vi "Position_TOTAL_R21.vi"(5 "Distance Between \nCameras  (*unit)":sgl=2.5) -> (12 "dX, dY\nLeft Cam":cluster{"X":sgl[], "Y":sgl[]}={"X"=[-5.750775, -4.1849813, -3.081379, -2.0098581, 0.0], "Y"=[7.9585915, 7.9595685, 7.960258, 7.960927, 0.0]}, 13 "Position Valid":bool=TRUE, 14 "Left Camera Real Coordinates":cluster{"X":sgl, "Y":sgl}={"X"=7.9602513, "Y"=5.592073}, 16 "dX, dY\nRight Cam":cluster{"X":sgl[], "Y":sgl[]}={"X"=[-7.3032045, -5.737411, -4.6338086, -3.5622878, -1.5524296], "Y"=[7.2714148, 7.2723923, 7.2730813, 7.273751, -0.68717635]}, 18 "Robot Coordinates":cluster{"X":sgl, "Y":sgl}={"X"=7.616663, "Y"=6.3682876}, 19 "Orietnation\n(current)":sgl=-23.843685 format="%#_13g")   [LabVIEW 2015]
uses:
  <vilib>/Analysis/coordinate.llb/2D Cartesian Coordinate Rotation (Array).vi
  <vilib>/myRIO/Common/Instrument Driver Framework/myRIO v1.0/DIO/vis/myRIO v1.0 Close DIO.vi
  <vilib>/myRIO/Common/Instrument Driver Framework/myRIO v1.0/DIO/vis/myRIO v1.0 Unreserve DIO.vi
  <vilib>/myRIO/Common/Instrument Driver Framework/myRIO v1.0/DIO/vis/myRIO v1.0 Build MUX Configuration DIO.vi
  <vilib>/myRIO/Common/Instrument Driver Framework/myRIO v1.0/Resource Manager/vis/myRIO v1.0 Unreserve Channel List.vi
  <vilib>/myRIO/Common/Instrument Driver Framework/myRIO v1.0/Resource Manager/vis/myRIO v1.0 Create Configuration List.vi
  <vilib>/myRIO/Common/Instrument Driver Framework/myRIO v1.0/Resource Manager/vis/myRIO v1.0 Unreserve Channel.vi
  <vilib>/myRIO/Common/Instrument Driver Framework/myRIO v1.0/Resource Manager/vis/myRIO v1.0 Build Mutex Name.vi
  <vilib>/Instr/_visa.llb/VISA Configure Serial Port (Instr).vi
  <vilib>/myRIO/Common/Instrument Driver Framework/myRIO v1.0/DIO/vis/myRIO v1.0 Shutdown DIO.vi
  <vilib>/Utility/error.llb/Error Cluster From Error Code.vi
  <vilib>/myRIO/Common/Instrument Driver Framework/myRIO v1.0/Resource Manager/vis/myRIO v1.0 Configure IO.vi
  <vilib>/myRIO/Common/Instrument Driver Framework/Utilities/vis/Configuration Manager.vi
  <vilib>/myRIO/Common/Instrument Driver Framework/Utilities/vis/IO Manager.vi
  <vilib>/myRIO/Common/Instrument Driver Framework/myRIO v1.0/myRIO v1.0 Close.vi
  <vilib>/Analysis/NI_AALPro.lvlib
  <vilib>/myRIO/Instrument Drivers/Onboard IO/DIO/DIO.lvlib
panel:
  out "Scale Based\nWeight":sgl format="%#_13g"
  in  "Triangle Based\nWeight":sgl=0.4 format="%#_13g"
  out "Current Cam State - R":T1(ring)=enum."Normal - 5"
  out "Current Cam State - L":T1(ring)=enum."Normal - 5"
  out "Valid Beacon Sets_":bool[](array[boolean])=[TRUE, TRUE, TRUE, TRUE, FALSE]
  in  "Distance Threshold\nRef Triangles (*unit)":sgl=30.0
  out "dA2 4":sgl=9.6935425 format="%#_13g"
  out "dA2 2":sgl=9.6935425 format="%#_13g"
  out "dA2 3":sgl=9.6935425 format="%#_13g"
  out "Beacon Scales - Left":sgl[](array[numeric])=[76.306, 116.841255, 157.35043, 195.67218, 0.0]
  out "Beacon Scales - Right":sgl[](array[numeric])=[76.306, 116.841255, 157.35043, 195.67218, 0.0]
  in  "New Orientation \nThreshold":sgl=10.0
  in  "Moving Average\nWindow Length":u8=2
  out "Current Recovery State -L":enum16{"Generic Sweep", "Recovery Search"}(ring)=enum."Recovery Search"
  out "Current Move Delta - L 2":u16
  out "Next Recovery State - Left":enum16{"Generic Sweep", "Recovery Search"}(ring)=enum."Recovery Search"
  out "Next Recovery State - Right":enum16{"Generic Sweep", "Recovery Search"}(ring)=enum."Recovery Search"
  out "Current Recovery State - Right":enum16{"Generic Sweep", "Recovery Search"}(ring)=enum."Recovery Search"
  in  "Initial Recovery State  - Right":enum16{"Generic Sweep", "Recovery Search"}(ring)=enum."Recovery Search"
  in  "Initial Recovery State - L":enum16{"Generic Sweep", "Recovery Search"}(ring)=enum."Recovery Search"
  out "Next Tracking State - Right":enum16{"Track", "Reactive Predict", ""}(ring)
  out "Current Tracking State - Right 2":enum16{"Track", "Reactive Predict", ""}(ring)
  in  "Initial Tracking State - Right":enum16{"Track", "Reactive Predict", ""}(ring)
  out "Last Track Angle - R":sgl=98.61328
  out "Next Tracking State - Left":enum16{"Track", "Reactive Predict", ""}(ring)
  in  "Initial Tracking State - Left":enum16{"Track", "Reactive Predict", ""}(ring)
  out "Current Tracking State - Left":enum16{"Track", "Reactive Predict", ""}(ring)
  in  "Timeout to \nEnable Reactive Predict":u16=5
  out "Tracking Timeout\nCount - R":i32
  in  "Tracking Timeout\nThreshold":i32=10
  out "Tracking Timeout\nCount - L":i32
  in  "Search Direction - in - Right":bool=TRUE
  out "Next Main State - Right":T2(ring)=enum."Tracking"
  in  "Recovery Search\nDirection - R":bool
  out "Recovery Mode Count in Right":i32
  out "Frames Processed\nCount - in Right":i32
  out "Recovery Search\nmove Count - Right":u16
  out "Recovery Search\nAttempt Count - Right":u16
  in  "Mounting Offset - Right":sgl=45.0
  in  "Tracking Angle - Right":sgl=98.60307
  in  "Current Servo Position\n- Right":u16
  out "New Data  Flag\nRight Servo":bool
  in  "Track Angle Valid  - Right":bool=TRUE
  out "Current Main State - Right":T2(ring)=enum."Tracking"
  in  "Initial Main State- Right":T2(ring)
  in  "Recovery Search\nDirection - L 2":bool
  in  "Max Recovery Count\n(Recovery Search) 2":u16
  in  "Max Recovery\nSearch Attempts 2":u16
  in  "Image Lock - Right 2":bool
  out "Last Track Angle - L":sgl=87.24609
  in  "Recovery Search\nDirection - L":bool=TRUE
  out "Next Main State - Left":T2(ring)=enum."Tracking"
  out "Current Move Delta - L":u16
  in  "Max Recovery Count\n(Recovery Search)":u16=10
  in  "Max Recovery\nSearch Attempts":u16=3
  out "Recovery Search\nAttempt Count - in - L":u16
  out "Recovery Search\nmove Count - in - L":u16
  in  "Image Lock - Right":bool=TRUE
  out "Recovery Mode Count - in Left":u16
  in  "Middle Beacon\nCoordinates":cluster{"X":sgl, "Y":sgl}={"X"=0.0, "Y"=2.5}
  in  "Min Num Frames\nper Search":i32=2
  in  "Wait Tick Threshold":i32=10
  out "Frames Processed\nCount - in -L":i32
  in  "Maximum Move \nServo Threshold":i16=300
  in  "Minimum Delta \nServo Threshold":i16=3
  in  "Mounting Offset - Left":sgl=-45.0
  in  "Search Step Size":u16=50
  in  "Search Direction - in - L":bool
  in  "Current Servo Position\n- Left":u16
  in  "Tracking Angle - Left":sgl=87.25689
  out "New Data  Flag\nLeft Servo":bool
  in  "Track Angle Valid - Left":bool=TRUE
  in  "Image Lock - Left":bool=TRUE
  in  "Initial Main State - Left":T2(ring)
  out "Current Main State - Left":T2(ring)=enum."Tracking"
  in  "Position Calc\nTimer":u32=100 caption="Position Calc Timer"
  in  "Fetch Input\n(mSec)":u32=20 caption="Update Camera Input\n(mSec)"
  out "Right Data\nInput Flag\n- Internal":bool=TRUE
  in  "Position Calc\nReady":bool
  out "This Servo \nAngle - Right":sgl=98.90625
  in  "Beacon Angles -R":sgl[](array[numeric])=[111.28093, 105.355774, 98.60307, 92.04714, 103.90625]
  in  "Beacon Angles - L":sgl[](array[numeric])=[101.98467, 94.59042, 87.25689, 80.30646, 91.66016]
  in  "Valid Angles -R":bool[](array[boolean])=[TRUE, TRUE, TRUE, TRUE, FALSE]
  in  "Valid Angles - L":bool[](array[boolean])=[TRUE, TRUE, TRUE, TRUE, FALSE]
  out "Left Data\nInput Flag\n- Internal":bool
  in  "Check Shared Var Timer":u32=50 caption="Main Loop\n Timer (ms)"
  out "Left_Flag 2":bool
  out "Right_Flag 2":bool
  out "Beacons Found\n- Left (Bool Array) 2":bool[](array[boolean])=[TRUE, TRUE, TRUE, TRUE, FALSE]
  out "LEFT Beacon Coord - X px (IN) 2":sgl[](array[numeric])=[76.306, 116.841255, 157.35043, 195.67218, 0.0]
  out "LEFT Beacon Position - Y px (IN) 2":sgl[](array[numeric])=[154.30304, 148.59094, 148.39949, 146.94655, 0.0]
  out "This Servo \nAngle - Left":sgl=86.66016
  in  "Compliance Slope":u8=128
  out "deltaMoveServo\n- R":i16
  out "Move Respond - R":bool
  out "Move Respond - L":bool
  out "Last Position":cluster{"X":sgl, "Y":sgl}={"X"=7.6261, "Y"=6.350474}
  out "Last Orientation":sgl=-23.876373
  in  "Distance\nBetween Beacons \n- Tolerance":sgl=0.35 format="%#_13g"
  in  "Distance\nBetween Beacons":sgl=1.0 format="%#_13g"
  out "dT":dbl=143.499
  out "Position Valid\nHistory":bool[](array[boolean])=[TRUE, FALSE, FALSE, TRUE, TRUE, FALSE, TRUE, TRUE, TRUE, TRUE, TRUE, TRUE, FALSE, TRUE, FALSE]
  out "Orientation\nHistory":sgl[](array[numeric])=[-23.876373, 0.0, 0.0, -23.938759, -24.0458, 0.0, -23.14014, -22.504314, -22.596928, -22.90728, -23.237453, -23.75214, 0.0, -23.808718, 0.0]
  out "Robot Coordinates\nHistory":cluster{sgl, sgl}[](array[cluster])=[{7.6261, 6.350474}, {0.0, 0.0}, {0.0, 0.0}, {7.63815, 6.33973}, {7.6316156, 6.322055}, {0.0, 0.0}, {7.6863523, 6.2558875}, {7.688662, 6.2228284}, {7.6736236, 6.2455945}, {7.6880507, 6.2819676}, {7.6893277, 6.3140097}, {7.668109, 6.3330927}, {0.0, 0.0}, {7.6506357, 6.3142757}, {0.0, 0.0}]
  in  "New Position \nThreshold":sgl=1.5
  out "Orientation Avgd":sgl=-23.876373
  in  "History Size":u8=15
  in  "Max Y (arena)":sgl=15.0
  in  "Max X (arena)":sgl=35.0
  in  "New Position\nWeight":sgl=0.7 format="%#_13g"
  in  "Max Std Dev (3)":sgl=0.2 format="%#_13g"
  in  "Max Std Dev (4)":sgl=0.2 format="%#_13g"
  out "Post Filtering\n- Valid Beacons":bool[](array[boolean])=[FALSE, TRUE, TRUE, TRUE, FALSE]
  out "Robot Coordinates - Avgd":cluster{"X":sgl, "Y":sgl}={"X"=7.6261, "Y"=6.350474}
  out "Real Position in Course 2":cluster{"X":dbl[], "Y":dbl[]}(graph)={"X"=[7.626100046018056], "Y"=[6.35047366782369]}
  out "Position \nLock Status":bool=TRUE
  out "Right Camera Real Coordinate":cluster{"X":sgl, "Y":sgl}={"X"=7.2730746, "Y"=7.1445026}
  out "deltaMoveServo\n- L":i16
  in  "Search Step Size\n(deg)":sgl=15.0 format="%#_13g"
  out "Beacons Found\n- Right (Bool Array)":bool[](array[boolean])=[TRUE, TRUE, TRUE, TRUE, FALSE]
  out "RIGHT Beacon Position - Y px (IN)":sgl[](array[numeric])=[153.02994, 149.48933, 150.4864, 150.33003, 0.0]
  out "RIGHT Beacon Coord - X px (IN)":sgl[](array[numeric])=[91.3685, 123.99656, 161.27843, 197.4523, 0.0]
  in  "Right Servo\nID":string="\u0001"
  in  "Servo Comm\nWait Time - (ms)":i32
  in  "Left Servo\nID":string="\u0000"
  out "dT - Comm Loop":u32=19
  in  "Servo Comm\nLoop Time (ms)":i32=20
  in  "close comms":bool
  in  "Max Read\nTx Attempts":u8=3
  in  "Max Write\nTx Attempts":u8=3
  out "Current R (10bit)":u16=696
  out "Servo Moving - R":bool
  out "Servo Moving - L":bool
  out "Current L (10bit)":u16=347
  in  "SERVO ENABLE":bool=TRUE
  out "Move Servo - L":bool
  out "Move Servo - R":bool
  in  "Servo Goal Position\n - Right":u16=695
  in  "Move Servo\nThreshold (deg)":sgl=2.0 format="%#_13g"
  in  "Servo Algorithm\nCycle Time(ms)":i32=25
  in  "Servo Goal Position\n - Left":u16=349
  in  "Current Angle\n - Left (internal)":sgl=86.66016
  in  "Current Angle\n - Right (internal)":sgl=98.90625
  in  "stop":bool
  in  "Num of Beacons (Total)":i8=5
  out "Angle to Pixel Ratios":T3={"Angle to Pixel\nRatio - Horizontal"=0.18125, "Angle to Pixel\nRatio - Vertical"=0.1875} {"Angle to Pixel\nRatio - Vertical" format="%#_13g"; "Angle to Pixel\nRatio - Horizontal" format="%#_13g"}
  in  "Cam AOV Vertical (deg)":sgl=45.0
  in  "Cam AOV Horizontal (deg)":sgl=58.0
  in  "Image Height (px)":sgl=240.0
  in  "Image Width (px)":sgl=320.0
  out "Beacon Coordinates - Left Image":T4={"Beacon Position - X px"=[76.306, 116.841255, 157.35043, 195.67218, 0.0], "Beacon Position - Y px"=[154.30304, 148.59094, 148.39949, 146.94655, 0.0]}
  out "Beacon Coordinates - Right Image":T4={"Beacon Position - X px"=[91.3685, 123.99656, 161.27843, 197.4523, 0.0], "Beacon Position - Y px"=[153.02994, 149.48933, 150.4864, 150.33003, 0.0]}
  out "Distance to LBF":sgl[](array[numeric])=[0.024284193, 0.015691843, 0.008273765, 0.028971607, 0.03291407]
  out "Local Coordinates - Calculated":cluster{sgl[], sgl[]}(graph)={[-2.0384164, -0.70265853, 0.4090246, 1.3811935, 0.0], [9.602626, 8.751521, 8.536832, 8.085801, 0.0]}
  out "Local Coordinates - Rotated":cluster{dbl[], dbl[]}(graph)={[1.5524295802029098, -5.750774735805926, -4.1849814062260675, -3.0813788557258652, -2.009858210562305, 0.0], [0.6871763361707266, 7.9585912385832795, 7.959568450875426, 7.960257859242679, 7.960927027680405, 0.0]}
  out "All Object Coordinates \n- Local - Rotated":cluster{"X":sgl[], "Y":sgl[]}={"X"=[1.5524296, -5.750775, -4.1849813, -3.081379, -2.0098581, 0.0], "Y"=[0.68717635, 7.9585915, 7.9595685, 7.960258, 7.960927, 0.0]}
  out "Local Coordinates - Normalized":cluster{sgl[], dbl[]}(graph)={[1.6977187, -2.0372734, -0.60508364, 0.4043527, 1.3844445, 0.0], [0.0, 9.605212211608887, 8.972328186035156, 8.526259422302246, 8.093157768249512, 0.0]}
  in  "Max Std Dev (5)":sgl=0.2 format="%#_13g"
  out "All Object Coordinates \n- Local":cluster{"X":sgl[], "Y":sgl[]}={"X"=[1.6977187, -2.0372734, -0.60508364, 0.4043527, 1.3844445, 0.0], "Y"=[0.0, 9.605212, 8.972328, 8.526259, 8.093158, 0.0]}
  out "LOCAL\nBeacon Coordinates\nRelative to Robot":cluster{"dX_beacon":sgl[], "dY_beacon":sgl[]}={"dX_beacon"=[-2.0384164, -0.70265853, 0.4090246, 1.3811935, 0.0], "dY_beacon"=[9.602626, 8.751521, 8.536832, 8.085801, 0.0]}
  in  "Real Beacon\n - Coordinates":cluster{"X":dbl[], "Y":dbl[]}={"X"=[0.0, 0.0, 0.0, 0.0, 0.0, 0.0], "Y"=[0.5, 1.5, 2.5, 3.5, 4.5, 0.0]}
  # "POSITION CALCULATION VARIABLES"
  # "OUTPUT VALUES"
  # "CONFIG VALUES"
  # "FILTER CONFIG VALUES"
  # "FEEDBACK INPUT VALUES"
  # "INPUT VALUES"
  # "INTERMEDIATE VALUES"
  # "IMAGE TO ANGLE VARIABLES"
  # "VISION PROCESSEING INPUTS"
  # "Use moving average for previous orientation thresholds"
  # "INPUTS"
  # "CONFIG"
  # "OUTPUT VALUES"
  # "*********************"
  # "unfiltered"
  # "NEW FILTER VALS"
  # "Inter Beacon Distance Filtering"
  # "MOVING AVERAGE\nVARIABLES"
  # "DISTANCE SOURCE WEIGHT"
  # "SERVO CONTROL VARIABLES"
  # "SERVO CONTROL VARIABLES"
  # "CONFIG"
  # "SHARED VARIABLE INPUTS"
  # "LOCAL VARIABLE INPUTS"
  # "INTERNRAL VARIABLES"
  # "SEARCH ROUTINE VARIABLES"
  # "MISC"
  # "SERVO IDs"
  # "CONTROL DELAYS"
  # "COMM LOOP DELAY"
  # "COMM PROTOCOL"
  # "SETTINGS"
  # "Make function of distance^^"
  # "**** only left side starts search\nat previously known good angle"
  # "LEFT SERVO"
  # "RIGHT SERVO"
  # "Main State Machine"
  # "Recovery State Machine"
  # "Current Track Angle Inputs"
  # "Servo Status Inputs"
  # "Main State Machine Inputs"
  # "Recovery State Machine Inputs"
  # "Current Track Angle Inputs"
  # "Servo Status Inputs"
  # "Recovery State Machine Feedback"
  # "Tracking State Machine Inputs"
  # "Tracking State Machine Inputs"
  # "NOTE: Must be 1 bigger than amount of beacons"
  # "NOTE: Must be 1 bigger than amount of beacons"
types:
  T1 = enum16{"Sub - 2", "Sub - 3", "Sub - 4", "Normal - 5"}
  T2 = enum16{"Start Up Search", "Tracking", "Recovery Mode", ""}
  T3 = cluster{"Angle to Pixel\nRatio - Horizontal":sgl, "Angle to Pixel\nRatio - Vertical":sgl}
  T4 = cluster{"Beacon Position - X px":sgl[], "Beacon Position - Y px":sgl[]}
  T5 = cluster{"Tracking Coordinates":cluster{"X":dbl, "Y":dbl}, "Current Valid":bool, "Current State - Out":enum16{"Sub - 2", "Sub - 3", "Sub - 4", "Normal - 5"}}
  T6 = cluster{"Array of Double":dbl[], "Array of Double":dbl[]}
  T7 = typedef "DIO.lvlib/DIO Reference.ctl" = cluster{"myRIO Reference":T8, "DIO Channels List":T12}
  T8 = typedef "myRIO Generic Hardware Reference.ctl" = cluster{"myRIO Model":T9, "myRIO Hardware Reference":T10}
  T9 = typedef "Hardware Version Enum.ctl" = enum16{"Unknown", "myRIO-1900", "myRIO-1950", "roboRIO"}
  T10 = typedef "myRIO v1.0 Reference.ctl" = cluster{"Generic FPGA Reference":T11, "Allow multiple opens":bool}
  T11 = typedef "Generic FPGA Reference.ctl" = refnum<k20>
  T12 = typedef "DIO Channels List.ctl" = T13[]
  T13 = typedef "DIO Channels Enum.ctl" = enum16{"Not Connected", "C/DIO0", "C/DIO1", "C/DIO2", "C/DIO3", "C/DIO4", "C/DIO5", "C/DIO6", "C/DIO7", "A/DIO0", "A/DIO1", "A/DIO2", "A/DIO3", "A/DIO4", "A/DIO5", "A/DIO6", "A/DIO7", "A/DIO8", "A/DIO9", "A/DIO10", "A/DIO11", "A/DIO12", "A/DIO13", "A/DIO14", "A/DIO15", "B/DIO0", "B/DIO1", "B/DIO2", "B/DIO3", "B/DIO4", "B/DIO5", "B/DIO6", "B/DIO7", "B/DIO8", "B/DIO9", "B/DIO10", "B/DIO11", "B/DIO12", "B/DIO13", "B/DIO14", "B/DIO15", "LED0", "LED1", "LED2", "LED3", "Button0", "DIO/DIO0", "DIO/DIO1", "DIO/DIO2", "DIO/DIO3", "DIO/DIO4", "DIO/DIO5", "DIO/DIO6", "DIO/DIO7", "DIO/DIO8", "DIO/DIO9", "SPI/CS0", "SPI/CS1", "SPI/CS2", "SPI/CS3", "LED RADIO (Green)", "LED RADIO (Red)", "LED COMM (Green)", "LED COMM (Red)", "LED MODE (Green)", "LED MODE (Red)"}
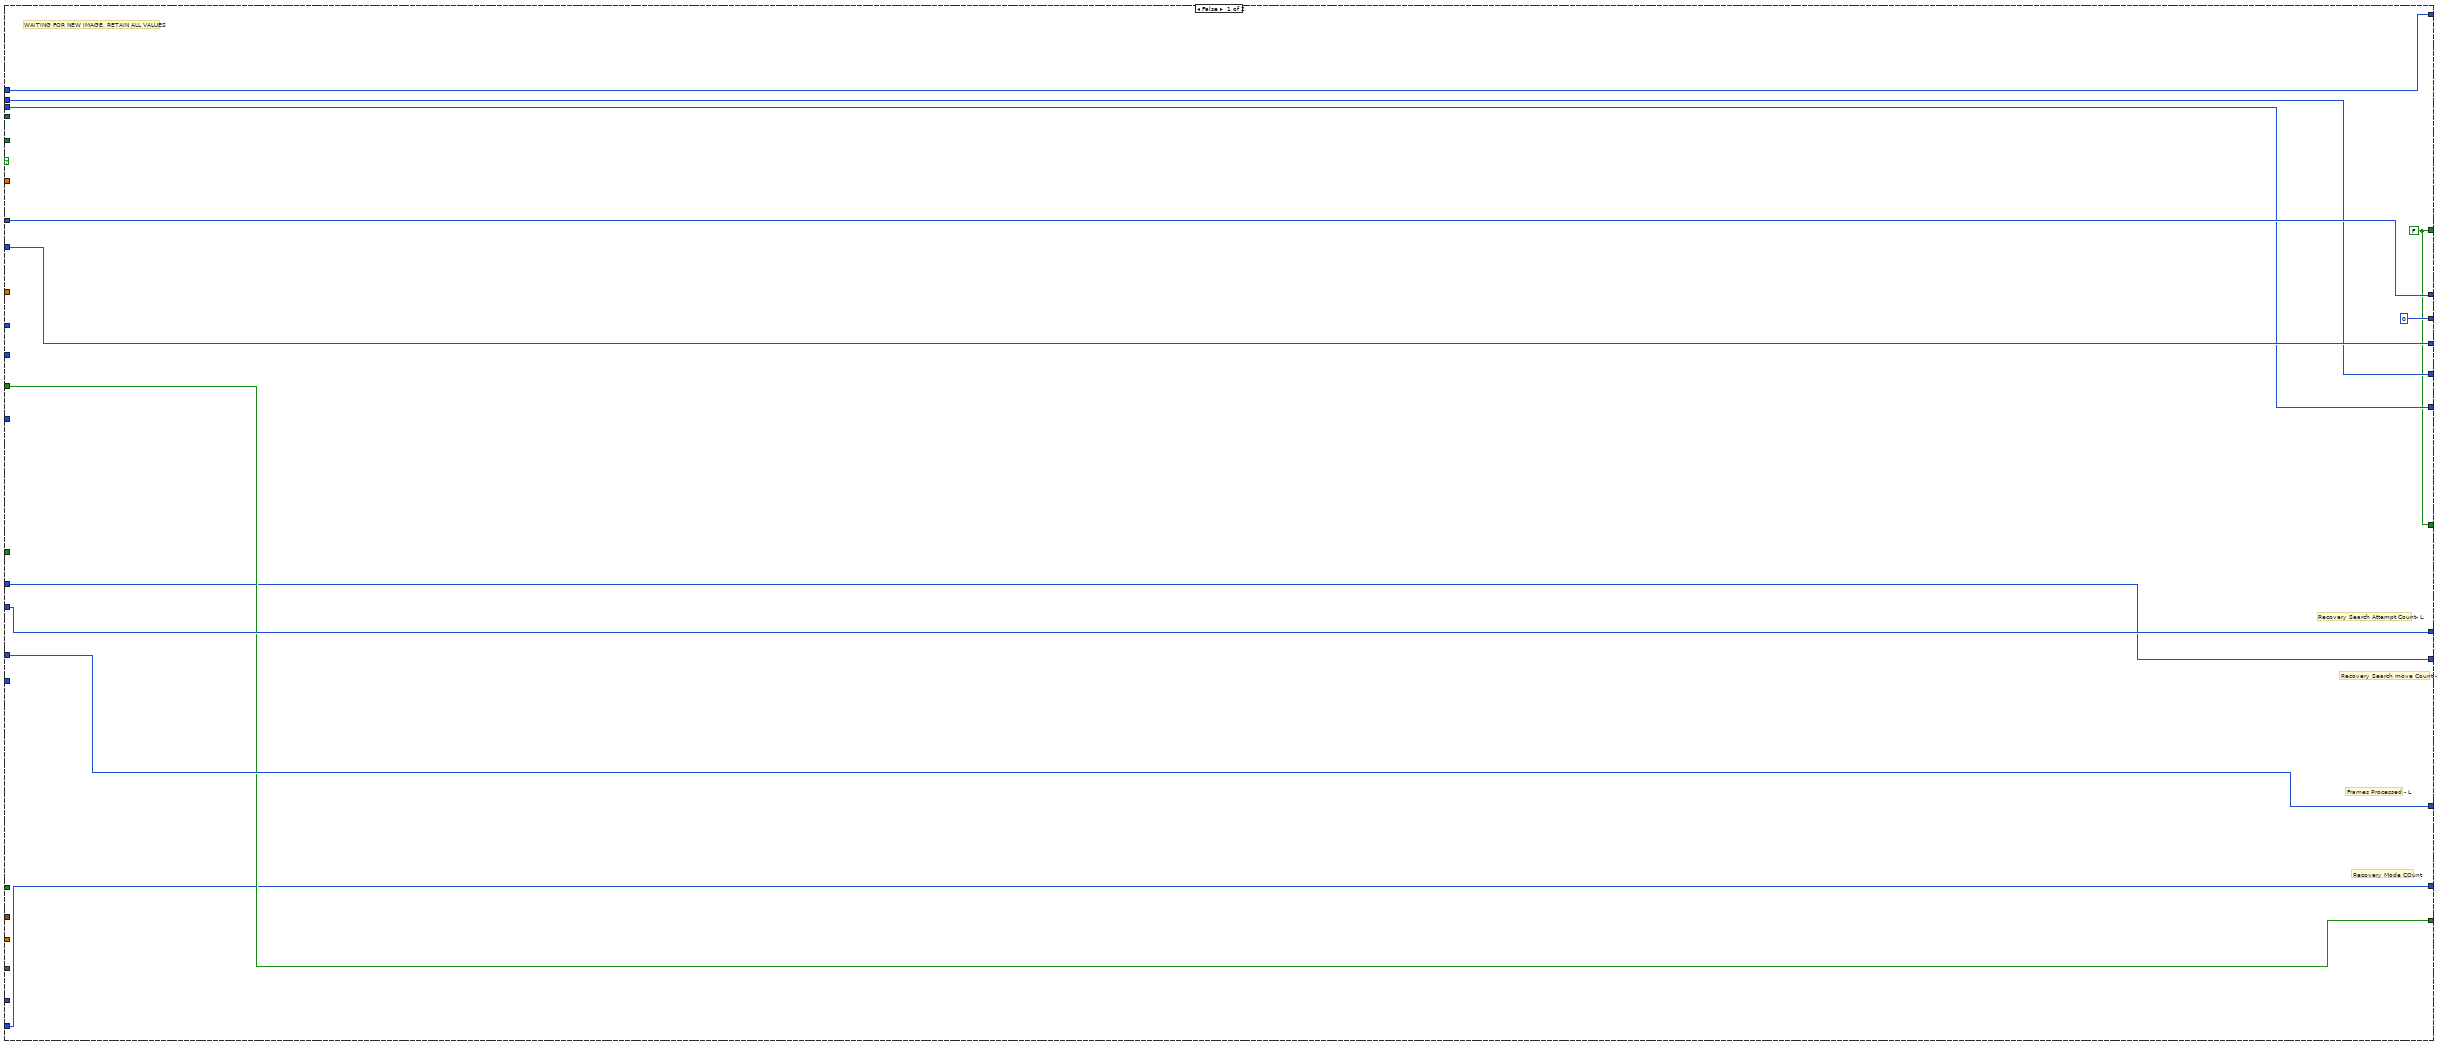
[diagram p2: hidden frame]
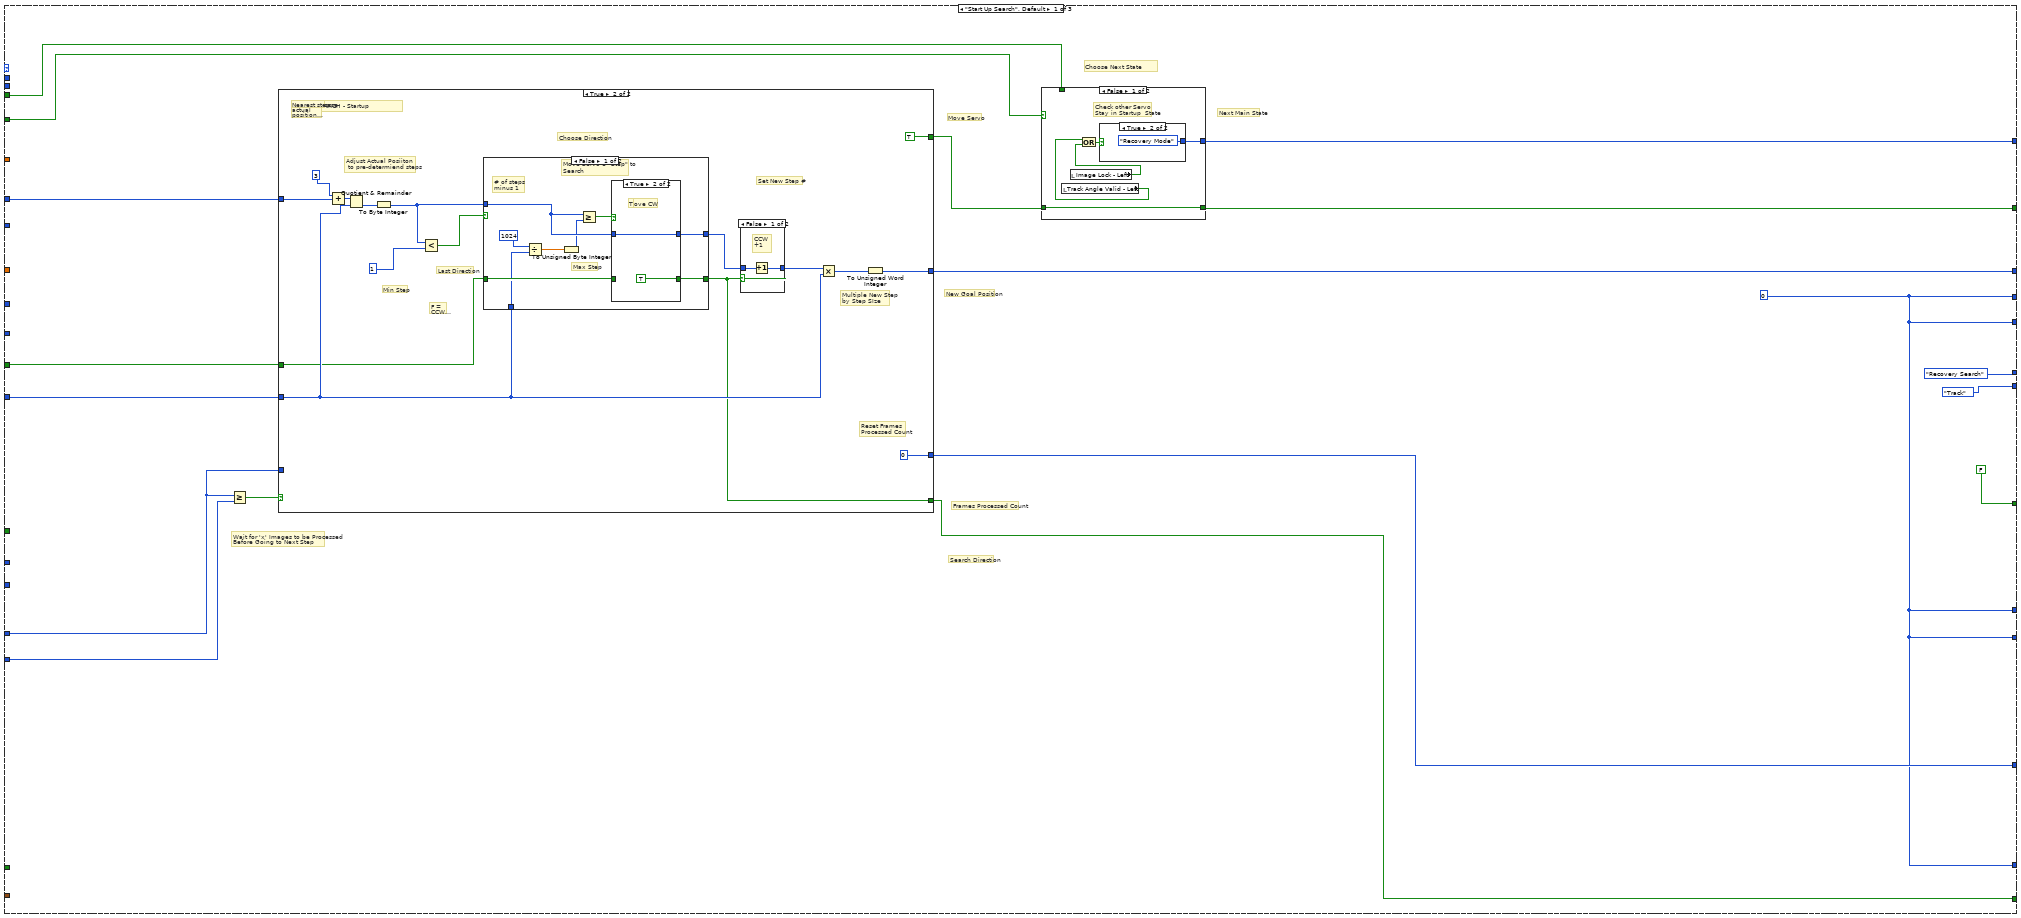
[diagram p3: hidden frame]
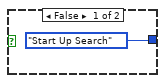
[diagram p4: hidden frame]
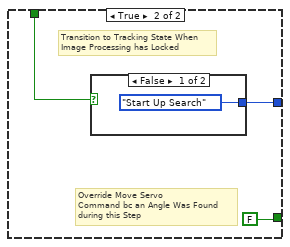
[diagram p5: hidden frame]
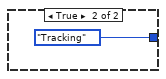
[diagram p6: hidden frame]
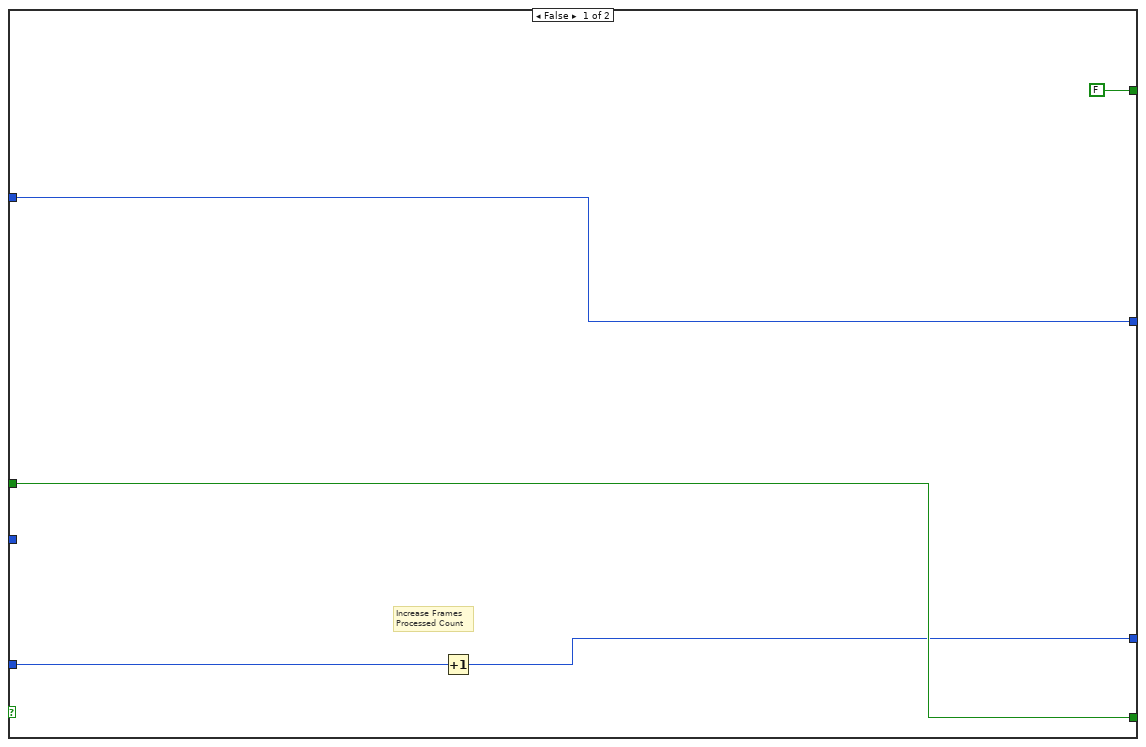
[diagram p7: hidden frame]
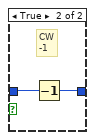
[diagram p8: hidden frame]
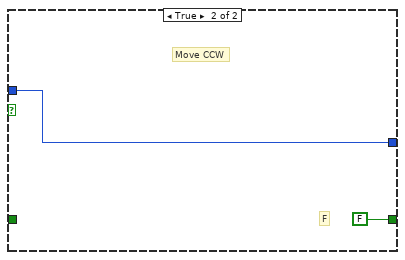
[diagram p10: hidden frame]
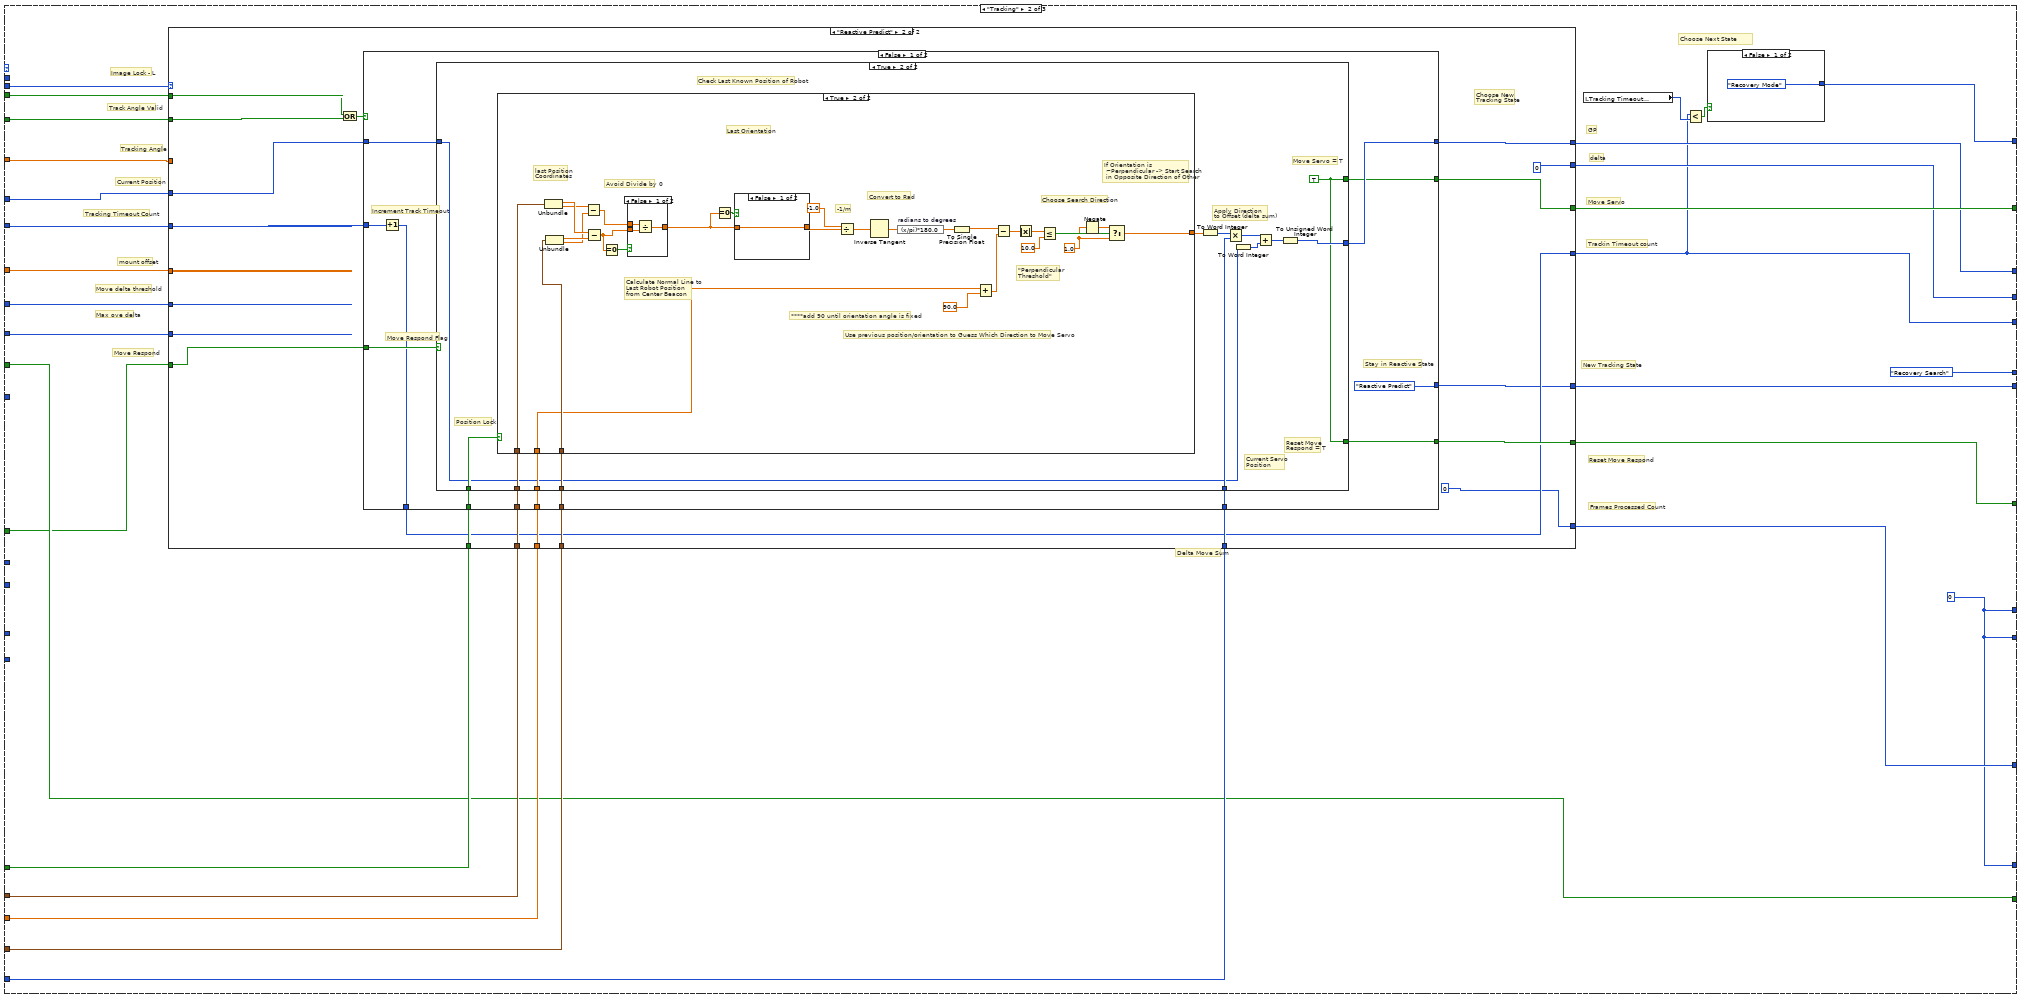
[diagram p11: hidden frame]
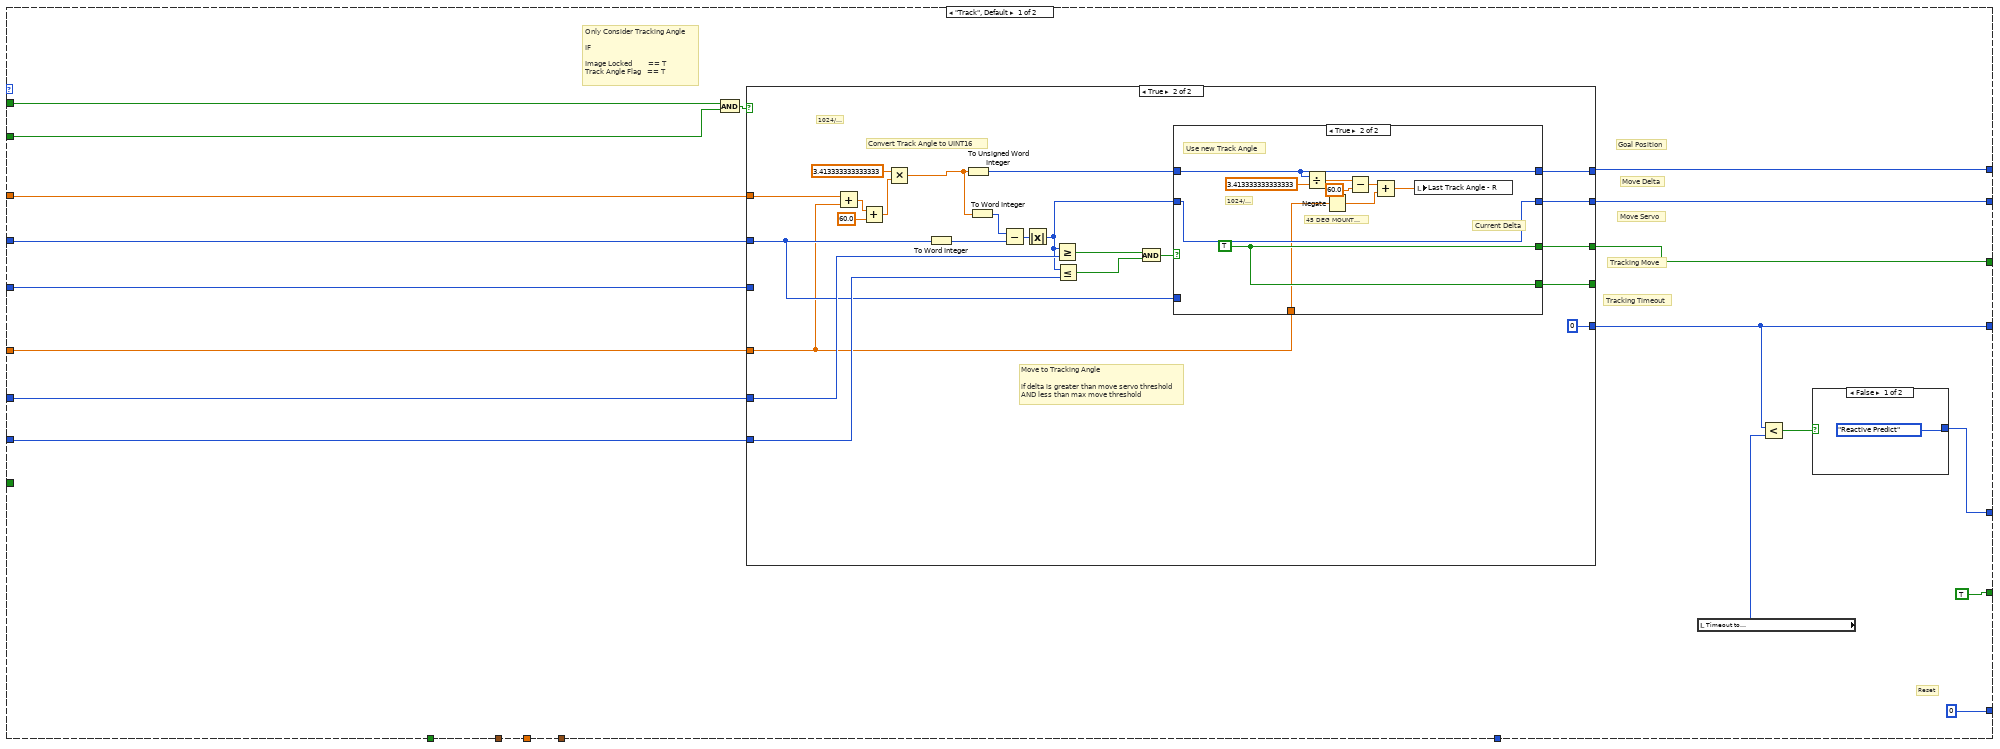
[diagram p12: hidden frame]
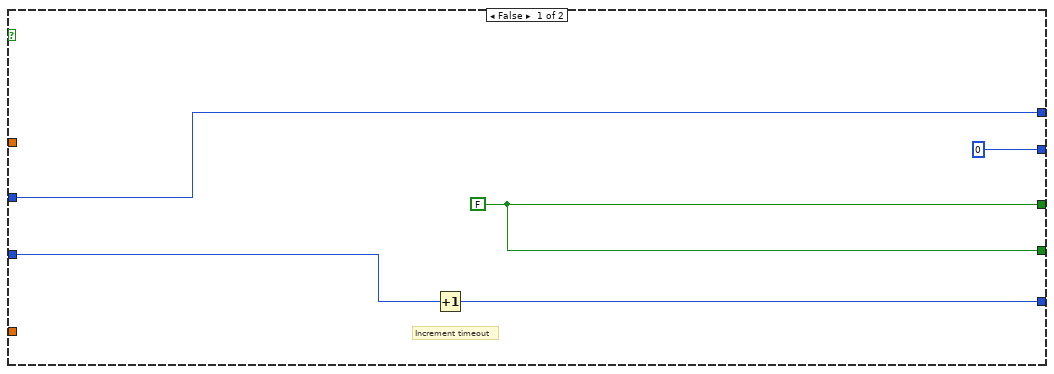
[diagram p13: hidden frame]
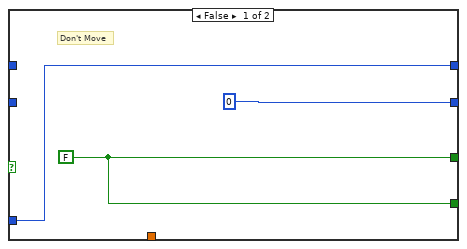
[diagram p14: hidden frame]
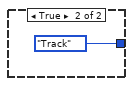
[diagram p15: hidden frame]
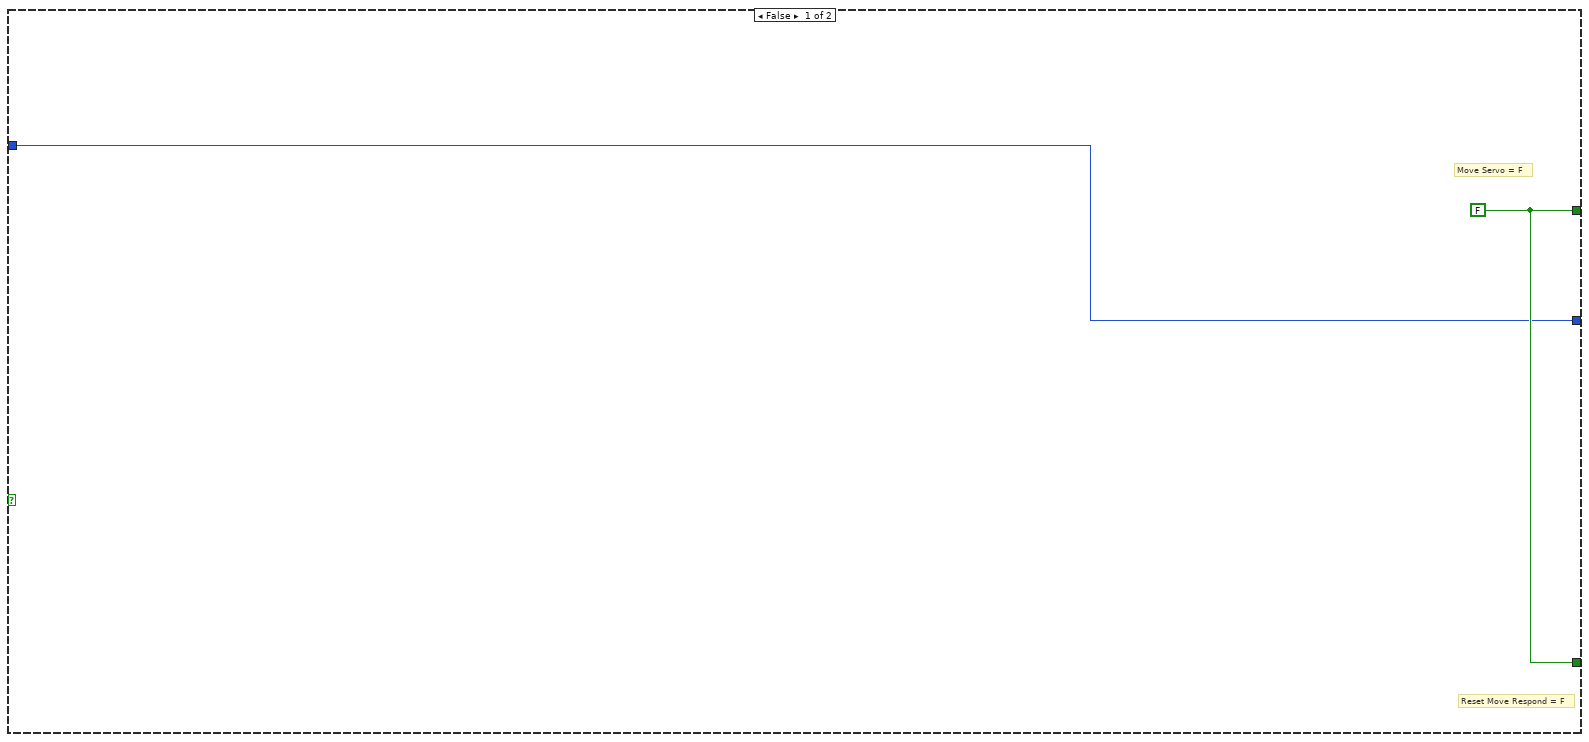
[diagram p16: hidden frame]
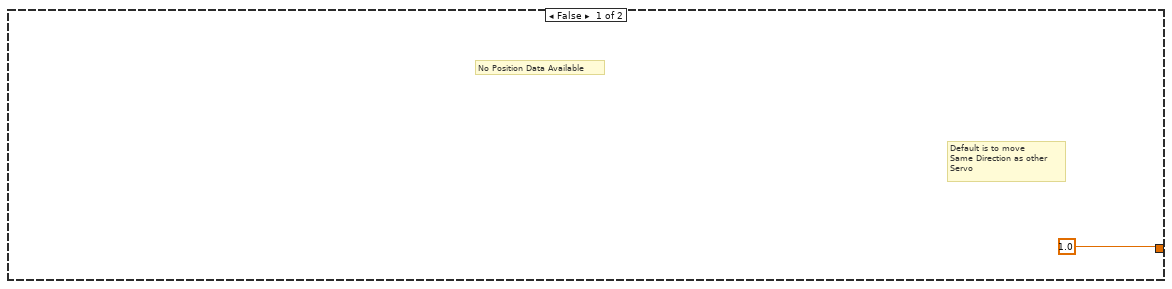
[diagram p17: hidden frame]
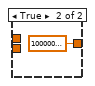
[diagram p18: hidden frame]
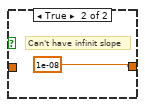
[diagram p19: hidden frame]
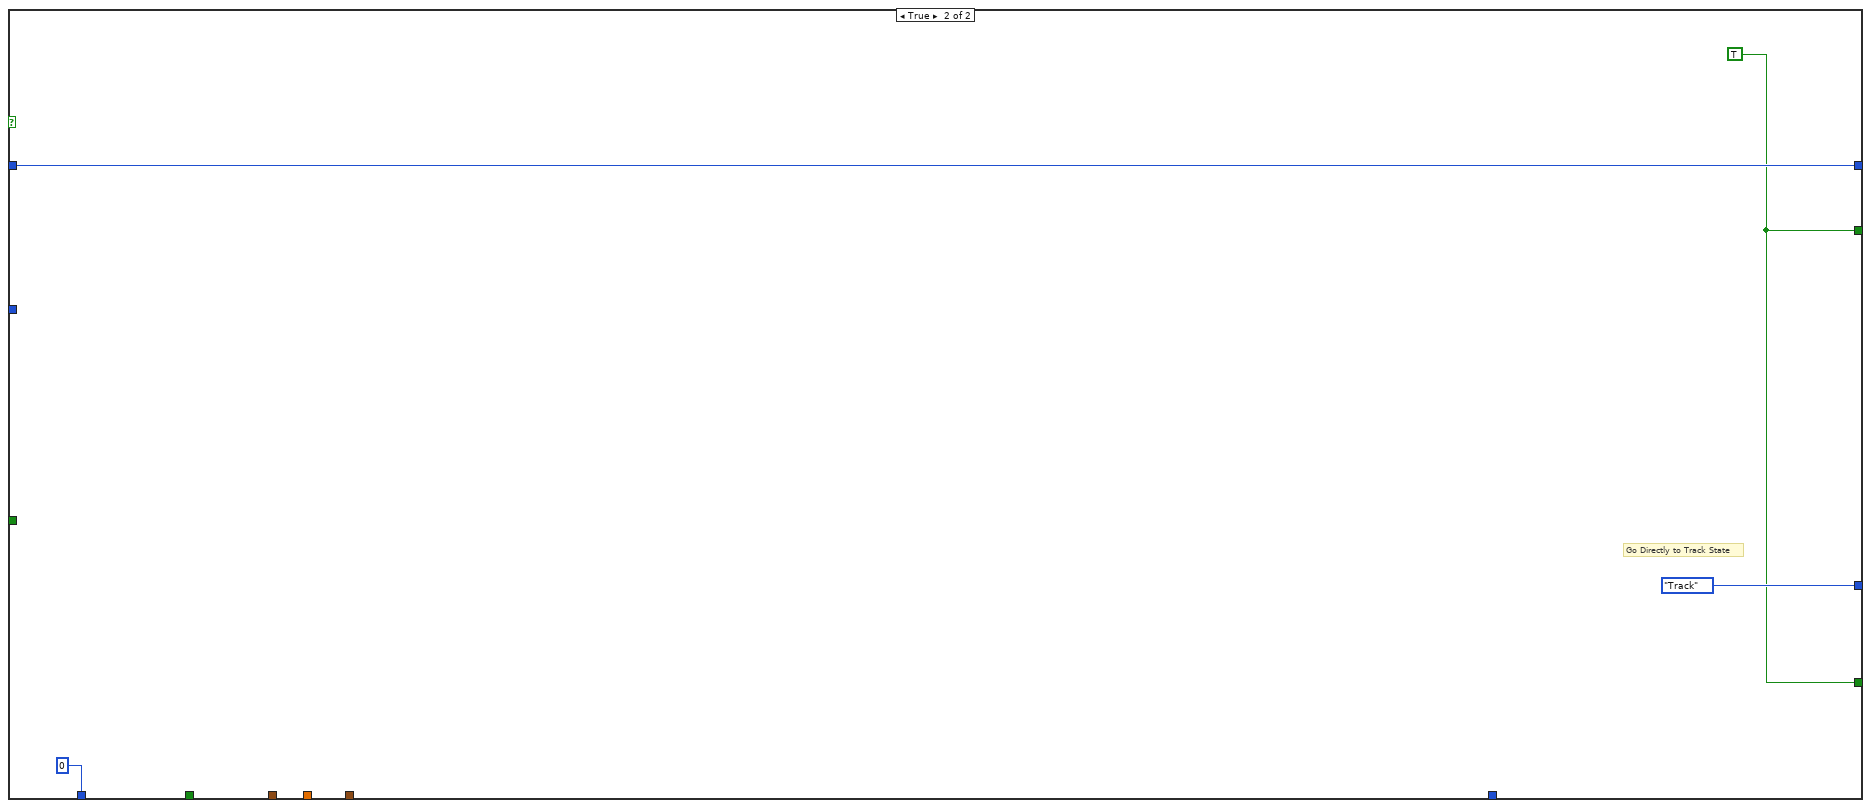
[diagram p20: hidden frame]
diagram:
  (unwired) enum16{"Generic Sweep", "Recovery Search"}."Recovery Search"
  w12 = 0 ("Frames Processed\nCount - in")
  w13 = 0 ("Frames Processed\nCount - in")
  w2 = FALSE
  w34 = sgl 0.0
  # "SERVO CONTROL FLAGS"
  # "***"
  # "Next Tracking State"
  # "Tracking Timeout Count"
  # "Search Direction - L"
  # "Next Recovery State"
  # "Move Respond"
  # "Recovery Mode Count - L"
  # "Delta Move Sum - L"
  # "Wait Tick Count - L"
  # "Frames Processed - L"
  # "Recovery Search move Count - L"
  # "Recovery Search Attempt Count- L"
  # "Next Main State"
  # "Search Direction - L"
  # "Next Recovery State"
  # "INPUTS - Local vars"
  # "Recovery Mode Count - L"
  # "Delta Move Sum - L"
  # "Frames Processed\nLeft"
  # "Move Respond - R"
  # "Initial Search Direction\n- Right"
  # "Move Respond"
  # "Recovery Mode Count - L"
  # "Delta Move Sum - L"
  # "Wait Tick Count - L"
  # "Frames Processed - L"
  # "Recovery Search move Count - L"
  # "Recovery Search Attempt Count- L"
  # "Next Main State"
  # "Settings -- Update in a slow loop"
  # "Recovery Mode Count - L"
  # "Delta Move Sum - L"
  # "Frames Processed\nLeft"
  # "Move Respond - L"
  # "Replace these with\nconstants"
  # "Initial Search Direction\n- Left"
  # "Read Inputs when Available"
  # "# of Physical Beacons"
  # "Right Data Internal Falg"
  # "Left Data Internal Falg"
  # "Initialize Shift Arrays"
  # "Robot Position (cluster)\nShift Array"
  # "Robot Position (cluster)\nShift Array"
  # "Position Valid Shift Array"
  # "Orientation Shift Array"
  # "Position Valid Shift Array"
  # "Orientation Shift Array"
  # "Servo Communication (to Servo- UART))"
  # "Internal Local Variables"
  # "Servo Control Logic"
  # "Local Variables"
  # "Images to Robot Position Calculation Process"
  # "SERVO MOTOR CONTROL"
  # "SERVO MOTOR CONTROL"
  n1 = Divide(x="Cam AOV Horizontal (deg)", y="Image Width (px)") -> (x/y=w25:sgl)
  n2 = Divide(x="Cam AOV Vertical (deg)", y="Image Height (px)") -> (x/y=w26:sgl)
  n3 = Bundle(w25, w26) -> (w20:cluster{sgl, sgl})  [unwired: 1 in]
  "Angle to Pixel Ratios" <- w20
  n4 = disable-structure shown="Disabled" {
    frame Disabled {
      # "Always Read Incoming Flags & Store"
      n5 = while {
        tunnel: "Check Shared Var Timer" -> [w46]
        stop <- FALSE stop-if-true
        n6 = shared-variable "myRIO-1900\\Lib1.lvlib\\RIGHT_FLAG"() -> (→"Right_Flag 2":bool)  [unwired: 1 in, 1 out]
        n7 = shared-variable "myRIO-1900\\Lib1.lvlib\\Left_Flag"() -> (→"Left_Flag 2":bool)  [unwired: 1 in, 1 out]
        n8 = call "Wait8"("Count(mSec)"=w46) -> ()  [unwired: 1 out]
      }
    }
    frame Enabled {
    }
  }
  n9 = while {
    shift-right: [w55] -> _
    shift-left: w2 -> [w60]
    shift-right: [w54] -> _
    shift-left: w2 -> [w58]
    tunnel: w20 -> [w56]
    tunnel: "Num of Beacons (Total)" -> [w57]
    stop <- FALSE stop-if-true
    # "Wait for Both Internal Flags"
    n10 = call "Wait6"("Count(mSec)"="Fetch Input\n(mSec)") -> ()  [unwired: 1 out]
    n11 = shared-variable "RT myRIO Target - Overlord\\Localization_Variables_r0.lvlib\\RIGHT_FLAG"() -> (w51:bool)  [unwired: 1 in, 1 out]
    n12 = shared-variable "RT myRIO Target - Overlord\\Localization_Variables_r0.lvlib\\Left_Flag"() -> (w52:bool)  [unwired: 1 in, 1 out]
    n13 = case shown="True" w51 {
      tunnel: w57 -> [_ w79]
      tunnel: w56 -> [_ w77]
      tunnel: [w61 w67] -> w49
      tunnel: w58 -> [w61 _]
      frame False {
        # "Don't Update Servo Position\nbc we're waiting on new Data to\ncome in and the servo position\nwas set at the previous set of data"
      }
      frame True {
        w67 = TRUE
        # "Store Values"
        # "Raise Internal Flag"
        # "If New Data Available"
        # "From Shift Reg"
        # "Perforrm Indivudual Angle Calculation"
        # "Pull Down Individual Flag"
        n14 = shared-variable "RT myRIO Target - Overlord\\Localization_Variables_r0.lvlib\\RIGHT_BEACON_X_array"() -> (w73:dbl[])  [unwired: 1 in, 1 out]
        "RIGHT Beacon Coord - X px (IN)" <- w73
        n15 = shared-variable "RT myRIO Target - Overlord\\Localization_Variables_r0.lvlib\\Image Lock - R"() -> (w68:bool)  [unwired: 1 in, 1 out]
        n16 = shared-variable "RT myRIO Target - Overlord\\Localization_Variables_r0.lvlib\\RIGHT_BEACON_Scales"() -> (→"Beacon Scales - Right":sgl[])  [unwired: 1 in, 1 out]
        n17 = shared-variable "RT myRIO Target - Overlord\\Localization_Variables_r0.lvlib\\Info - Right"() -> (w65:T5)  [unwired: 1 in, 1 out]
        n18 = shared-variable "RT myRIO Target - Overlord\\Localization_Variables_r0.lvlib\\RIGHT_BEACON_Y_array"() -> (w72:dbl[])  [unwired: 1 in, 1 out]
        "RIGHT Beacon Position - Y px (IN)" <- w72
        n19 = shared-variable "RT myRIO Target - Overlord\\Localization_Variables_r0.lvlib\\RIGHT_BEACON_BOOL_array"() -> (w71:bool[])  [unwired: 1 in, 1 out]
        "Beacons Found\n- Right (Bool Array)" <- w71
        n20 = Unbundle By Name(w65) -> ("Tracking Coordinates"=w64:cluster{"X":dbl, "Y":dbl}, "Current Valid"=w63:bool, "Current State - Out"=→"Current Cam State - R":T1)
        n21 = local write "Image Lock - Right"(w68) -> ()
        n22 = Bundle("Array of Double"=w73, "Array of Double"=w72) -> (w70:T6)  [unwired: 1 in]
        "Beacon Coordinates - Right Image" <- w70
        n23 = shared-variable "RT myRIO Target - Overlord\\Localization_Variables_r0.lvlib\\Right Servo Angle_Image"() -> (w69:dbl)  [unwired: 1 in, 1 out]
        "This Servo \nAngle - Right" <- w69
        n24 = shared-variable "RT myRIO Target - Overlord\\Localization_Variables_r0.lvlib\\RIGHT_FLAG"(FALSE) -> ()  [unwired: 1 in, 1 out]
        n25 = feedback #1() -> (w81:sgl[])  [unwired: 1 in]
        n26 = feedback #2() -> (w80:bool[])  [unwired: 1 in]
        n27 = call "Angle Calc_Individual Process R4.vi"("Angle to Pixel Ratios"=w77, "Previous Angles"=w81, "Num of Beacons"=w79, "Beacon Coordinates - Image"=w70, "Current Servo Angle"=w69, "Beacons Found (Bool Array)"=w71, "Previous Valid Angles"=w80, "Tracking Coordinates"=w64) -> ("Servo Goal Angle"=w76:sgl, "Valid Beacons (Bool Array)\nPosition Calc"=w75:bool[], "Angle Of Beacons \nRelative to Robot"=w74:sgl[])  [unwired: 4 in, 1 out]
        n28 = feedback-in #1(w74) -> ()
        n29 = feedback-in #2(w75) -> ()
        n30 = local write "Beacon Angles -R"(w74) -> ()
        n31 = local write "Tracking Angle - Right"(w76) -> ()
        n32 = local write "Valid Angles -R"(w75) -> ()
        n33 = local write "Track Angle Valid  - Right"(w63) -> ()
        n34 = local write "New Data  Flag\nRight Servo"(w67) -> ()
      }
    }
    "Right Data\nInput Flag\n- Internal" <- w49
    n35 = case shown="True" w52 {
      tunnel: [w82 w88] -> w48
      tunnel: w60 -> [w82 _]
      tunnel: w56 -> [_ w92]
      tunnel: w57 -> [_ w91]
      frame False {
        # "Don't Update Servo Position\nbc we're waiting on new Data to\ncome in and the servo position\nwas set at the previous set of data"
      }
      frame True {
        w88 = TRUE
        # "Store Values"
        # "Raise Internal Flag"
        # "If New Data Available"
        # "Perforrm Indivudual Angle Calculation"
        # "Pull Down Individual Flag"
        n36 = shared-variable ".\\Localization_Variables_r0.lvlib\\LEFT_BEACON_X_array"() -> (w98:dbl[])  [unwired: 1 in, 1 out]
        "LEFT Beacon Coord - X px (IN) 2" <- w98
        n37 = shared-variable "RT myRIO Target - Overlord\\Localization_Variables_r0.lvlib\\LEFT_BEACON_Scales"() -> (→"Beacon Scales - Left":sgl[])  [unwired: 1 in, 1 out]
        n38 = shared-variable "RT myRIO Target - Overlord\\Localization_Variables_r0.lvlib\\LEFT_BEACON_Y_array"() -> (w99:dbl[])  [unwired: 1 in, 1 out]
        "LEFT Beacon Position - Y px (IN) 2" <- w99
        n39 = shared-variable "RT myRIO Target - Overlord\\Localization_Variables_r0.lvlib\\LEFT_BEACON_BOOL_array"() -> (w100:bool[])  [unwired: 1 in, 1 out]
        "Beacons Found\n- Left (Bool Array) 2" <- w100
        n40 = shared-variable "RT myRIO Target - Overlord\\Localization_Variables_r0.lvlib\\Image Lock - L"() -> (w89:bool)  [unwired: 1 in, 1 out]
        n41 = shared-variable "RT myRIO Target - Overlord\\Localization_Variables_r0.lvlib\\Info - Left"() -> (w86:T5)  [unwired: 1 in, 1 out]
        n42 = Unbundle By Name(w86) -> ("Tracking Coordinates"=w85:cluster{"X":dbl, "Y":dbl}, "Current Valid"=w84:bool, "Current State - Out"=→"Current Cam State - L":T1)
        n43 = local write "Image Lock - Left"(w89) -> ()
        n44 = Bundle("Array of Double"=w98, "Array of Double"=w99) -> (w96:T6)  [unwired: 1 in]
        "Beacon Coordinates - Left Image" <- w96
        n45 = shared-variable "RT myRIO Target - Overlord\\Localization_Variables_r0.lvlib\\Left Servo Angle_Image"() -> (w90:dbl)  [unwired: 1 in, 1 out]
        "This Servo \nAngle - Left" <- w90
        n46 = shared-variable "RT myRIO Target - Overlord\\Localization_Variables_r0.lvlib\\Left_Flag"(FALSE) -> ()  [unwired: 1 in, 1 out]
        n47 = feedback #3() -> (w102:sgl[])  [unwired: 1 in]
        n48 = feedback #4() -> (w101:bool[])  [unwired: 1 in]
        n49 = call "Angle Calc_Individual Process R4.vi"("Angle to Pixel Ratios"=w92, "Previous Angles"=w102, "Num of Beacons"=w91, "Beacon Coordinates - Image"=w96, "Current Servo Angle"=w90, "Beacons Found (Bool Array)"=w100, "Previous Valid Angles"=w101, "Tracking Coordinates"=w85) -> ("Servo Goal Angle"=w95:sgl, "Valid Beacons (Bool Array)\nPosition Calc"=w94:bool[], "Angle Of Beacons \nRelative to Robot"=w93:sgl[])  [unwired: 4 in, 1 out]
        n50 = feedback-in #3(w93) -> ()
        n51 = feedback-in #4(w94) -> ()
        n52 = local write "Beacon Angles - L"(w93) -> ()
        n53 = local write "Valid Angles - L"(w94) -> ()
        n54 = local write "Tracking Angle - Left"(w95) -> ()
        n55 = local write "Track Angle Valid - Left"(w84) -> ()
        n56 = local write "New Data  Flag\nLeft Servo"(w88) -> ()
      }
    }
    "Left Data\nInput Flag\n- Internal" <- w48
    n57 = And(x=w48, y=w49) -> (x .and. y?=w59:bool)
    n58 = case shown="True" w59 {
      selector: w59 -> [_ w105]
      tunnel: w48 -> [w104 _]
      tunnel: [w104 w106] -> w55
      tunnel: [w103 w106] -> w54
      tunnel: w49 -> [w103 _]
      frame False {
      }
      frame True {
        w106 = FALSE
        # "Reset Internal Data Flags"
        # "Position Data\nReady Enabled"
        n59 = local write "Position Calc\nReady"(w105) -> ()
      }
    }
  }
  n60 = Bundle(w34, w34) -> (w37:cluster{sgl, sgl})  [unwired: 1 in]
  n61 = Initialize Array(w34, "History Size") -> (w32:sgl[])
  n62 = Initialize Array(w37, "History Size") -> (w33:cluster{sgl, sgl}[])
  n63 = Initialize Array(FALSE, "History Size") -> (w31:bool[])
  n64 = call "Tick Count4"() -> ("Tick Count(uSec)"=w30:u32)
  n65 = while {
    shift-right: [w117] -> _
    shift-left: w32 -> [w114]
    shift-right: [w116] -> _
    shift-left: w31 -> [w115]
    shift-right: [w118] -> _
    shift-left: w33 -> [w109]
    shift-right: [w110] -> _
    shift-left: w30 -> [w111]
    stop <- "stop" stop-if-true
    n66 = call "Wait5"("Count(mSec)"="Position Calc\nTimer") -> ()  [unwired: 1 out]
    n67 = case shown="True" "Position Calc\nReady" {
      selector: "Position Calc\nReady" -> [_ w179]
      tunnel: w109 -> [_ w204]
      tunnel: w109 -> [w127 w197]
      tunnel: w114 -> [w129 w196]
      tunnel: w115 -> [w128 w195]
      tunnel: [w129 w203] -> w117
      tunnel: [w128 w201] -> w116
      tunnel: [w127 w202] -> w118
      tunnel: w115 -> [_ w194]
      tunnel: w114 -> [_ w193]
      tunnel: [w126 w186] -> w112
      tunnel: w111 -> [_ w186]
      tunnel: [FALSE TRUE] -> w113
      tunnel: w109 -> [_ w181]
      frame False {
        n68 = call "Tick Count5"() -> ("Tick Count(uSec)"=w126:u32)
      }
      frame True {
        # "dY"
        # "dX"
        # "Valid"
        # "Find Local Coordinates"
        # "Valid COunt"
        # "Make sure 2+ Data Sets are Still available"
        # "Check 1st element\nwith rest of elements"
        # "Make Sure all Pointed \nIn Same Direction"
        # "For Each Valid Beacon\nCalculate Distance from Each Camera to Each Beacon"
        # "Find Common Beacons\nAmong Cameras"
        # "Currently will only\ncalculate position if 2+ \nbeacons are available \nfrom both cameras"
        # "System is in Normal (long range) State"
        # "Average Both Data Sets"
        # "Estimate Distance for each Available Beacon Angle\nPER Camera, indivduallly"
        # "At least 2+ Avaialbe"
        # "CALCULATE AVERAGE ORIENTATION"
        # "Update Outputs\nif Current Calc is Invalid\n(shouldn't matter)"
        # "Estimate Orienation Based on Previous Position"
        # "****# of previous in history that must be true\nin order for position to be considered \"locked\""
        # "New Position is Valid if both \nOrientation and Positions\nis within range of previous"
        # "Robot Position\n Shift Array"
        # "Position Valid Shift Array"
        # "Orientation Shift Array"
        # "Orientation Value"
        # "Shift & Insert Current Position Valid"
        # "Position Valid\n(orientation)"
        # "Position Valid\n(position)"
        # "Update Shift Registers"
        # "Shift & Insert Current Calculated Orientation"
        # "Shift & Insert Current Robot Position"
        # "UPDATE FINAL OUTPUT\n VALUES"
        n69 = local read "Num of Beacons (Total)"() -> (w162:i8)
        n70 = Not(x=w179) -> (.not. x?=w180:bool)
        n71 = local write "Position Calc\nReady"(w180) -> ()
        n72 = disable-structure shown="Disabled" {
          frame Disabled {
            w205 = T1."Normal - 5" ("Initial State")
            # "***********do for both"
            # "sTATE"
            n73 = local read "Current Cam State - L"() -> (w209:T1)
            n74 = local read "Current Cam State - R"() -> (w208:T1)
            n75 = Equal?(x=w209, y=w205) -> (x = y?=w207:bool)
            n76 = Equal?(x=w208, y=w205) -> (x = y?=w206:bool)
            n77 = And(x=w207, y=w206) -> ()  [unwired: 1 out]
          }
          frame Enabled {
          }
        }
        n78 = local read "Beacon Scales - Left"() -> (w168:sgl[])
        n79 = local read "Beacon Scales - Right"() -> (w165:sgl[])
        n80 = for {
          N: w162 -> [_]
          tunnel: "Valid Angles - L" -> [w338] mode=indexing
          tunnel: "Beacon Angles - L" -> [w347] mode=indexing
          tunnel: w168 -> [w348] mode=indexing
          tunnel: "Valid Angles -R" -> [w337] mode=indexing
          tunnel: "Beacon Angles -R" -> [w346] mode=indexing
          tunnel: w165 -> [w345] mode=indexing
          tunnel: "Distance Between \nCameras  (*unit)" -> [w344]
          tunnel: [w336] -> w159 mode=indexing
          tunnel: [w335] -> w158 mode=indexing
          tunnel: [w334] -> w160 mode=indexing
          # "dY"
          # "dX"
          # "Valid"
          # "If Both Cameras are using Same Beacon Data,\nAverage the 2 independently esitmated positions"
          # "dY"
          # "dX"
          # "dY"
          # "dX"
          n81 = case shown="True" w338 {
            tunnel: w347 -> [_ w425]
            tunnel: [w412 w416] -> w342
            tunnel: [w412 w417] -> w341
            tunnel: w348 -> [_ w415]
            frame False {
              w412 = sgl 0.0
              # "Current Data Set Was Not Valid\nFill with 0\nWill not be used later"
            }
            frame True {
              # "Estimate Distance"
              # "Negate dX if A2>90"
              # "Find LOCAL Coordinate of Each Beacon"
              # "Current - Valid Data Set"
              n82 = call "Scaling and Mapping"("Signals"=w415) -> ("Scaled Signals"=w414:dynamicdata)  [unwired: 9 in, 1 out]
              n83 = To Single Precision Float(number=w414) -> (single precision float=w413:sgl)
              n84 = Less?(x=w425, y=sgl 90.0) -> (x < y?=w427:bool)
              n85 = case shown="False" w427 {
                tunnel: w425 -> [w434 w436]
                tunnel: [w432 w437] -> w424
                tunnel: [FALSE TRUE] -> w419
                frame False {
                  # "Negative Y"
                  # "A2 is > 90"
                  n86 = Subtract(x=w434, y=sgl 90.0) -> (x-y=w432:sgl)
                }
                frame True {
                  # "Positive Y"
                  # "A2 is < 90"
                  n87 = Subtract(x=sgl 90.0, y=w436) -> (x-y=w437:sgl)
                }
              }
              "dA2 2" <- w424
              n88 = expression code="(x/180.0)*pi" "degrees to radians"(w424) -> (w422:sgl)
              n89 = expression code="(x/180.0)*pi" "degrees to radians"(w424) -> (w423:sgl)
              n90 = Cosine(x=w422) -> (cos(x)=w420:sgl)
              n91 = Sine(x=w423) -> (sin(x)=w421:sgl)
              n92 = Multiply(x=w413, y=w420) -> (x*y=w417:sgl)
              n93 = Multiply(x=w413, y=w421) -> (x*y=w418:sgl)
              n94 = case shown="True" w419 {
                tunnel: w418 -> [w429 w430]
                tunnel: [w428 w430] -> w416
                frame False {
                  n95 = Negate(x=w429) -> (-x=w428:sgl)
                }
                frame True {
                }
              }
            }
          }
          n96 = case shown="True" w337 {
            tunnel: w346 -> [_ w398]
            tunnel: [w383 w385] -> w340
            tunnel: [w383 w384] -> w339
            tunnel: w345 -> [_ w390]
            tunnel: w344 -> [_ w387]
            frame False {
              w383 = sgl 0.0
              # "Current Data Set Was Not Valid\nFill with 0\nWill not be used later"
            }
            frame True {
              # "Add delta for\nRIGHT camera ONLY"
              # "Estimate Distance"
              # "Negate dX if A2>90"
              # "Find LOCAL Coordinate of Each Beacon"
              # "Current - Valid Data Set"
              n97 = call "Scaling and Mapping2"("Signals"=w390) -> ("Scaled Signals"=w389:dynamicdata)  [unwired: 9 in, 1 out]
              n98 = To Single Precision Float(number=w389) -> (single precision float=w388:sgl)
              n99 = Less?(x=w398, y=sgl 90.0) -> (x < y?=w400:bool)
              n100 = case shown="False" w400 {
                tunnel: w398 -> [w407 w409]
                tunnel: [w405 w410] -> w397
                tunnel: [FALSE TRUE] -> w392
                frame False {
                  # "Negative Y"
                  # "A2 is > 90"
                  n101 = Subtract(x=w407, y=sgl 90.0) -> (x-y=w405:sgl)
                }
                frame True {
                  # "Positive Y"
                  # "A2 is < 90"
                  n102 = Subtract(x=sgl 90.0, y=w409) -> (x-y=w410:sgl)
                }
              }
              "dA2 3" <- w397
              n103 = expression code="(x/180.0)*pi" "degrees to radians"(w397) -> (w395:sgl)
              n104 = expression code="(x/180.0)*pi" "degrees to radians"(w397) -> (w396:sgl)
              n105 = Cosine(x=w395) -> (cos(x)=w393:sgl)
              n106 = Sine(x=w396) -> (sin(x)=w394:sgl)
              n107 = Multiply(x=w388, y=w393) -> (x*y=w384:sgl)
              n108 = Multiply(x=w388, y=w394) -> (x*y=w391:sgl)
              n109 = case shown="True" w392 {
                tunnel: w391 -> [w402 w403]
                tunnel: [w401 w403] -> w386
                frame False {
                  n110 = Negate(x=w402) -> (-x=w401:sgl)
                }
                frame True {
                }
              }
              n111 = Add(x=w387, y=w386) -> (x+y=w385:sgl)
            }
          }
          n112 = And(x=w338, y=w337) -> (x .and. y?=w343:bool)
          n113 = case shown="False" w343 {
            tunnel: w342 -> [w356 w382]
            tunnel: w341 -> [w353 w381]
            tunnel: w340 -> [w355 w380]
            tunnel: w339 -> [w354 w379]
            tunnel: [w351 w375] -> w336
            tunnel: [w350 w374] -> w335
            tunnel: w338 -> [w352 _]
            tunnel: w337 -> [w357 _]
            tunnel: [w349 TRUE] -> w334
            frame False {
              n114 = Exclusive Or(1:w357, 2:w352) -> (0:w358:bool)
              n115 = case shown="True" w358 {
                tunnel: w356 -> [_ w366]
                tunnel: w355 -> [_ w363]
                tunnel: w354 -> [_ w362]
                tunnel: w353 -> [_ w364]
                tunnel: w352 -> [_ w368]
                tunnel: [w359 w367] -> w351
                tunnel: [w359 w365] -> w350
                tunnel: [FALSE TRUE] -> w349
                frame False {
                  w359 = sgl 0.0
                  # "None are valid,"
                }
                frame True {
                  # "Only 1 beacon is valid,\nUse the valid beacon"
                  n116 = case shown="False" w368 {
                    tunnel: [w370 w372] -> w367
                    tunnel: w366 -> [_ w372]
                    tunnel: [w369 w371] -> w365
                    tunnel: w364 -> [_ w371]
                    tunnel: w363 -> [w370 _]
                    tunnel: w362 -> [w369 _]
                    frame False {
                      # "Left is invalid,\nRight MUST be valid"
                    }
                    frame True {
                      # "Left is Valid"
                    }
                  }
                }
              }
            }
            frame True {
              w376 = sgl 2.0 ("y")
              # "Both are Valid"
              n117 = Add(x=w382, y=w380) -> (x+y=w377:sgl)
              n118 = Add(x=w381, y=w379) -> (x+y=w378:sgl)
              n119 = Divide(x=w378, y=w376) -> (x/y=w374:sgl)
              n120 = Divide(x=w377, y=w376) -> (x/y=w375:sgl)
            }
          }
        }
        n121 = And(x="Valid Angles - L", y="Valid Angles -R") -> (x .and. y?=w150:bool[])
        n122 = Boolean To (0,1)(Boolean=w150) -> (0, 1=w147:i16[])
        n123 = Add Array Elements(numeric array=w147) -> (sum=w148:i16)
        n124 = Greater?(x=w148, y=1) -> (0:w146:bool)
        n125 = for {
          N: w162 -> [_]
          tunnel: w146 -> [w270]
          tunnel: "Beacon Angles - L" -> [w269] mode=indexing
          tunnel: "Beacon Angles -R" -> [w268] mode=indexing
          tunnel: "Distance Between \nCameras  (*unit)" -> [w267]
          tunnel: "Distance Threshold\nRef Triangles (*unit)" -> [w266]
          tunnel: [w265] -> w133 mode=indexing
          tunnel: [w264] -> _ mode=indexing
          tunnel: [w263] -> w132 mode=indexing
          tunnel: [w262] -> _ mode=indexing
          tunnel: [w261] -> w134 mode=indexing
          tunnel: [w260] -> w140 mode=indexing
          n126 = case shown="True" w270 {
            tunnel: w269 -> [w275 w285]
            tunnel: w268 -> [w274 w284]
            tunnel: w267 -> [_ w276]
            tunnel: w266 -> [_ w277]
            tunnel: [w275 w283] -> w265
            tunnel: [w274 w282] -> w264
            tunnel: [FALSE w281] -> w263
            tunnel: [w272 w280] -> w262
            tunnel: [w272 w279] -> w261
            tunnel: [0 w278] -> w260
            frame False {
              w272 = sgl 1.0
            }
            frame True {
              # "Build Reference Triangle"
              n127 = call "Position Calc_Build Reference Triangle_R1.vi"("A2_in"=w285, "A3_in"=w284, "S1 (Length Between\n Cameras - inches)"=w276, "Distance\nThreshold"=w277) -> ("S2"=w280:sgl, "S3"=w279:sgl, "Direction"=w278:i8, "A2"=w283:sgl, "A3"=w282:sgl, "Accept"=w281:bool)  [unwired: 6 in]
            }
          }
        }
        n128 = for {
          N: w162 -> [_]
          tunnel: w132 -> [w255] mode=indexing
          tunnel: w140 -> [w259] mode=indexing
          tunnel: [w259] -> w142 mode=indexing if=w255
          shift-right: [w258] -> w136
          shift-left: 0 -> [w256]
          # "Only add to array\nif valid distance"
          n129 = Increment(x=w256) -> (x+1=w257:i32)
          n130 = Select(t=w257, s=w255, f=w256) -> (s? t:f=w258:i32)
        }
        n131 = Index Array(array=w142, index=0) -> (element=w143:i32)
        n132 = Equal?(x=w142, y=w143) -> (x = y?=w144:bool[])
        n133 = And Array Elements(Boolean array=w144) -> (logical AND=w138:bool)
        n134 = Greater?(x=w136, y=1) -> (0:w137:bool)
        n135 = And(x=w138, y=w137) -> (x .and. y?=w131:bool)
        n136 = case shown="True" w131 {
          tunnel: w162 -> [w212 w221]
          tunnel: w134 -> [_ w220]
          tunnel: w133 -> [_ w219]
          tunnel: w132 -> [_ w218]
          tunnel: [w211 w217] -> w161
          tunnel: [w210 w216] -> w157
          tunnel: [w210 w215] -> w156
          frame False {
            # "Build Array for False"
            n137 = for {
              N: w212 -> [_]
              tunnel: [sgl 0.0] -> w210 mode=indexing
              tunnel: [FALSE] -> w211 mode=indexing
            }
          }
          frame True {
            n138 = for {
              N: w221 -> [_]
              tunnel: w219 -> [w227] mode=indexing
              tunnel: w220 -> [w226] mode=indexing
              tunnel: [w225] -> w216 mode=indexing
              tunnel: [w224] -> w215 mode=indexing
              tunnel: [w223] -> w217 mode=indexing
              tunnel: w218 -> [w222] mode=indexing
              n139 = case shown="True" w222 {
                selector: w222 -> [w229 w233]
                tunnel: w227 -> [_ w241]
                tunnel: [w228 w231] -> w225
                tunnel: [w228 w232] -> w224
                tunnel: w226 -> [_ w230]
                tunnel: [w229 w233] -> w223
                frame False {
                  w228 = sgl 0.0
                  # "Current Data Set Was Not Valid\nFill with 0\nWill not be used later"
                }
                frame True {
                  # "dY"
                  # "dX"
                  # "Negate dX if A2>90"
                  # "Find LOCAL Coordinate of Each Beacon"
                  # "Current - Valid Data Set"
                  n140 = Less?(x=w241, y=sgl 90.0) -> (x < y?=w243:bool)
                  n141 = case shown="False" w243 {
                    tunnel: w241 -> [w250 w252]
                    tunnel: [w248 w253] -> w240
                    tunnel: [FALSE TRUE] -> w235
                    frame False {
                      # "Negative Y"
                      # "A2 is > 90"
                      n142 = Subtract(x=w250, y=sgl 90.0) -> (x-y=w248:sgl)
                    }
                    frame True {
                      # "Positive Y"
                      # "A2 is < 90"
                      n143 = Subtract(x=sgl 90.0, y=w252) -> (x-y=w253:sgl)
                    }
                  }
                  "dA2 4" <- w240
                  n144 = expression code="(x/180.0)*pi" "degrees to radians"(w240) -> (w238:sgl)
                  n145 = expression code="(x/180.0)*pi" "degrees to radians"(w240) -> (w239:sgl)
                  n146 = Cosine(x=w238) -> (cos(x)=w236:sgl)
                  n147 = Sine(x=w239) -> (sin(x)=w237:sgl)
                  n148 = Multiply(x=w230, y=w236) -> (x*y=w232:sgl)
                  n149 = Multiply(x=w230, y=w237) -> (x*y=w234:sgl)
                  n150 = case shown="True" w235 {
                    tunnel: w234 -> [w245 w246]
                    tunnel: [w244 w246] -> w231
                    frame False {
                      n151 = Negate(x=w245) -> (-x=w244:sgl)
                    }
                    frame True {
                    }
                  }
                }
              }
            }
          }
        }
        n152 = Subtract(x=sgl 1.0, y="Triangle Based\nWeight") -> (x-y=w153:sgl)
        "Scale Based\nWeight" <- w153
        n153 = for {
          N: w162 -> [_]
          tunnel: w161 -> [w290] mode=indexing
          tunnel: w160 -> [w289] mode=indexing
          tunnel: w159 -> [w294] mode=indexing
          tunnel: w158 -> [w293] mode=indexing
          tunnel: w157 -> [w296] mode=indexing
          tunnel: w156 -> [w295] mode=indexing
          tunnel: "Triangle Based\nWeight" -> [w292]
          tunnel: w153 -> [w291]
          tunnel: [w288] -> w130 mode=indexing
          tunnel: [w287] -> w152 mode=indexing
          tunnel: [w286] -> w151 mode=indexing
          # "If Beacon info \nis available from\nboth"
          n154 = And(x=w290, y=w289) -> (x .and. y?=w297:bool)
          n155 = case shown="False" w297 {
            selector: w297 -> [_ w323]
            tunnel: w296 -> [w304 w331]
            tunnel: w295 -> [w302 w332]
            tunnel: w294 -> [w300 w330]
            tunnel: w293 -> [w299 w329]
            tunnel: w292 -> [_ w333]
            tunnel: w291 -> [_ w328]
            tunnel: [w303 w321] -> w286
            tunnel: [w305 w322] -> w287
            tunnel: w290 -> [w306 _]
            tunnel: w289 -> [w301 _]
            tunnel: [w298 w323] -> w288
            frame False {
              n156 = case shown="False" w306 {
                selector: w306 -> [_ w318]
                tunnel: [w311 w320] -> w305
                tunnel: w304 -> [_ w320]
                tunnel: [w309 w319] -> w303
                tunnel: w302 -> [_ w319]
                tunnel: w301 -> [w312 _]
                tunnel: w300 -> [w310 _]
                tunnel: w299 -> [w308 _]
                tunnel: [w307 w318] -> w298
                frame False {
                  n157 = case shown="False" w312 {
                    selector: w312 -> [w313 w315]
                    tunnel: [w314 w317] -> w311
                    tunnel: w310 -> [_ w317]
                    tunnel: [w314 w316] -> w309
                    tunnel: w308 -> [_ w316]
                    tunnel: [w313 w315] -> w307
                    frame False {
                      w314 = sgl 0.0
                      # "None avail"
                    }
                    frame True {
                    }
                  }
                }
                frame True {
                }
              }
            }
            frame True {
              n158 = Multiply(x=w331, y=w333) -> (x*y=w327:sgl)
              n159 = Multiply(x=w332, y=w333) -> (x*y=w325:sgl)
              n160 = Multiply(x=w330, y=w328) -> (x*y=w326:sgl)
              n161 = Multiply(x=w329, y=w328) -> (x*y=w324:sgl)
              n162 = Add(x=w327, y=w326) -> (x+y=w322:sgl)
              n163 = Add(x=w325, y=w324) -> (x+y=w321:sgl)
            }
          }
        }
        "Valid Beacon Sets_" <- w130
        n164 = Boolean To (0,1)(Boolean=w130) -> (0, 1=w173:i16[])
        n165 = Add Array Elements(numeric array=w173) -> (sum=w172:i16)
        n166 = Greater?(x=w172, y=i16 1) -> (0:w170:bool)
        n167 = case shown="True" w170 {
          tunnel: w204 -> [_ w529]
          tunnel: [0.0 ("f") w528] -> w200
          tunnel: [w441 w527] -> w199
          tunnel: w194 -> [_ w445]
          tunnel: w193 -> [_ w526]
          tunnel: [FALSE w525] -> w184
          tunnel: [FALSE w524] -> w183
          tunnel: w181 -> [_ w523]
          tunnel: [sgl 0.0 w521] -> w174
          tunnel: "Distance Between \nCameras  (*unit)" -> [_ w457]
          tunnel: w152 -> [_ w456]
          tunnel: w151 -> [_ w455]
          tunnel: w130 -> [_ w454]
          tunnel: w162 -> [_ w453]
          frame False {
            w440 = 0.0 ("f")
            n168 = Bundle("f"=w440, "f"=w440) -> (w441:cluster{"f":dbl, "f":dbl})  [unwired: 1 in]
          }
          frame True {
            w493 = sgl 2.0
            w510 = 0
            # "Valid Position Ccount"
            # "Only Apply This Filtering \nif 3 or More Beacons Still Valid"
            # "Orientation Value"
            # "Orientation Valid"
            # "Y (current)"
            # "X (current)"
            # "Number of Valid\nPrevious Orientations"
            # "More than 1 Previous\nValid Positions"
            # "More than\n2previous position\navailable"
            # "Choose Beacon Set\nwith Lowest Std Dev"
            # "Y value cannot be negative"
            # "Find New # Of Valid Beacons"
            # "Adjust/Normalize\nLocal Beacon Positions\nusing Line of Best fit"
            # "# Valid\nData Sets"
            # "cam, y"
            # "cam, x"
            # "Calculate dX and dY\nfor right cam"
            # "Average dX and dY from each (valid) beacon to find position of each camera\n\nthen average all  positions for each camera find center between"
            # "Convert Slope\nto Radians"
            # "*rotate CCW in rad"
            # "Rotate Coordinate\n System by Slope"
            n169 = Boolean To (0,1)(Boolean=w445) -> (0, 1=w477:i16[])
            n170 = Initialize Array(u8 0, "Moving Average\nWindow Length") -> (w450:u8[])
            n171 = Add Array Elements(numeric array=w477) -> (sum=w471:i16)
            n172 = Greater?(x=w471, y=0) -> (0:w447:bool)
            n173 = while {
              shift-right: [w531] -> w448
              shift-left: w450 -> [w533]
              tunnel: w445 -> [w538] mode=indexing
              shift-right: [w537] -> w446
              shift-left: u8 0 -> [w539]
              tunnel: "Moving Average\nWindow Length" -> [w530]
              i -> [w532]
              stop <- w534 stop-if-true
              # "Grab Last 2 Valid Position Indexes"
              n174 = case shown="True" w538 {
                tunnel: w539 -> [w541 w543]
                tunnel: [w541 w546] -> w537
                tunnel: w533 -> [w540 w545]
                tunnel: w532 -> [_ w544]
                tunnel: [w540 w542] -> w531
                frame False {
                }
                frame True {
                  # "Update Index\nto use"
                  # "Increment\nValid Count"
                  n175 = Replace Array Subset(array=w545, new element=w544, index=w543) -> (w542:u8[])
                  n176 = Increment(x=w543) -> (x+1=w546:u8)
                }
              }
              n177 = Greater Or Equal?(x=w537, y=w530) -> (x >= y?=w536:bool)
              n178 = Greater Or Equal?(x=w532, y=w530) -> (x >= y?=w535:bool)
              n179 = Or(x=w536, y=w535) -> (x .or. y?=w534:bool)
            }
            n180 = Bundle(w456, w455) -> (→"LOCAL\nBeacon Coordinates\nRelative to Robot" →"Local Coordinates - Calculated":cluster{sgl[], sgl[]})  [unwired: 1 in]
            n181 = call "Coordinate_Outlier_Filtering_R1.vi"("Num of Beacons"=w453, "Max Std Dev(all 5)"="Max Std Dev (5)", "X in"=w456, "Valid Data\nSets in"=w454, "Y in"=w455, "Max Std Dev( 4 )"="Max Std Dev (4)", "Max Std Dev (3)"="Max Std Dev (3)") -> ("Y out"=w467:sgl[], "X out"=w468:sgl[], "Valid Beacons\nout"=w465:bool[], "Slope out"=w474:dbl)  [unwired: 3 in, 2 out]
            n182 = Inverse Tangent(1:w474) -> (0:w489:dbl)
            n183 = expression code="(x/pi)*180.0" "radians to degrees"(w489) -> (w473:dbl)
            n184 = Boolean To (0,1)(Boolean=w465) -> (0, 1=w464:i16[])
            n185 = To Single Precision Float(number=w473) -> (single precision float=w521:sgl)
            n186 = case shown="True" w447 {
              tunnel: [w556 w567] -> w524
              tunnel: w526 -> [_ w570]
              tunnel: w521 -> [w557 w564]
              tunnel: [w555 w568] -> w528
              tunnel: w523 -> [_ _]
              tunnel: w448 -> [_ w562]
              tunnel: w446 -> [_ w561]
              frame False {
                # "Since no history available,\ncheck that current is with 0-360"
                # "Use Current Orientation bc \nPrevious are not available"
                # "New Position\nValid"
                n187 = In Range and Coerce(upper limit=sgl 360.0, x=w557, lower limit=sgl -360.0 ("upper limit")) -> (In Range?=w556:bool)  [unwired: 1 out]
                n188 = Select(t=w557, s=w556, f=sgl 0.0) -> (s? t:f=w555:sgl)
              }
              frame True {
                # "Moving Average Out"
                n189 = for {
                  N: w561 -> [_]
                  shift-right: [w596] -> w572
                  shift-left: 0.0 -> [w595]
                  tunnel: w562 -> [w594] mode=indexing
                  tunnel: w570 -> [w592]
                  # "Fetch Last Valid Values\nand Sum"
                  n190 = Index Array(array=w592, index=w594) -> (element=w593:sgl)
                  n191 = Add(x=w593, y=w595) -> (x+y=w596:dbl)
                }
                n192 = Increment(x=w561) -> (x+1=w563:u8)
                n193 = Add(x=w564, y=w572) -> (x+y=w565:dbl)
                n194 = To Double Precision Float(number=w563) -> (double precision float=w571:dbl)
                n195 = Divide(x=w565, y=w571) -> (x/y=w569:dbl)
                n196 = Greater Than 0?(x=w563) -> (x > 0?=w566:bool)
                n197 = case shown="True" w566 {
                  tunnel: w569 -> [w576 w582]
                  tunnel: w562 -> [_ w589]
                  tunnel: w570 -> [_ w588]
                  tunnel: [w575 w581] -> w568
                  tunnel: [w574 w584] -> w567
                  frame False {
                    # "No Pevious is Available to Compare\ncheck that current is real angle"
                    n198 = In Range and Coerce(upper limit=sgl 360.0, x=w576, lower limit=sgl -360.0 ("upper limit")) -> (In Range?=w574:bool)  [unwired: 1 out]
                    n199 = Select(t=w576, s=w574, f=sgl 0.0) -> (s? t:f=w575:dbl)
                  }
                  frame True {
                    # "Calculate New, Weighted\nOrientation"
                    # "Check That New Value\nis within Range of Old\n(avg)"
                    # "(X1 - X2)^2"
                    # "Previous"
                    # "Pevious is Available to Compare"
                    n200 = Index Array(array=w589, index=u8 0) -> (element=w590:u8)
                    n201 = Index Array(array=w588, index=w590) -> (element=w587:sgl)
                    n202 = Subtract(x=w587, y=w582) -> (x-y=w586:dbl)
                    n203 = Absolute Value(x=w586) -> (abs(x)=w585:dbl)
                    n204 = Less Or Equal?(x=w585, y="New Orientation \nThreshold") -> (x <= y?=w584:bool)
                    n205 = Select(t=w582, s=w584, f=sgl 0.0) -> (s? t:f=w581:dbl)
                  }
                }
              }
            }
            n206 = Add Array Elements(numeric array=w464) -> (sum=w463:i16)
            n207 = Greater?(x=w463, y=i16 2) -> (0:w461:bool)
            n208 = case shown="True" w461 {
              tunnel: w453 -> [_ w554]
              tunnel: w465 -> [w547 w553]
              tunnel: w468 -> [_ w552]
              tunnel: w467 -> [_ w551]
              tunnel: [w547 w550] -> w466
              tunnel: "Distance\nBetween Beacons" -> [_ w549]
              tunnel: "Distance\nBetween Beacons \n- Tolerance" -> [_ w548]
              frame False {
                # "Don't apply filtering,\nnot enough data points"
              }
              frame True {
                # "This will filter beacons if they are calculate to be \ntoo close to each other. The beacon(s) that is\n discarded is chosen based distance between each/every\nbeacon,. Capable of filtering as long as 1/2 of sample\nset has uniform distances (between beacons)."
                # "Validate Distance Between\nEach Beacon"
                n209 = call "Beacon_Filtering_Inter_Beacon_Distance_R1.vi"("Num of Beacons"=w554, "Inter Beacon\nReal Distance"=w549, "X in"=w552, "Inter Beacon\ndelta Threshold"=w548, "Y in"=w551, "Valid Data\nSets in"=w553) -> ("Beacons Valid - Out"=w550:bool[])  [unwired: 9 in]
              }
            }
            "Post Filtering\n- Valid Beacons" <- w466
            n210 = Increment(x=w453) -> (x+1=w511:i8)
            n211 = for {
              N: w511 -> [_]
              tunnel: [w709] -> w512 mode=indexing
              tunnel: w468 -> [w705]
              tunnel: w467 -> [w708]
              tunnel: [w707] -> w513 mode=indexing
              tunnel: w457 -> [w704]
              i -> [w706]
              # "Build Array's of Coordinates\nFor All Objects"
              n212 = Greater Than 0?(x=w706) -> (x > 0?=w710:bool)
              n213 = case shown="True" w710 {
                tunnel: [w712 w718] -> w709
                tunnel: w705 -> [w715 _]
                tunnel: w708 -> [w714 _]
                tunnel: [w711 0.0] -> w707
                tunnel: w706 -> [w716 _]
                tunnel: w704 -> [_ w718]
                frame True {
                  # "Rest of Array is\nBeacon Coordinates"
                  n214 = Decrement(x=w716) -> (x-1=w713:i32)
                  n215 = Index Array(array=w715, index=w713) -> (element=w712:sgl)
                  n216 = Index Array(array=w714, index=w713) -> (element=w711:sgl)
                }
                frame False {
                  # "First object is the\nother Camera\n\nthis coordinate\nis simply:\nx = 0\ny = distance btween cams"
                }
              }
            }
            n217 = Bundle(w512, w513) -> (→"All Object Coordinates \n- Local" →"Local Coordinates - Normalized":cluster{sgl[], dbl[]})  [unwired: 1 in]
            n218 = expression code="(x/180.0)*pi" "degrees to radians"(w528) -> (w472:dbl)
            n219 = call-poly <vilib>:"2D Cartesian Coordinate Rotation.vi"("theta"=w472, "Y"=w513, "X"=w512) -> ("Y Out"=w490:dbl[], "X Out"=w491:dbl[])  [unwired: 6 in, 1 out]
            n220 = Bundle("X Out"=w491, "Y Out"=w490) -> (→"All Object Coordinates \n- Local - Rotated" →"Local Coordinates - Rotated":cluster{"X Out":dbl[], "Y Out":dbl[]})  [unwired: 1 in]
            n221 = Index Array(array=w490, index=w510) -> (element=w486:dbl)
            n222 = Index Array(array=w491, index=w510) -> (element=w509:dbl)
            n223 = for {
              N: w453 -> [_]
              tunnel: w490 -> [w700]
              tunnel: w491 -> [w701]
              tunnel: w509 -> [w699]
              tunnel: w486 -> [w698]
              tunnel: [w697] -> w483 mode=indexing
              tunnel: [w696] -> w482 mode=indexing
              tunnel: [w695] -> w458 mode=indexing
              tunnel: [w694] -> w484 mode=indexing
              i -> [w703]
              n224 = Increment(x=w703) -> (x+1=w702:i32)
              n225 = Index Array(array=w700, index=w702) -> (element=w694:dbl)
              n226 = Index Array(array=w701, index=w702) -> (element=w695:dbl)
              n227 = Subtract(x=w694, y=w698) -> (x-y=w696:dbl)
              n228 = Subtract(x=w695, y=w699) -> (x-y=w697:dbl)
            }
            n229 = Bundle(w483, w482) -> (→"dX, dY\nRight Cam":cluster{dbl[], dbl[]})  [unwired: 1 in]
            n230 = Bundle(w458, w484) -> (→"dX, dY\nLeft Cam":cluster{dbl[], dbl[]})  [unwired: 1 in]
            n231 = Unbundle("Real Beacon\n - Coordinates") -> ("X"=w507:dbl[], "Y"=w487:dbl[])
            n232 = Boolean To (0,1)(Boolean=w466) -> (0, 1=w485:i16[])
            n233 = for {
              N: w453 -> [_]
              tunnel: w466 -> [w680] mode=indexing
              tunnel: w507 -> [w677] mode=indexing
              tunnel: w487 -> [w676] mode=indexing
              tunnel: w458 -> [w679] mode=indexing
              tunnel: w484 -> [w675] mode=indexing
              tunnel: w483 -> [w678] mode=indexing
              tunnel: w482 -> [w674] mode=indexing
              tunnel: [w673] -> w506 mode=indexing
              tunnel: [w672] -> w505 mode=indexing
              tunnel: [w671] -> w504 mode=indexing
              tunnel: [w670] -> w503 mode=indexing
              n234 = case shown="True" w680 {
                tunnel: w679 -> [_ w693]
                tunnel: w678 -> [_ w692]
                tunnel: w677 -> [_ w683]
                tunnel: w676 -> [_ w682]
                tunnel: w675 -> [_ w691]
                tunnel: w674 -> [_ w684]
                tunnel: [w681 w689] -> w673
                tunnel: [w681 w688] -> w672
                tunnel: [w681 w687] -> w671
                tunnel: [w681 w686] -> w670
                frame False {
                  w681 = sgl 0.0
                  # "Add Nothing"
                }
                frame True {
                  # "realX = beaconX + dY\nrealY = beaconY + (-dx)"
                  # "Right Cam"
                  # "Left Cam"
                  # "dX = -dX\nSwap dX, dY"
                  # "Translate to Real Coordinates\nOnly Apply for Valid Beacons"
                  n235 = Negate(x=w693) -> (-x=w690:dbl)
                  n236 = Negate(x=w692) -> (-x=w685:dbl)
                  n237 = Add(x=w683, y=w691) -> (x+y=w689:dbl)
                  n238 = Add(x=w682, y=w690) -> (x+y=w688:dbl)
                  n239 = Add(x=w683, y=w684) -> (x+y=w687:dbl)
                  n240 = Add(x=w682, y=w685) -> (x+y=w686:dbl)
                }
              }
            }
            n241 = Add Array Elements(numeric array=w485) -> (sum=w488:i16)
            n242 = Add Array Elements(numeric array=w506) -> (sum=w502:dbl)
            n243 = Add Array Elements(numeric array=w505) -> (sum=w501:dbl)
            n244 = Add Array Elements(numeric array=w504) -> (sum=w500:dbl)
            n245 = Add Array Elements(numeric array=w503) -> (sum=w499:dbl)
            n246 = Divide(x=w502, y=w488) -> (x/y=w498:dbl)
            n247 = Divide(x=w501, y=w488) -> (x/y=w496:dbl)
            n248 = Divide(x=w500, y=w488) -> (x/y=w497:dbl)
            n249 = Divide(x=w499, y=w488) -> (x/y=w495:dbl)
            n250 = Bundle(w498, w496) -> (→"Left Camera Real Coordinates":cluster{dbl, dbl})  [unwired: 1 in]
            n251 = Bundle(w497, w495) -> (→"Right Camera Real Coordinate":cluster{dbl, dbl})  [unwired: 1 in]
            n252 = Add(x=w498, y=w497) -> (x+y=w494:dbl)
            n253 = Add(x=w496, y=w495) -> (x+y=w492:dbl)
            n254 = Divide(x=w494, y=w493) -> (x/y=w476:dbl)
            n255 = Divide(x=w492, y=w493) -> (x/y=w475:dbl)
            n256 = Bundle(w476, w475) -> (→"Robot Coordinates":cluster{dbl, dbl})  [unwired: 1 in]
            n257 = Less Than 0?(x=w475) -> ()  [unwired: 1 out]
            n258 = case shown="True" w447 {
              tunnel: w471 -> [_ _]
              tunnel: w476 -> [w601 w618]
              tunnel: [w602 w629] -> w525
              tunnel: w529 -> [_ w623]
              tunnel: w475 -> [w600 w617]
              tunnel: [w599 w633] -> w527
              tunnel: "Max X (arena)" -> [w598 w628]
              tunnel: "Max Y (arena)" -> [w597 w627]
              tunnel: w448 -> [_ w625]
              tunnel: w446 -> [_ w624]
              frame False {
                # "New Position\nValid"
                # "Since no history available,\ncheck that current is within\nthe bounds of the arena size"
                # "Use Current Position bc \nPrevious are not available"
                n259 = In Range and Coerce(upper limit=w598, x=w601, lower limit=sgl 0.0 ("upper limit")) -> (In Range?=w604:bool)  [unwired: 1 out]
                n260 = In Range and Coerce(upper limit=w597, x=w600, lower limit=sgl 0.0 ("upper limit")) -> (In Range?=w603:bool)  [unwired: 1 out]
                n261 = Bundle(w601, w600) -> (w599:cluster{dbl, dbl})  [unwired: 1 in]
                n262 = And(x=w604, y=w603) -> (x .and. y?=w602:bool)
              }
              frame True {
                w626 = 0.0
                # "If needed, make seperate FOR Loop for \nY only... Using more previous values than X"
                # "New Y"
                # "New X"
                # "Only consider if velocity is\ngreater than certain speed"
                # "Weighted Robot \nCoordinates"
                # "Position\nValid\n(current)"
                n263 = for {
                  N: w624 -> [_]
                  shift-right: [w642] -> w622
                  shift-left: w626 -> [w641]
                  shift-right: [w640] -> w621
                  shift-left: w626 -> [w639]
                  tunnel: w625 -> [w637] mode=indexing
                  tunnel: w623 -> [w635]
                  # "Fetch Last Valid Values\nand Sum"
                  n264 = Index Array(array=w635, index=w637) -> (element=w636:cluster{sgl, sgl})
                  n265 = Unbundle(w636) -> (w638:sgl, w634:sgl)
                  n266 = Add(x=w634, y=w639) -> (x+y=w640:dbl)
                  n267 = Add(x=w638, y=w641) -> (x+y=w642:dbl)
                }
                n268 = To Single Precision Float(number=w624) -> (single precision float=w611:sgl)
                n269 = Subtract(x=sgl 1.0, y="New Position\nWeight") -> (x-y=w620:sgl)
                n270 = Multiply(x=w620, y=w622) -> (x*y=w612:dbl)
                n271 = Multiply(x=w620, y=w621) -> (x*y=w613:dbl)
                n272 = Divide(x=w612, y=w611) -> (x/y=w609:dbl)
                n273 = Divide(x=w613, y=w611) -> (x/y=w610:dbl)
                n274 = Multiply(x="New Position\nWeight", y=w618) -> (x*y=w615:dbl)
                n275 = Multiply(x="New Position\nWeight", y=w617) -> (x*y=w614:dbl)
                n276 = Add(x=w615, y=w609) -> (x+y=w608:dbl)
                n277 = Add(x=w614, y=w610) -> (x+y=w607:dbl)
                n278 = Greater Than 0?(x=w624) -> (x > 0?=w632:bool)
                n279 = case shown="True" w632 {
                  tunnel: w608 -> [w647 w654]
                  tunnel: w607 -> [w646 w653]
                  tunnel: w625 -> [_ w666]
                  tunnel: w623 -> [_ w665]
                  tunnel: [w644 w654] -> w631
                  tunnel: [w643 w653] -> w630
                  tunnel: [w648 w655] -> w629
                  tunnel: w628 -> [w650 _]
                  tunnel: w627 -> [w649 _]
                  frame False {
                    w645 = sgl 0.0 ("upper limit")
                    # "Check that within bounds of arena"
                    # "No Pevious is Available to Compare"
                    n280 = In Range and Coerce(upper limit=w650, x=w647, lower limit=w645) -> (In Range?=w652:bool)  [unwired: 1 out]
                    n281 = In Range and Coerce(upper limit=w649, x=w646, lower limit=w645) -> (In Range?=w651:bool)  [unwired: 1 out]
                    n282 = And(x=w652, y=w651) -> (x .and. y?=w648:bool)
                    n283 = Select(t=w647, s=w648, f=w645) -> (s? t:f=w644:dbl)
                    n284 = Select(t=w646, s=w648, f=w645) -> (s? t:f=w643:dbl)
                  }
                  frame True {
                    # "New"
                    # "(Y1 - Y2)^2"
                    # "(X1 - X2)^2"
                    # "Previous"
                    # "Pevious is Available to Compare"
                    n285 = Index Array(array=w666, index=u8 0) -> (element=w668:u8)
                    n286 = Index Array(array=w665, index=w668) -> (element=w667:cluster{sgl, sgl})
                    n287 = Unbundle(w667) -> (w657:sgl, w656:sgl)
                    n288 = Subtract(x=w657, y=w654) -> (x-y=w662:dbl)
                    n289 = Subtract(x=w653, y=w656) -> (x-y=w661:dbl)
                    n290 = Square(x=w662) -> (x^2=w660:dbl)
                    n291 = Square(x=w661) -> (x^2=w659:dbl)
                    n292 = Add(x=w660, y=w659) -> (x+y=w663:dbl)
                    n293 = Square Root(x=w663) -> (sqrt(x)=w658:dbl)
                    n294 = Less Or Equal?(x=w658, y="New Position \nThreshold") -> (x <= y?=w655:bool)
                  }
                }
                n295 = Bundle("upper limit"=w631, "upper limit"=w630) -> (w633:cluster{"upper limit":dbl, "upper limit":dbl})  [unwired: 1 in]
              }
            }
          }
        }
        "Orietnation\n(current)" <- w174
        n296 = And(x=w184, y=w183) -> (x .and. y?=w188:bool)
        "Position Valid" <- w188
        n297 = Exclusive Or(1:w183, 2:w184) -> (0:w182:bool)
        n298 = case shown="True" w188 {
          tunnel: [w725 w728] -> w198
          tunnel: [w726 w727] -> w187
          tunnel: w200 -> [_ w728]
          tunnel: w199 -> [_ w727]
          tunnel: w182 -> [_ _]
          frame False {
            w725 = sgl 0.0 ("f")
            n299 = Bundle("f"=w725, "f"=w725) -> (w726:cluster{"f":sgl, "f":sgl})  [unwired: 1 in]
          }
          frame True {
            # "For Servos"
            "Last Orientation" <- w728
            "Last Position" <- w727
          }
        }
        "Robot Coordinates - Avgd" <- w187
        "Orientation Avgd" <- w198
        n300 = local read "History Size"() -> (w176:u8)
        n301 = Decrement(x=w176) -> (x-1=w177:u8)
        n302 = for {
          N: w176 -> [_]
          shift-right: [w766] -> w202
          shift-left: w197 -> [w765]
          tunnel: w187 -> [w764]
          tunnel: w177 -> [w763]
          i -> [w762]
          n303 = Subtract(x=w763, y=w762) -> (x-y=w761:i32)
          n304 = Equal To 0?(x=w761) -> (x = 0?=w760:bool)
          n305 = case shown="False" w760 {
            tunnel: w761 -> [w768 w773]
            tunnel: w765 -> [w771 w774]
            tunnel: [w769 w775] -> w766
            tunnel: w764 -> [_ w772]
            frame False {
              n306 = Decrement(x=w768) -> (x-1=w767:i32)
              n307 = Index Array(array=w771, index=w767) -> (element=w770:cluster{sgl, sgl})
              n308 = Replace Array Subset(array=w771, new element=w770, index=w768) -> (w769:cluster{sgl, sgl}[])
            }
            frame True {
              n309 = Replace Array Subset(array=w774, new element=w772, index=w773) -> (w775:cluster{sgl, sgl}[])
            }
          }
        }
        n310 = Decrement(x=w176) -> (x-1=w178:u8)
        n311 = for {
          N: w176 -> [_]
          shift-right: [w750] -> w203
          shift-left: w196 -> [w749]
          tunnel: w198 -> [w748]
          tunnel: w178 -> [w747]
          i -> [w746]
          n312 = Subtract(x=w747, y=w746) -> (x-y=w744:i32)
          n313 = Equal To 0?(x=w744) -> (x = 0?=w745:bool)
          n314 = case shown="False" w745 {
            tunnel: w744 -> [w752 w757]
            tunnel: w749 -> [w755 w758]
            tunnel: [w753 w759] -> w750
            tunnel: w748 -> [_ w756]
            frame False {
              # "Shift"
              n315 = Decrement(x=w752) -> (x-1=w751:i32)
              n316 = Index Array(array=w755, index=w751) -> (element=w754:sgl)
              n317 = Replace Array Subset(array=w755, new element=w754, index=w752) -> (w753:sgl[])
            }
            frame True {
              # "insert new"
              n318 = Replace Array Subset(array=w758, new element=w756, index=w757) -> (w759:sgl[])
            }
          }
        }
        n319 = Decrement(x=w176) -> (x-1=w175:u8)
        n320 = for {
          N: w176 -> [_]
          shift-right: [w735] -> w201
          shift-left: w195 -> [w734]
          tunnel: w188 -> [w733]
          tunnel: w175 -> [w732]
          i -> [w731]
          n321 = Subtract(x=w732, y=w731) -> (x-y=w729:i32)
          n322 = Equal To 0?(x=w729) -> (x = 0?=w730:bool)
          n323 = case shown="False" w730 {
            tunnel: w734 -> [w740 w742]
            tunnel: [w738 w743] -> w735
            tunnel: w733 -> [_ w741]
            tunnel: w729 -> [w736 _]
            frame False {
              n324 = Decrement(x=w736) -> (x-1=w737:i32)
              n325 = Index Array(array=w740, index=w737) -> (element=w739:bool)
              n326 = Replace Array Subset(array=w740, new element=w739, index=w736) -> (w738:bool[])
            }
            frame True {
              n327 = Replace Array Subset(array=w742, new element=w741) -> (w743:bool[])  [unwired: 1 in]
            }
          }
        }
        n328 = Boolean To (0,1)(Boolean=w201) -> (0, 1=w192:i16[])
        n329 = Add Array Elements(numeric array=w192) -> (sum=w190:i16)
        n330 = Greater Or Equal?(x=w190, y=i16 2) -> (x >= y?=→"Position \nLock Status":bool)
        n331 = case shown="True" w188 {
          tunnel: w187 -> [_ w724]
          frame False {
          }
          frame True {
            # "update debug graph\nif current is valid"
            n332 = Unbundle(w724) -> ("upper limit"=w723:dbl, "upper limit"=w722:dbl)
            n333 = Build Array(w722) -> (w720:dbl[])
            n334 = Build Array(w723) -> (w721:dbl[])
            n335 = Bundle(w721, w720) -> (→"Real Position in Course 2":cluster{dbl[], dbl[]})  [unwired: 1 in]
          }
        }
      }
    }
    n336 = case shown="True" w113 {
      tunnel: w112 -> [_ w120]
      frame False {
      }
      frame True {
        n337 = call "Tick Count3"() -> ("Tick Count(uSec)"=w121:u32)
        n338 = Subtract(x=w121, y=w120) -> (x-y=w124:u32)
        n339 = Divide(x=w124, y=u32 1000 ("x")) -> (x/y=→"dT":dbl)
      }
    }
    n340 = call "Tick Count6"() -> ("Tick Count(uSec)"=w110:u32)
    "Robot Coordinates\nHistory" <- w109
    "Orientation\nHistory" <- w114
    "Position Valid\nHistory" <- w115
  }
  n341 = disable-structure shown="Enabled" {
    disable-tunnel: [w778 _] -> _
    disable-tunnel: ["Search Step Size\n(deg)" _] -> _
    frame Enabled {
      n342 = Multiply(x=3.413333333333333, y="Search Step Size\n(deg)") -> (x*y=w776:dbl)
      n343 = To Unsigned Word Integer(number=w776) -> (unsigned 16bit integer=w778:u16)
    }
    frame Disabled {
    }
  }
  n344 = Multiply(x="Move Servo\nThreshold (deg)", y=3.413333333333333) -> (x*y=w18:dbl)
  n345 = To Unsigned Word Integer(number=w18) -> ()  [unwired: 1 out]
  n346 = call "Tick Count8"() -> ()  [unwired: 1 out]
  n347 = flat-sequence {
    tunnel: [w782] -> w42
    tunnel: [w781] -> w41
    tunnel: [w786] -> w40
    tunnel: ["Left Servo\nID"] -> w29
    tunnel: ["Right Servo\nID"] -> w28
    tunnel: ["Compliance Slope"] -> w27
    tunnel: [w826] -> w39
    tunnel: [w825] -> w38
    tunnel: w42 -> [w824]
    tunnel: w41 -> [w823]
    tunnel: w40 -> [w822]
    tunnel: w29 -> [w820]
    tunnel: w28 -> [w819]
    tunnel: w27 -> [w818]
    tunnel: w39 -> [w1099]
    tunnel: w38 -> [w1098]
    frame #0 {
      # "BAUD RATE"
      # "Initialize UART and DIO"
      n348 = call-poly "VISA Configure Serial Port"("VISA resource name"=refnum<visa-resource-name> "ASRL1::INSTR", "Enable Termination\nChar (T)"=FALSE ("Enable Termination\nChar (T)"), "baud rate (9600)"=u32 115200) -> ("VISA resource name out"=w782:refnum<visa-resource-name>)  [unwired: 11 in, 1 out]
      n349 = call <vilib>:"Smart Open.vi"("Channel Names"=tag[] ["A/DIO2"]) -> ("DIO Ref Out"=w781:T7)  [unwired: 9 in, 1 out]
      n350 = flat-sequence {
        tunnel: w782 -> [w794]
        tunnel: w781 -> [w793]
        tunnel: "Left Servo\nID" -> [w795]
        tunnel: [w792] -> w783
        tunnel: "Compliance Slope" -> [w791]
        tunnel: "Right Servo\nID" -> [w808]
        tunnel: w783 -> [w807]
        tunnel: "Compliance Slope" -> [w806]
        tunnel: w782 -> [w805]
        tunnel: w781 -> [w804]
        frame #0 {
          w792 = 3
          n351 = while {
            tunnel: w792 -> [w801]
            tunnel: w794 -> [w799]
            tunnel: w793 -> [w798]
            tunnel: w795 -> [w797]
            tunnel: w791 -> [w796]
            i -> [w802]
            stop <- w800 stop-if-true
            n352 = call "Set_Compliance_Slope_R2.vi"("Compliance Slope"=w796, "DIO Ref Out"=w798, "VISA resource name"=w799, "Servo ID"=w797) -> ()  [unwired: 6 in, 2 out]
            n353 = Increment(x=w802) -> (x+1=w803:i32)
            n354 = Greater Or Equal?(x=w803, y=w801) -> (x >= y?=w800:bool)
          }
        }
        frame #1 {
          n355 = while {
            tunnel: w807 -> [w814]
            tunnel: w808 -> [w812]
            tunnel: w805 -> [w811]
            tunnel: w804 -> [w810]
            tunnel: w806 -> [w809]
            i -> [w815]
            stop <- w813 stop-if-true
            n356 = call "Set_Compliance_Slope_R2.vi"("Compliance Slope"=w809, "DIO Ref Out"=w810, "VISA resource name"=w811, "Servo ID"=w812) -> ()  [unwired: 6 in, 2 out]
            n357 = Increment(x=w815) -> (x+1=w816:i32)
            n358 = Greater Or Equal?(x=w816, y=w814) -> (x >= y?=w813:bool)
          }
        }
      }
      n359 = call "Tick Count"() -> ("Tick Count(uSec)"=w786:u32)
    }
    frame #1 {
      # "Service Count"
      n360 = while {
        shift-right: [w829] -> _
        shift-left: w822 -> [w846]
        tunnel: "Max Write\nTx Attempts" -> [w841]
        tunnel: "Max Read\nTx Attempts" -> [w840]
        shift-right: [w836] -> w826
        shift-left: w824 -> [w839]
        shift-right: [w835] -> w825
        shift-left: w823 -> [w838]
        tunnel: w820 -> [w834]
        tunnel: w819 -> [w833]
        tunnel: w818 -> [w832]
        shift-right: [w830] -> _
        shift-left: u16 0 -> [w831]
        stop <- "close comms" stop-if-true
        # "Loop Timer"
        n361 = local read "SERVO ENABLE"() -> (w828:bool)
        n362 = call "Tick Count2"() -> ("Tick Count(uSec)"=w829:u32)
        n363 = Subtract(x=w829, y=w846) -> (x-y=w845:u32)
        n364 = call "Wait4"("Count(mSec)"="Servo Comm\nLoop Time (ms)") -> ()  [unwired: 1 out]
        n365 = Divide(x=w845, y=u32 1000) -> (x/y=→"dT - Comm Loop":dbl)
        n366 = case shown="True" w828 {
          tunnel: w841 -> [_ w855]
          tunnel: w840 -> [_ w886]
          tunnel: w839 -> [w849 w850]
          tunnel: w838 -> [w848 w879]
          tunnel: [w849 w852] -> w836
          tunnel: [w848 w851] -> w835
          tunnel: w834 -> [_ w858]
          tunnel: w833 -> [_ w857]
          tunnel: w832 -> [_ w856]
          tunnel: w831 -> [_ w854]
          tunnel: [u16 100 w853] -> w830
          frame False {
            # "Restart at same value\nUsed to Periodically update \nCompliance Slope"
          }
          frame True {
            n367 = flat-sequence {
              tunnel: [w892] -> w890
              tunnel: [w893] -> w889
              tunnel: [w891] -> w888
              tunnel: w886 -> [w894]
              tunnel: [w896] -> w877
              tunnel: [w895] -> w875
              tunnel: w850 -> [w896]
              tunnel: w879 -> [w895]
              tunnel: w858 -> [w891]
              tunnel: w890 -> [w914]
              tunnel: w889 -> [w915]
              tunnel: w888 -> [w913]
              tunnel: [w913] -> w887
              tunnel: [w912] -> w880
              tunnel: [w911] -> w878
              tunnel: w877 -> [w911]
              tunnel: [w910] -> w876
              tunnel: w875 -> [w910]
              tunnel: w887 -> [w936]
              tunnel: w855 -> [w935]
              tunnel: w880 -> [w930]
              tunnel: w878 -> [w932]
              tunnel: w876 -> [w931]
              tunnel: [w932] -> w873
              tunnel: [w931] -> w871
              tunnel: [w969] -> w874
              tunnel: w873 -> [w969]
              tunnel: [w968] -> w872
              tunnel: w871 -> [w968]
              tunnel: ["Servo Comm\nWait Time - (ms)"] -> w863
              tunnel: w886 -> [w976]
              tunnel: [w975] -> w885
              tunnel: [w974] -> w884
              tunnel: [w970] -> w882
              tunnel: w874 -> [w973]
              tunnel: w872 -> [w972]
              tunnel: [w973] -> w870
              tunnel: [w972] -> w867
              tunnel: [w971] -> w864
              tunnel: w863 -> [w971]
              tunnel: w857 -> [w970]
              tunnel: w885 -> [w996]
              tunnel: w884 -> [w995]
              tunnel: [w994] -> w883
              tunnel: w882 -> [w994]
              tunnel: [w993] -> w881
              tunnel: w870 -> [w992]
              tunnel: [w992] -> w869
              tunnel: [w991] -> w868
              tunnel: w867 -> [w991]
              tunnel: w864 -> [w990]
              tunnel: [w990] -> w862
              tunnel: w883 -> [w1018]
              tunnel: w881 -> [w1016]
              tunnel: w855 -> [w1017]
              tunnel: w869 -> [w1015]
              tunnel: w868 -> [w1014]
              tunnel: [w1015] -> w866
              tunnel: [w1014] -> w865
              tunnel: w862 -> [w1011]
              tunnel: [w1011] -> w861
              tunnel: w866 -> [w1051]
              tunnel: w865 -> [w1050]
              tunnel: w861 -> [w1049]
              tunnel: [w1051] -> w860
              tunnel: [w1050] -> w859
              tunnel: w860 -> [w1055]
              tunnel: w859 -> [w1054]
              tunnel: w858 -> [w1060]
              tunnel: w857 -> [w1059]
              tunnel: w856 -> [w1058]
              tunnel: w854 -> [w1053]
              tunnel: w855 -> [w1057]
              tunnel: [w1056] -> w853
              tunnel: [w1055] -> w852
              tunnel: [w1054] -> w851
              frame #0 {
                n368 = while {
                  tunnel: [w909] -> w892
                  tunnel: w891 -> [w908]
                  tunnel: [w901] -> w893
                  tunnel: w894 -> [w899]
                  tunnel: w896 -> [w898]
                  tunnel: w895 -> [w897]
                  i -> [w900]
                  stop <- w902 stop-if-true
                  # "Attemp to Read Until\nMax Read Tx Attemps Limit"
                  n369 = call "ReadServo_R3.vi"("DIO Ref In"=w897, "VISA resource name out"=w898, "Servo ID"=w908) -> ("Error"=w905:u8, "Valid Checksum"=w906:bool, "Current Position"=w909:u64)  [unwired: 6 in]
                  n370 = Increment(x=w900) -> (x+1=w903:i32)
                  n371 = Equal To 0?(x=w905) -> (x = 0?=w907:bool)
                  n372 = Greater Or Equal?(x=w903, y=w899) -> (x >= y?=w904:bool)
                  n373 = And(x=w906, y=w907) -> (x .and. y?=w901:bool)
                  n374 = Or(x=w901, y=w904) -> (x .or. y?=w902:bool)
                }
              }
              frame #1 {
                # "Read Position First"
                n375 = local read "Servo Goal Position\n - Left"() -> (w912:u16)
                n376 = case shown="True" w915 {
                  tunnel: w914 -> [_ w920]
                  tunnel: w912 -> [_ w918]
                  frame False {
                  }
                  frame True {
                    # "Convert Received Position to Angle Relative to Robot"
                    # "45 DEG MOUNT OFFSET"
                    # "1024/300"
                    n377 = local write "Current L (10bit)"(w920) -> ()
                    n378 = To Word Integer(number=w920) -> (16bit integer=w924:i16)
                    n379 = To Word Integer(number=w918) -> (16bit integer=w923:i16)
                    n380 = Subtract(x=w923, y=w924) -> (x-y=w922:i16)
                    n381 = Divide(x=w920, y=3.413333333333333) -> (x/y=w928:dbl)
                    n382 = Absolute Value(x=w922) -> (abs(x)=w921:i16)
                    n383 = Subtract(x=w928, y=sgl 60.0) -> (x-y=w926:dbl)
                    n384 = Greater?(x=w921, y=u16 5) -> (0:w917:bool)
                    n385 = Add(x=w926, y=sgl 45.0) -> (x+y=w916:dbl)
                    n386 = local write "Move Servo - L"(w917) -> ()
                    n387 = local write "Servo Moving - L"(w917) -> ()
                    n388 = local write "Current Angle\n - Left (internal)"(w916) -> ()
                    n389 = shared-variable "RT myRIO Target - Overlord\\Localization_Variables_r0.lvlib\\Left Servo Angle_Current"(w916) -> ()  [unwired: 1 in, 1 out]
                  }
                }
              }
              frame #2 {
                n390 = local read "Move Servo - L"() -> (w933:bool)
                n391 = case shown="True" w933 {
                  tunnel: w936 -> [_ w951]
                  tunnel: w930 -> [_ w938]
                  tunnel: [TRUE w949] -> w934
                  tunnel: w935 -> [_ w941]
                  tunnel: w932 -> [_ w940]
                  tunnel: w931 -> [_ w939]
                  frame False {
                    # "Only Send if Current Position is far enough"
                  }
                  frame True {
                    w947 = 1
                    # "High Byte"
                    # "Low Byte"
                    n392 = Type Cast(type="", x=w938) -> (*(type *) &x=w948:string)
                    n393 = local write "Servo Moving - L"(TRUE) -> ()
                    n394 = String Subset(string=w948, offset (0)=1, length (rest)=w947) -> (substring=w943:string)
                    n395 = String Subset(string=w948, offset (0)=0, length (rest)=w947) -> (substring=w942:string)
                    n396 = while {
                      tunnel: w951 -> [w965]
                      tunnel: [w957] -> w949
                      tunnel: w943 -> [w961]
                      tunnel: w942 -> [w960]
                      tunnel: w941 -> [w954]
                      tunnel: w940 -> [w953]
                      tunnel: w939 -> [w952]
                      i -> [w955]
                      stop <- w956 stop-if-true
                      # "Attemp to Write Until\nMax Write Tx Attemps Limit"
                      n397 = call "MoveServo_R3.vi"("DIO Ref Out"=w952, "VISA resource name out"=w953, "GP - Low Byte"=w961, "GP - High Byte"=w960, "Servo ID"=w965) -> ("Valid Checksum"=w962:bool, "Error"=w964:u64)  [unwired: 5 in]
                      n398 = Equal To 0?(x=w964) -> (x = 0?=w963:bool)
                      n399 = And(x=w962, y=w963) -> (x .and. y?=w957:bool)
                      n400 = Increment(x=w955) -> (x+1=w959:i32)
                      n401 = Greater Or Equal?(x=w959, y=w954) -> (x >= y?=w958:bool)
                      n402 = Or(x=w957, y=w958) -> (x .or. y?=w956:bool)
                    }
                  }
                }
                n403 = case shown="True" w934 {
                  frame False {
                  }
                  frame True {
                    # "Update Servo flag"
                    n404 = local write "Move Servo - L"(FALSE) -> ()
                  }
                }
              }
              frame #3 {
                n405 = call "Wait2"("Count(mSec)"="Servo Comm\nWait Time - (ms)") -> ()  [unwired: 1 out]
              }
              frame #4 {
                n406 = while {
                  tunnel: [w989] -> w975
                  tunnel: w970 -> [w988]
                  tunnel: [w981] -> w974
                  tunnel: w976 -> [w979]
                  tunnel: w973 -> [w978]
                  tunnel: w972 -> [w977]
                  i -> [w980]
                  stop <- w982 stop-if-true
                  # "Attemp to Read Until\nMax Read Tx Attemps Limit"
                  n407 = call "ReadServo_R3.vi"("DIO Ref In"=w977, "VISA resource name out"=w978, "Servo ID"=w988) -> ("Error"=w985:u8, "Valid Checksum"=w986:bool, "Current Position"=w989:u64)  [unwired: 6 in]
                  n408 = Increment(x=w980) -> (x+1=w983:i32)
                  n409 = Equal To 0?(x=w985) -> (x = 0?=w987:bool)
                  n410 = Greater Or Equal?(x=w983, y=w979) -> (x >= y?=w984:bool)
                  n411 = And(x=w986, y=w987) -> (x .and. y?=w981:bool)
                  n412 = Or(x=w981, y=w984) -> (x .or. y?=w982:bool)
                }
              }
              frame #5 {
                n413 = local read "Servo Goal Position\n - Right"() -> (w993:u16)
                n414 = case shown="True" w995 {
                  tunnel: w996 -> [_ w1000]
                  tunnel: w993 -> [_ w999]
                  frame False {
                    # "Don't update current position"
                  }
                  frame True {
                    # "Convert Received Position to Angle Relative to Robot"
                    # "45 DEG MOUNT OFFSET"
                    # "1024/300"
                    n415 = local write "Current R (10bit)"(w1000) -> ()
                    n416 = Divide(x=w1000, y=3.413333333333333) -> (x/y=w1009:dbl)
                    n417 = Subtract(x=w1009, y=sgl 60.0) -> (x-y=w1007:dbl)
                    n418 = Subtract(x=w1007, y=sgl 45.0) -> (x-y=w997:dbl)
                    n419 = To Word Integer(number=w999) -> (16bit integer=w1004:i16)
                    n420 = To Word Integer(number=w1000) -> (16bit integer=w1005:i16)
                    n421 = shared-variable "RT myRIO Target - Overlord\\Localization_Variables_r0.lvlib\\Right Servo Angle_Current"(w997) -> ()  [unwired: 1 in, 1 out]
                    n422 = local write "Current Angle\n - Right (internal)"(w997) -> ()
                    n423 = Subtract(x=w1004, y=w1005) -> (x-y=w1003:i16)
                    n424 = Absolute Value(x=w1003) -> (abs(x)=w1002:i16)
                    n425 = Greater?(x=w1002, y=u16 5) -> (0:w998:bool)
                    n426 = local write "Move Servo - R"(w998) -> ()
                    n427 = local write "Servo Moving - R"(w998) -> ()
                  }
                }
              }
              frame #6 {
                n428 = local read "Move Servo - R"() -> (w1012:bool)
                n429 = case shown="True" w1012 {
                  tunnel: w1016 -> [_ w1021]
                  tunnel: w1018 -> [_ w1028]
                  tunnel: [TRUE w1029] -> w1013
                  tunnel: w1017 -> [_ w1024]
                  tunnel: w1015 -> [_ w1023]
                  tunnel: w1014 -> [_ w1022]
                  frame False {
                  }
                  frame True {
                    w1031 = 1
                    # "High Byte"
                    # "Low Byte"
                    n430 = Type Cast(type="", x=w1021) -> (*(type *) &x=w1030:string)
                    n431 = local write "Servo Moving - R"(TRUE) -> ()
                    n432 = String Subset(string=w1030, offset (0)=1, length (rest)=w1031) -> (substring=w1027:string)
                    n433 = String Subset(string=w1030, offset (0)=0, length (rest)=w1031) -> (substring=w1026:string)
                    n434 = while {
                      tunnel: [w1040] -> w1029
                      tunnel: w1028 -> [w1045]
                      tunnel: w1027 -> [w1044]
                      tunnel: w1026 -> [w1043]
                      tunnel: w1024 -> [w1038]
                      tunnel: w1023 -> [w1036]
                      tunnel: w1022 -> [w1035]
                      i -> [w1039]
                      stop <- w1037 stop-if-true
                      # "Attemp to Write Until\nMax Write Tx Attemps Limit"
                      n435 = call "MoveServo_R3.vi"("DIO Ref Out"=w1035, "VISA resource name out"=w1036, "GP - Low Byte"=w1044, "GP - High Byte"=w1043, "Servo ID"=w1045) -> ("Valid Checksum"=w1047:bool, "Error"=w1046:u64)  [unwired: 5 in]
                      n436 = Increment(x=w1039) -> (x+1=w1041:i32)
                      n437 = Greater Or Equal?(x=w1041, y=w1038) -> (x >= y?=w1042:bool)
                      n438 = Equal To 0?(x=w1046) -> (x = 0?=w1048:bool)
                      n439 = And(x=w1047, y=w1048) -> (x .and. y?=w1040:bool)
                      n440 = Or(x=w1040, y=w1042) -> (x .or. y?=w1037:bool)
                    }
                  }
                }
                n441 = case shown="True" w1013 {
                  frame False {
                  }
                  frame True {
                    # "Update Servo flag"
                    n442 = local write "Move Servo - R"(FALSE) -> ()
                  }
                }
              }
              frame #7 {
                n443 = call "Wait3"("Count(mSec)"=w1049) -> ()  [unwired: 1 out]
              }
              frame #8 {
                # "Increment Service Count"
                # "Update Compliance Slope\nEvery x loops"
                n444 = Equal?(x=w1053, y=u16 1000) -> (x = y?=w1062:bool)
                n445 = case shown="True" w1062 {
                  tunnel: w1058 -> [_ w1072]
                  tunnel: w1055 -> [_ w1071]
                  tunnel: w1054 -> [_ w1070]
                  tunnel: w1055 -> [_ w1069]
                  tunnel: w1054 -> [_ w1068]
                  tunnel: w1060 -> [_ w1067]
                  tunnel: w1059 -> [_ w1066]
                  tunnel: w1053 -> [w1063 _]
                  tunnel: [w1063 u16 0] -> w1061
                  tunnel: w1057 -> [_ w1064]
                  frame False {
                  }
                  frame True {
                    # "Reset Service\nCount"
                    n446 = flat-sequence {
                      tunnel: w1071 -> [w1077]
                      tunnel: w1070 -> [w1076]
                      tunnel: w1067 -> [w1078]
                      tunnel: [w1074] -> w1073
                      tunnel: w1072 -> [w1075]
                      tunnel: w1064 -> [w1074]
                      tunnel: w1066 -> [w1090]
                      tunnel: w1073 -> [w1089]
                      tunnel: w1072 -> [w1088]
                      tunnel: w1069 -> [w1087]
                      tunnel: w1068 -> [w1086]
                      frame #0 {
                        n447 = while {
                          tunnel: w1074 -> [w1085]
                          tunnel: w1077 -> [w1083]
                          tunnel: w1076 -> [w1082]
                          tunnel: w1078 -> [w1081]
                          tunnel: w1075 -> [w1080]
                          i -> [w1079]
                          stop <- w1084 stop-if-true
                          n448 = call "Set_Compliance_Slope_R2.vi"("Compliance Slope"=w1080, "DIO Ref Out"=w1082, "VISA resource name"=w1083, "Servo ID"=w1081) -> ()  [unwired: 6 in, 2 out]
                          n449 = Greater Or Equal?(x=w1079, y=w1085) -> (x >= y?=w1084:bool)
                        }
                      }
                      frame #1 {
                        n450 = while {
                          tunnel: w1089 -> [w1097]
                          tunnel: w1090 -> [w1095]
                          tunnel: w1087 -> [w1094]
                          tunnel: w1086 -> [w1093]
                          tunnel: w1088 -> [w1092]
                          i -> [w1091]
                          stop <- w1096 stop-if-true
                          n451 = call "Set_Compliance_Slope_R2.vi"("Compliance Slope"=w1092, "DIO Ref Out"=w1093, "VISA resource name"=w1094, "Servo ID"=w1095) -> ()  [unwired: 6 in, 2 out]
                          n452 = Greater Or Equal?(x=w1091, y=w1097) -> (x >= y?=w1096:bool)
                        }
                      }
                    }
                  }
                }
                n453 = Increment(x=w1061) -> (x+1=w1056:u16)
              }
            }
          }
        }
      }
    }
    frame #2 {
      n454 = VISA Close(VISA resource name=w1099) -> ()  [unwired: 1 in, 1 out]
      n455 = call <vilib>:"Close.vi"("DIO Ref In"=w1098) -> ()  [unwired: 10 in, 1 out]
    }
  }
  n456 = while {
    stop <- FALSE stop-if-true
    n457 = call "Wait9"("Count(mSec)"=u32 1000) -> ()  [unwired: 1 out]
  }
  n458 = while {
    shift-right: [w1160] -> _
    shift-left: "Initial Main State - Left" -> [w1185]
    shift-right: [w1152] -> _
    shift-left: "Search Direction - in - L" -> [w1179]
    shift-right: [w1151] -> _
    shift-left: FALSE -> [w1178]
    shift-right: [w1154] -> _
    shift-left: w13 -> [w1153]
    shift-right: [w1155] -> _
    shift-left: w13 -> [w1172]
    shift-right: [w1156] -> _
    shift-left: w13 -> [w1177]
    shift-right: [w1157] -> _
    shift-left: w13 -> [w1171]
    shift-right: [w1158] -> _
    shift-left: w13 -> [w1170]
    shift-right: [w1103] -> _
    shift-left: "Search Direction - in - Right" -> [w1127]
    shift-right: [w1148] -> _
    shift-left: FALSE -> [w1125]
    shift-right: [w1149] -> _
    shift-left: w12 -> [w1116]
    shift-right: [w1104] -> _
    shift-left: w12 -> [w1115]
    shift-right: [w1105] -> _
    shift-left: w12 -> [w1122]
    shift-right: [w1106] -> _
    shift-left: w12 -> [w1124]
    shift-right: [w1107] -> _
    shift-left: w12 -> [w1123]
    shift-right: [w1114] -> _
    shift-left: "Initial Main State- Right" -> [w1139]
    shift-right: [w1144] -> _
    shift-left: 0 -> [w1146]
    shift-right: [w1111] -> _
    shift-left: 0 -> [w1131]
    shift-right: [w1143] -> _
    shift-left: "Initial Tracking State - Left" -> [w1145]
    shift-right: [w1109] -> _
    shift-left: "Initial Tracking State - Right" -> [w1137]
    shift-right: [w1110] -> _
    shift-left: "Initial Recovery State  - Right" -> [w1138]
    shift-right: [w1141] -> _
    shift-left: "Initial Recovery State - L" -> [w1142]
    stop <- FALSE stop-if-true
    w1164 = T2."Tracking" ("Next Main State")
    # "Wait for New"
    # "ADD TRACKING TIMEOUT COUNT**********************"
    # "Service Track Angle Flag"
    # "Add Logic to Have Search Directions\nopposite if Both Searching"
    # "REMOVE LAST GOAL POSITION WITH cURRENT"
    # "Go to Current State"
    # "Add Logic to Have Search Directions\nopposite if Both Searching"
    # "Manuallly Reset\nRespond Var"
    # "Manuallly Reset\nRespond Var"
    # "Update Comm Process Variables"
    # "Both Tracking"
    # "Current delta - L"
    # "delta move sum - R"
    # "delta move sum - L"
    # "Current delta - R"
    # "Service Move Respond Variables"
    n459 = local read "Min Num Frames\nper Search"() -> (w1150:i32)
    n460 = local read "Minimum Delta \nServo Threshold"() -> (w1169:i16)
    n461 = local read "Maximum Move \nServo Threshold"() -> (w1168:i16)
    n462 = local read "Middle Beacon\nCoordinates"() -> (w1117:cluster{"X":sgl, "Y":sgl})
    n463 = local read "Position \nLock Status"() -> (w1176:bool)
    n464 = local read "Position \nLock Status"() -> (w1120:bool)
    n465 = local read "Search Step Size"() -> (w1167:u16)
    n466 = local read "Last Orientation"() -> (w1174:sgl)
    n467 = local read "Last Orientation"() -> (w1118:sgl)
    n468 = local read "Last Position"() -> (w1175:cluster{"X":sgl, "Y":sgl})
    n469 = local read "Last Position"() -> (w1119:cluster{"X":sgl, "Y":sgl})
    n470 = local read "Min Num Frames\nper Search"() -> (w1121:i32)
    n471 = call "Wait"("Count(mSec)"="Servo Algorithm\nCycle Time(ms)") -> ()  [unwired: 1 out]
    n472 = local read "Minimum Delta \nServo Threshold"() -> (w1129:i16)
    n473 = local read "Maximum Move \nServo Threshold"() -> (w1128:i16)
    n474 = local read "Search Step Size"() -> (w1126:u16)
    n475 = local read "New Data  Flag\nRight Servo"() -> (w1134:bool)
    n476 = local read "New Data  Flag\nLeft Servo"() -> (w1140:bool)
    n477 = local read "Image Lock - Right"() -> (w1136:bool)
    n478 = local read "Image Lock - Left"() -> (w1184:bool)
    n479 = local read "Tracking Angle - Right"() -> (w1133:sgl)
    n480 = local read "Tracking Angle - Left"() -> (w1182:sgl)
    n481 = local read "Current R (10bit)"() -> (w1132:u16)
    n482 = local read "Current L (10bit)"() -> (w1181:u16)
    n483 = case shown="True" w1134 {
      tunnel: [w1212 w1250] -> w1102
      tunnel: [w1206 w1249] -> w1113
      tunnel: w1139 -> [w1207 w1248]
      tunnel: w1136 -> [_ w1247]
      tunnel: "Track Angle Valid  - Right" -> [_ w1246]
      tunnel: w1133 -> [_ w1245]
      tunnel: w1132 -> [w1212 w1244]
      tunnel: "Mounting Offset - Right" -> [_ w1243]
      tunnel: w1127 -> [w1203 w1242]
      tunnel: w1125 -> [_ w1241]
      tunnel: w1122 -> [w1204 w1240]
      tunnel: w1120 -> [_ w1239]
      tunnel: w1119 -> [_ w1238]
      tunnel: w1118 -> [_ w1237]
      tunnel: w1117 -> [_ w1236]
      tunnel: w1115 -> [w1202 w1235]
      tunnel: w1124 -> [w1201 w1234]
      tunnel: w1123 -> [w1205 w1233]
      tunnel: w1129 -> [_ w1232]
      tunnel: w1128 -> [_ w1231]
      tunnel: w1126 -> [_ w1230]
      tunnel: [0 w1229] -> w1112
      tunnel: [w1207 w1228] -> w1114
      tunnel: [w1206 w1227] -> w1108
      tunnel: [w1205 w1226] -> w1107
      tunnel: [w1201 w1225] -> w1106
      tunnel: [w1204 w1224] -> w1105
      tunnel: [w1202 w1223] -> w1104
      tunnel: w1116 -> [_ w1222]
      tunnel: [w1203 w1221] -> w1103
      tunnel: w1121 -> [_ w1220]
      tunnel: w1131 -> [w1210 w1219]
      tunnel: w1137 -> [w1209 w1218]
      tunnel: [w1210 w1217] -> w1111
      tunnel: [w1209 w1216] -> w1109
      tunnel: w1138 -> [w1208 w1215]
      tunnel: [w1208 w1214] -> w1110
      frame False {
        w1206 = FALSE
        # "Recovery Mode COunt"
        # "Frames Processed - L"
        # "Recovery Search move Count - L"
        # "Recovery Search Attempt Count- L"
        # "WAITING FOR NEW IMAGE, RETAIN ALL VALUES"
      }
      frame True {
        w1252 = u16 1023
        w1255 = u16 0
        # "New Tracking State"
        # "Tracking Timeout Count"
        # "Next Main State"
        # "Next Recovery State"
        # "Reset Respond"
        # "Search Direction"
        # "Recovery Count"
        # "Recovery Search move Count"
        # "Recovery Search Attempt Count"
        # "Frames Processed"
        # "Apply Floor/Ceiling to Goal Position"
        # "Current move Delta"
        # "Service Track Angle Flag"
        # "Move Servo"
        # "Goal Position"
        # "Go to Current State"
        n484 = case shown="\"Recovery Mode\"" w1248 {
          tunnel: w1244 -> [w1274 w1351 w1529]
          tunnel: w1245 -> [_ w1353 _]
          tunnel: w1230 -> [w1273 _ w1524]
          tunnel: w1242 -> [w1272 w1333 w1518]
          tunnel: [w1271 w1349 w1528] -> w1256
          tunnel: [w1269 w1350 w1527] -> w1249
          tunnel: w1246 -> [w1267 w1344 w1505]
          tunnel: [w1266 w1346 w1514] -> w1228
          tunnel: w1247 -> [w1265 w1345 w1504]
          tunnel: w1243 -> [_ w1354 w1525]
          tunnel: w1232 -> [_ w1352 _]
          tunnel: [w1259 w1348 w1509] -> w1229
          tunnel: w1231 -> [_ w1347 _]
          tunnel: w1240 -> [w1264 _ w1519]
          tunnel: [enum16{"Generic Sweep", "Recovery Search"}."Recovery Search" enum16{"Generic Sweep", "Recovery Search"}."Recovery Search" w1526] -> w1214
          tunnel: w1235 -> [_ _ w1523]
          tunnel: w1215 -> [_ _ w1506]
          tunnel: w1241 -> [_ w1330 w1535]
          tunnel: w1222 -> [_ w1335 w1530]
          tunnel: w1237 -> [_ w1337 w1532]
          tunnel: w1238 -> [_ w1338 w1533]
          tunnel: w1239 -> [_ w1339 w1534]
          tunnel: w1236 -> [_ w1336 w1531]
          tunnel: [FALSE w1332 w1507] -> w1227
          tunnel: w1220 -> [w1263 _ w1517]
          tunnel: [w1259 w1327 w1516] -> w1223
          tunnel: [w1259 w1327 w1522] -> w1226
          tunnel: [w1259 w1327 w1521] -> w1225
          tunnel: [w1262 w1328 w1520] -> w1224
          tunnel: w1234 -> [_ _ w1512]
          tunnel: w1233 -> [_ _ w1511]
          tunnel: [w1260 w1333 w1510] -> w1221
          tunnel: w1219 -> [_ w1343 _]
          tunnel: [w1259 w1334 w1509] -> w1217
          tunnel: w1218 -> [_ w1340 _]
          tunnel: [enum16{"Track", "Reactive Predict", ""}."Track" ("Initial Tracking State - Right") w1331 enum16{"Track", "Reactive Predict", ""}."Track" ("Initial Tracking State - Right")] -> w1216
          frame "Start Up Search", Default {
            w1259 = u16 0
            # "Search Direction"
            # "Wait for 'x' Images to be Processed\nBefore Going to Next Step"
            # "Next Main State"
            # "New Goal Position"
            # "Move Servo"
            # "Choose Next State"
            # "Frames Processed Count"
            n485 = Greater Or Equal?(x=w1264, y=w1263) -> (x >= y?=w1270:bool)
            n486 = case shown="True" w1270 {
              tunnel: w1274 -> [w1289 w1301]
              tunnel: w1273 -> [_ w1299]
              tunnel: w1272 -> [w1288 w1298]
              tunnel: [w1289 w1295] -> w1271
              tunnel: [w1287 0] -> w1262
              tunnel: [FALSE TRUE] -> w1268
              tunnel: w1264 -> [w1290 _]
              tunnel: [w1288 w1292] -> w1260
              frame False {
                # "Increase Frames\nProcessed Count"
                n487 = Increment(x=w1290) -> (x+1=w1287:i32)
              }
              frame True {
                # "Reset Frames\nProcessed Count"
                # "SWEEP SEARCH - Startup"
                # "Multiple New Step\nby Step SIze"
                # "F = CCW\nT = CW"
                # "Last Direction"
                # "Min Step"
                # "add 10 in case\nactual position\nis lower than GP"
                # "Set New Step #"
                # "Choose Direction"
                # "Nearest step"
                # "Adjust Actual Posiiton\n to pre-determiend steps"
                # "Move Servo 1 \"Step\" to\nSearch"
                n488 = Add(x=3, y=w1301) -> (x+y=w1307:i32)
                n489 = Quotient & Remainder(x=w1307, y=w1299) -> (floor(x/y)=w1305:i32)  [unwired: 1 out]
                n490 = To Byte Integer(number=w1305) -> (8bit integer=w1296:i8)
                n491 = Less?(x=w1296, y=1) -> (x < y?=w1302:bool)
                n492 = case shown="False" w1302 {
                  tunnel: w1296 -> [w1318 w1326]
                  tunnel: [w1320 FALSE] -> w1292
                  tunnel: [w1319 w1326] -> w1304
                  tunnel: w1298 -> [w1317 _]
                  tunnel: w1299 -> [w1315 _]
                  frame False {
                    # "Max Step"
                    # "# of steps\nminus 1"
                    n493 = Divide(x=1024, y=w1315) -> (x/y=w1312:dbl)
                    n494 = To Unsigned Byte Integer(number=w1312) -> (unsigned 8bit integer=w1313:u8)
                    n495 = Greater Or Equal?(x=w1318, y=w1313) -> (x >= y?=w1314:bool)
                    n496 = case shown="True" w1314 {
                      tunnel: [w1321 TRUE] -> w1320
                      tunnel: [w1322 w1323] -> w1319
                      tunnel: w1318 -> [w1322 w1323]
                      tunnel: w1317 -> [w1321 _]
                      frame False {
                        # "No Need to\nChange Direction"
                      }
                      frame True {
                        # "T"
                        # "Move CW"
                      }
                    }
                  }
                  frame True {
                    # "F"
                    # "Move CCW"
                  }
                }
                n497 = case shown="False" w1292 {
                  tunnel: w1304 -> [w1309 w1310]
                  tunnel: [w1308 w1311] -> w1300
                  frame False {
                    # "CCW\n+1"
                    n498 = Increment(x=w1309) -> (x+1=w1308:i8)
                  }
                  frame True {
                    # "CW\n-1"
                    n499 = Decrement(x=w1310) -> (x-1=w1311:i8)
                  }
                }
                n500 = Multiply(x=w1300, y=w1299) -> (x*y=w1297:u16)
                n501 = To Unsigned Word Integer(number=w1297) -> (unsigned 16bit integer=w1295:u16)
              }
            }
            n502 = case shown="False" w1267 {
              tunnel: [w1278 FALSE] -> w1269
              tunnel: w1268 -> [w1278 _]
              tunnel: [w1279 w1284] -> w1266
              tunnel: w1265 -> [_ w1282]
              frame False {
                # "Check other Servo\nStay in Startup  State"
                n503 = local read "Track Angle Valid - Left"() -> (w1275:bool)
                n504 = local read "Image Lock - Left"() -> (w1276:bool)
                n505 = Or(x=w1275, y=w1276) -> (x .or. y?=w1277:bool)
                n506 = case shown="True" w1277 {
                  tunnel: [T2."Start Up Search" ("Next Main State") T2."Recovery Mode" ("Next Main State")] -> w1279
                  frame False {
                  }
                  frame True {
                  }
                }
              }
              frame True {
                # "Override Move Servo\nCommand bc an Angle Was Found\nduring this Step"
                # "Transition to Tracking State When\nImage Processing has Locked"
                n507 = case shown="False" w1282 {
                  tunnel: [T2."Start Up Search" ("Next Main State") T2."Tracking" ("Next Main State")] -> w1284
                  frame False {
                  }
                  frame True {
                  }
                }
              }
            }
          }
          frame "Tracking" {
            w1327 = 0
            # "Frames Processed Count"
            # "Image Lock - L"
            # "Track Angle Valid"
            # "Tracking Angle"
            # "Tracking Timeout Count"
            # "Max ove delta"
            # "Move delta threshold"
            # "mount offset"
            # "Current Position"
            # "Move Respond"
            # "Trackin Timeout count"
            # "Move Servo"
            # "delta"
            # "GP"
            # "Reset Move Respond"
            # "New Tracking State"
            # "Delta Move Sum"
            # "Choose Next State"
            n508 = case shown="\"Reactive Predict\"" w1340 {
              tunnel: w1354 -> [w1372 _]
              tunnel: w1353 -> [w1371 _]
              tunnel: w1352 -> [w1370 _]
              tunnel: w1351 -> [w1369 w1427]
              tunnel: [w1368 w1425] -> w1350
              tunnel: [w1367 w1433] -> w1349
              tunnel: [w1366 0] -> w1348
              tunnel: w1347 -> [w1365 _]
              tunnel: w1345 -> [w1364 w1417]
              tunnel: w1344 -> [w1363 w1420]
              tunnel: w1343 -> [w1362 w1422]
              tunnel: w1339 -> [_ w1432]
              tunnel: w1338 -> [_ w1431]
              tunnel: w1337 -> [_ w1430]
              tunnel: w1336 -> [_ w1429]
              tunnel: w1330 -> [_ w1428]
              tunnel: w1335 -> [_ w1426]
              tunnel: [TRUE w1423] -> w1332
              tunnel: [w1359 w1421] -> w1334
              tunnel: [w1357 w1419] -> w1331
              tunnel: [0 0] -> w1328
              frame "Track", Default {
                # "Reset"
                # "Tracking Timeout"
                # "Move Delta"
                # "Goal Position"
                # "Tracking Move"
                # "Move Servo"
                # "Only Consider Tracking Angle\n\nIF\n\nImage Locked        == T\nTrack Angle Flag   == T"
                n509 = And(x=w1364, y=w1363) -> (x .and. y?=w1356:bool)
                n510 = case shown="True" w1356 {
                  tunnel: w1372 -> [_ w1378]
                  tunnel: w1371 -> [_ w1396]
                  tunnel: w1370 -> [_ w1393]
                  tunnel: w1369 -> [w1375 w1383]
                  tunnel: [w1375 w1392] -> w1367
                  tunnel: [w1377 w1391] -> w1368
                  tunnel: [w1377 w1390] -> _
                  tunnel: [u16 0 w1389] -> w1366
                  tunnel: w1365 -> [_ w1385]
                  tunnel: w1362 -> [w1374 _]
                  tunnel: [w1373 0] -> w1359
                  frame False {
                    w1377 = FALSE
                    # "Increment timeout"
                    n511 = Increment(x=w1374) -> (x+1=w1373:i32)
                  }
                  frame True {
                    # "Convert Track Angle to UINT16"
                    # "1024/300"
                    # "Move to Tracking Angle \n\nif delta is greater than move servo threshold\nAND less than max move threshold"
                    n512 = Add(x=w1396, y=w1378) -> (x+y=w1399:sgl)
                    n513 = Add(x=w1399, y=sgl 60.0) -> (x+y=w1398:sgl)
                    n514 = Multiply(x=3.413333333333333, y=w1398) -> (x*y=w1379:dbl)
                    n515 = To Word Integer(number=w1383) -> (16bit integer=w1381:i16)
                    n516 = To Unsigned Word Integer(number=w1379) -> (unsigned 16bit integer=w1395:u16)
                    n517 = To Word Integer(number=w1379) -> (16bit integer=w1394:i16)
                    n518 = Subtract(x=w1394, y=w1381) -> (x-y=w1384:i16)
                    n519 = Absolute Value(x=w1384) -> (abs(x)=w1380:i16)
                    n520 = Greater Or Equal?(x=w1380, y=w1393) -> (x >= y?=w1387:bool)
                    n521 = Less Or Equal?(x=w1380, y=w1385) -> (x <= y?=w1386:bool)
                    n522 = And(x=w1387, y=w1386) -> (x .and. y?=w1388:bool)
                    n523 = case shown="True" w1388 {
                      tunnel: w1395 -> [_ w1407]
                      tunnel: [w1402 w1407] -> w1392
                      tunnel: [w1403 w1413] -> w1391
                      tunnel: [w1403 w1413] -> w1390
                      tunnel: w1383 -> [w1402 _]
                      tunnel: w1380 -> [_ w1412]
                      tunnel: [u16 0 w1412] -> w1389
                      tunnel: w1378 -> [_ w1406]
                      frame False {
                        w1403 = FALSE
                        # "Don't Move"
                      }
                      frame True {
                        w1413 = TRUE
                        # "45 DEG MOUNT OFFSET"
                        # "1024/300"
                        # "Current Delta"
                        # "Use new Track Angle"
                        n524 = Divide(x=w1407, y=3.413333333333333) -> (x/y=w1409:dbl)
                        n525 = Negate(x=w1406) -> (-x=w1405:sgl)
                        n526 = Subtract(x=w1409, y=sgl 60.0) -> (x-y=w1411:dbl)
                        n527 = Add(x=w1411, y=w1405) -> (x+y=w1404:dbl)
                        n528 = local write "Last Track Angle - R"(w1404) -> ()
                      }
                    }
                  }
                }
                n529 = local read "Timeout to \nEnable Reactive Predict"() -> (w1360:u16)
                n530 = Less?(x=w1359, y=w1360) -> (x < y?=w1358:bool)
                n531 = case shown="False" w1358 {
                  tunnel: [enum16{"Track", "Reactive Predict", ""}."Reactive Predict" ("Initial Tracking State - Right") enum16{"Track", "Reactive Predict", ""}."Track" ("Initial Tracking State - Right")] -> w1357
                  frame False {
                  }
                  frame True {
                  }
                }
              }
              frame "Reactive Predict" {
                # "Choose New\nTracking State"
                n532 = Or(x=w1417, y=w1420) -> (x .or. y?=w1416:bool)
                n533 = case shown="False" w1416 {
                  tunnel: [w1446 w1498] -> w1433
                  tunnel: w1432 -> [w1445 _]
                  tunnel: w1431 -> [w1444 _]
                  tunnel: w1430 -> [w1443 _]
                  tunnel: w1429 -> [w1442 _]
                  tunnel: w1428 -> [w1441 _]
                  tunnel: w1426 -> [w1440 _]
                  tunnel: [w1439 w1497] -> w1425
                  tunnel: [w1438 w1497] -> w1423
                  tunnel: w1422 -> [w1437 _]
                  tunnel: [w1436 0] -> w1421
                  tunnel: [enum16{"Track", "Reactive Predict", ""}."Reactive Predict" ("Initial Tracking State - Right") enum16{"Track", "Reactive Predict", ""}."Track" ("Initial Tracking State - Right")] -> w1419
                  tunnel: w1427 -> [w1434 w1498]
                  frame False {
                    # "Stay in Reactive State"
                    # "Increment Track Timeout"
                    # "Move Respond Flag"
                    n534 = Increment(x=w1437) -> (x+1=w1436:i32)
                    n535 = case shown="True" w1441 {
                      tunnel: w1445 -> [_ w1461]
                      tunnel: w1444 -> [_ w1460]
                      tunnel: w1443 -> [_ w1459]
                      tunnel: w1442 -> [_ w1458]
                      tunnel: w1440 -> [_ w1455]
                      tunnel: [w1447 w1451] -> w1446
                      tunnel: [w1448 w1450] -> w1439
                      tunnel: [w1448 w1450] -> w1438
                      tunnel: w1434 -> [w1447 w1449]
                      frame False {
                        w1448 = FALSE
                        # "Reset Move Respond = F"
                        # "Move Servo = F"
                      }
                      frame True {
                        w1450 = TRUE
                        # "Position Lock"
                        # "Current Servo\nPosition"
                        # "Reset Move\nRespond = T"
                        # "Move Servo = T"
                        # "Apply Direction \nto Offset (delta sum)"
                        # "Check Last Known Position of Robot"
                        n536 = case shown="True" w1461 {
                          tunnel: w1460 -> [_ w1489]
                          tunnel: w1459 -> [_ w1464]
                          tunnel: w1458 -> [_ w1465]
                          tunnel: [sgl 1.0 ("y") w1463] -> w1457
                          frame False {
                            # "No Position Data Available"
                            # "Default is to move\nSame Direction as other\nServo"
                          }
                          frame True {
                            w1470 = sgl 1.0 ("y")
                            # "Use previous position/orientation to Guess Which Direction to Move Servo"
                            # "Choose Search Direction"
                            # "\"Perpendicular \nThreshold\""
                            # "If Orientation is\n ~Perpendicular -> Start Search\n in Opposite Direction of Other"
                            # "****add 90 until orientation angle is fixed"
                            # "Last Orientation"
                            # "Convert to Rad"
                            # "Avoid Divide by 0"
                            # "-1/m"
                            # "Calculate Normal Line to \nLast Robot Position\nfrom Center Beacon"
                            # "last Position \nCoordinates"
                            n537 = Unbundle(w1489) -> ("X"=w1469:sgl, "Y"=w1468:sgl)
                            n538 = Unbundle(w1465) -> ("X"=w1467:sgl, "Y"=w1466:sgl)
                            n539 = Subtract(x=w1468, y=w1466) -> (x-y=w1485:sgl)
                            n540 = Subtract(x=w1469, y=w1467) -> (x-y=w1483:sgl)
                            n541 = Equal To 0?(x=w1483) -> (x = 0?=w1484:bool)
                            n542 = case shown="False" w1484 {
                              tunnel: w1485 -> [w1492 _]
                              tunnel: w1483 -> [w1491 _]
                              tunnel: [w1490 1000000000000000.0] -> w1482
                              frame False {
                                n543 = Divide(x=w1492, y=w1491) -> (x/y=w1490:sgl)
                              }
                              frame True {
                              }
                            }
                            n544 = Equal To 0?(x=w1482) -> (x = 0?=w1487:bool)
                            n545 = case shown="False" w1487 {
                              tunnel: [w1494 1e-08] -> w1486
                              tunnel: w1482 -> [w1494 _]
                              frame False {
                              }
                              frame True {
                                # "Can't have infinit slope"
                              }
                            }
                            n546 = Divide(x=-1.0, y=w1486) -> (x/y=w1481:dbl)
                            n547 = Inverse Tangent(1:w1481) -> (0:w1479:dbl)
                            n548 = expression code="(x/pi)*180.0" "radians to degrees"(w1479) -> (w1480:dbl)
                            n549 = To Single Precision Float(number=w1480) -> (single precision float=w1477:sgl)
                            n550 = Add(x=w1464, y=sgl 90.0) -> (x+y=w1476:sgl)
                            n551 = Subtract(x=w1477, y=w1476) -> (x-y=w1475:sgl)
                            n552 = Absolute Value(x=w1475) -> (abs(x)=w1474:sgl)
                            n553 = Less Or Equal?(x=w1474, y=sgl 10.0) -> (x <= y?=w1472:bool)
                            n554 = Negate(x=w1470) -> (-x=w1471:sgl)
                            n555 = Select(t=w1471, s=w1472, f=w1470) -> (s? t:f=w1463:sgl)
                          }
                        }
                        n556 = To Word Integer(number=w1457) -> (16bit integer=w1456:i16)
                        n557 = Multiply(x=w1456, y=w1455) -> (x*y=w1454:i32)
                        n558 = To Word Integer(number=w1449) -> (16bit integer=w1453:i16)
                        n559 = Add(x=w1454, y=w1453) -> (x+y=w1452:i32)
                        n560 = To Unsigned Word Integer(number=w1452) -> (unsigned 16bit integer=w1451:u16)
                      }
                    }
                  }
                  frame True {
                    w1497 = TRUE
                    # "Go Directly to Track State"
                  }
                }
              }
            }
            n561 = local read "Tracking Timeout\nThreshold"() -> (w1341:i32)
            n562 = Less?(x=w1334, y=w1341) -> (x < y?=w1342:bool)
            n563 = case shown="False" w1342 {
              tunnel: [T2."Recovery Mode" ("Next Main State") T2."Tracking" ("Next Main State")] -> w1346
              frame False {
              }
              frame True {
              }
            }
          }
          frame "Recovery Mode" {
            w1509 = u16 0
            # "Increment Recovery Mode Count"
            # "Recovvery Mode\nCount"
            # "Frames Processed"
            # "Choose Next Main State"
            # "Reset recovery count"
            # "Recovery move\nCount"
            # "Recovery Search\nAttempt count"
            # "Move Servo = T"
            # "delta move sum"
            # "Robot Position Valid"
            n564 = local read "Image Lock - Left"() -> (w1513:bool)
            n565 = Or(x=w1504, y=w1505) -> (x .or. y?=w1503:bool)
            n566 = case shown="\"Recovery Search\"" w1506 {
              tunnel: w1535 -> [_ _]
              tunnel: w1534 -> [_ _]
              tunnel: w1533 -> [_ _]
              tunnel: w1532 -> [_ _]
              tunnel: w1531 -> [_ _]
              tunnel: w1530 -> [_ _]
              tunnel: w1529 -> [w1563 w1649]
              tunnel: [w1555 w1647] -> w1528
              tunnel: [w1552 w1641] -> w1527
              tunnel: [FALSE FALSE] -> w1507
              tunnel: [w1557 w1638] -> w1526
              tunnel: w1523 -> [w1561 _]
              tunnel: w1525 -> [w1564 _]
              tunnel: w1524 -> [w1562 w1644]
              tunnel: [w1554 w1637] -> w1521
              tunnel: [w1553 w1637] -> w1522
              tunnel: w1513 -> [w1551 _]
              tunnel: [w1542 w1648] -> w1520
              tunnel: w1519 -> [w1540 w1632]
              tunnel: w1518 -> [w1545 w1645]
              tunnel: w1517 -> [w1541 w1643]
              tunnel: w1504 -> [_ _]
              tunnel: w1505 -> [_ w1640]
              tunnel: [FALSE w1639] -> w1515
              tunnel: w1512 -> [w1549 _]
              tunnel: w1511 -> [w1548 _]
              tunnel: [w1545 w1636] -> w1510
              frame "Recovery Search" {
                # "Wait for 2 Images to be Processed\nBefore Going to Next Step"
                # "Choose Next Reovery State"
                # "Recovery Search \nAttempt Count"
                # "Move Servo"
                # "Goal Position"
                # "Recovery Search\nmove Count"
                # "Attempt Recovery Search if Other Servo has Valid Angle"
                n567 = local read "Last Track Angle - L"() -> (w1544:sgl)
                n568 = Greater Or Equal?(x=w1540, y=w1541) -> (x >= y?=w1543:bool)
                n569 = case shown="True" w1543 {
                  tunnel: w1564 -> [_ w1584]
                  tunnel: [w1569 w1583] -> w1553
                  tunnel: w1563 -> [w1572 w1582]
                  tunnel: w1562 -> [_ w1581]
                  tunnel: [w1570 w1580] -> w1554
                  tunnel: [w1572 w1579] -> w1555
                  tunnel: [FALSE w1578] -> w1552
                  tunnel: w1549 -> [w1570 w1577]
                  tunnel: w1548 -> [w1569 w1576]
                  tunnel: w1551 -> [_ w1575]
                  tunnel: w1544 -> [_ w1574]
                  tunnel: [w1567 0 ("Frames Processed\nCount - in")] -> w1542
                  tunnel: w1540 -> [w1568 _]
                  frame False {
                    # "Increment Frames Processed"
                    # "WAIT"
                    n570 = Increment(x=w1568) -> (x+1=w1567:i32)
                  }
                  frame True {
                    n571 = case shown="True" w1575 {
                      tunnel: w1574 -> [_ w1597]
                      tunnel: w1577 -> [w1585 w1593]
                      tunnel: w1584 -> [_ w1598]
                      tunnel: [w1588 w1596] -> w1579
                      tunnel: [w1586 w1595] -> w1583
                      tunnel: w1576 -> [w1586 w1594]
                      tunnel: w1582 -> [w1588 w1592]
                      tunnel: w1581 -> [_ w1591]
                      tunnel: [FALSE TRUE] -> w1578
                      tunnel: [w1585 w1589] -> w1580
                      frame False {
                        # "Don't Move bc Other Servo Doesn't Have Image Lock"
                      }
                      frame True {
                        # "Move Servo = T"
                        n572 = Greater Than 0?(x=w1593) -> (x > 0?=w1599:bool)
                        n573 = case shown="False" w1599 {
                          tunnel: w1598 -> [w1606 _]
                          tunnel: w1597 -> [w1600 _]
                          tunnel: [w1605 w1616] -> w1596
                          tunnel: [w1603 w1622] -> w1595
                          tunnel: w1594 -> [w1604 w1622]
                          tunnel: w1593 -> [w1602 w1619]
                          tunnel: [w1601 w1621] -> w1589
                          tunnel: w1592 -> [_ w1617]
                          tunnel: w1591 -> [_ w1614]
                          frame False {
                            # "Increment move count to transition\nto Pan mode"
                            # "Increment Recovery Search Attempt Count"
                            # "1024/300"
                            # "Move Parallel to Other Servo"
                            n574 = Increment(x=w1604) -> (x+1=w1603:i32)
                            n575 = Add(x=w1600, y=w1606) -> (x+y=w1612:sgl)
                            n576 = Add(x=w1612, y=sgl 60.0) -> (x+y=w1611:sgl)
                            n577 = Multiply(x=3.413333333333333, y=w1611) -> (x*y=w1609:dbl)
                            n578 = Add(x=0.5, y=w1609) -> (x+y=w1607:dbl)
                            n579 = To Unsigned Word Integer(number=w1607) -> (unsigned 16bit integer=w1605:u16)
                            n580 = Increment(x=w1602) -> (x+1=w1601:i32)
                          }
                          frame True {
                            # "Apply Direction"
                            # "Step SIze"
                            # "Current Position"
                            # "Attempt to Pan in Steps Towards other Servo"
                            # "Could be same or function of \nregular search step size"
                            # "Max # of Pan\nMoves"
                            # "Pan Towards Other Servo"
                            n581 = Greater Or Equal?(x=w1619, y=u16 20) -> (x >= y?=w1620:bool)
                            n582 = case shown="False" w1620 {
                              tunnel: w1619 -> [w1630 _]
                              tunnel: [w1629 u16 0] -> w1621
                              frame False {
                                # "Increment Pan Count"
                                n583 = Increment(x=w1630) -> (x+1=w1629:i32)
                              }
                              frame True {
                                # "Reset move count"
                              }
                            }
                            n584 = local read "Recovery Search\nDirection - R"() -> (w1615:bool)
                            n585 = case shown="False" w1615 {
                              tunnel: w1617 -> [w1624 w1628]
                              tunnel: w1614 -> [w1625 w1627]
                              tunnel: [w1623 w1626] -> w1616
                              frame False {
                                # "CCW"
                                n586 = Add(x=w1624, y=w1625) -> (x+y=w1623:u16)
                              }
                              frame True {
                                # "CW"
                                n587 = Subtract(x=w1628, y=w1627) -> (x-y=w1626:u16)
                              }
                            }
                          }
                        }
                      }
                    }
                  }
                }
                n588 = local read "Max Recovery Count\n(Recovery Search)"() -> (w1546:u16)
                n589 = local read "Max Recovery\nSearch Attempts"() -> (w1547:u16)
                n590 = Less Or Equal?(x=w1553, y=w1547) -> (x <= y?=w1559:bool)
                n591 = Less Or Equal?(x=w1561, y=w1546) -> (x <= y?=w1560:bool)
                n592 = And(x=w1559, y=w1560) -> (x .and. y?=w1558:bool)
                n593 = case shown="True" w1558 {
                  tunnel: [enum16{"Generic Sweep", "Recovery Search"}."Generic Sweep" enum16{"Generic Sweep", "Recovery Search"}."Recovery Search"] -> w1557
                  frame False {
                  }
                  frame True {
                  }
                }
              }
              frame "Generic Sweep" {
                w1637 = u16 0
                # "Angle Valid?"
                # "Choose Next Recovery State"
                # "Wait for 2 Images to be Processed\nBefore Going to Next Step"
                # "New Goal Position"
                # "Move Servo"
                # "Frames Processed Count"
                n594 = Greater Or Equal?(x=w1632, y=w1643) -> (x >= y?=w1650:bool)
                n595 = case shown="True" w1650 {
                  tunnel: w1649 -> [w1666 w1678]
                  tunnel: w1644 -> [_ w1676]
                  tunnel: w1645 -> [w1665 w1675]
                  tunnel: [w1666 w1672] -> w1647
                  tunnel: [w1664 0] -> w1648
                  tunnel: [FALSE TRUE] -> w1642
                  tunnel: w1632 -> [w1667 _]
                  tunnel: [w1665 w1669] -> w1636
                  frame False {
                    # "Increment Frames Processed"
                    n596 = Increment(x=w1667) -> (x+1=w1664:i32)
                  }
                  frame True {
                    # "Reset Frames\nProcessed Count"
                    # "SWEEP SEARCH - Startup"
                    # "Multiple New Step\nby Step SIze"
                    # "F = CCW\nT = CW"
                    # "Last Direction"
                    # "Min Step"
                    # "add 10 in case\nactual position\nis lower than GP"
                    # "Set New Step #"
                    # "Choose Direction"
                    # "Nearest step"
                    # "Adjust Actual Posiiton\n to pre-determiend steps"
                    # "Move Servo 1 \"Step\" to\nSearch"
                    n597 = Add(x=5, y=w1678) -> (x+y=w1684:i32)
                    n598 = Quotient & Remainder(x=w1684, y=w1676) -> (floor(x/y)=w1682:i32)  [unwired: 1 out]
                    n599 = To Byte Integer(number=w1682) -> (8bit integer=w1673:i8)
                    n600 = Less?(x=w1673, y=1) -> (x < y?=w1679:bool)
                    n601 = case shown="False" w1679 {
                      tunnel: w1673 -> [w1695 w1703]
                      tunnel: [w1697 FALSE] -> w1669
                      tunnel: [w1696 w1703] -> w1681
                      tunnel: w1675 -> [w1694 _]
                      tunnel: w1676 -> [w1692 _]
                      frame False {
                        # "Max Step"
                        # "# of steps\nminus 1"
                        n602 = Divide(x=1024, y=w1692) -> (x/y=w1689:dbl)
                        n603 = To Unsigned Byte Integer(number=w1689) -> (unsigned 8bit integer=w1690:u8)
                        n604 = Greater Or Equal?(x=w1695, y=w1690) -> (x >= y?=w1691:bool)
                        n605 = case shown="True" w1691 {
                          tunnel: [w1698 TRUE] -> w1697
                          tunnel: [w1699 w1700] -> w1696
                          tunnel: w1695 -> [w1699 w1700]
                          tunnel: w1694 -> [w1698 _]
                          frame False {
                            # "No Need to\nChange Direction"
                          }
                          frame True {
                            # "T"
                            # "Move CW"
                          }
                        }
                      }
                      frame True {
                        # "F"
                        # "Move CCW"
                      }
                    }
                    n606 = case shown="True" w1669 {
                      tunnel: w1681 -> [w1686 w1687]
                      tunnel: [w1685 w1688] -> w1677
                      frame False {
                        # "CCW\n+1"
                        n607 = Increment(x=w1686) -> (x+1=w1685:i8)
                      }
                      frame True {
                        # "CW\n-1"
                        n608 = Decrement(x=w1687) -> (x-1=w1688:i8)
                      }
                    }
                    n609 = Multiply(x=w1677, y=w1676) -> (x*y=w1674:u16)
                    n610 = To Unsigned Word Integer(number=w1674) -> (unsigned 16bit integer=w1672:u16)
                  }
                }
                n611 = local read "Track Angle Valid - Left"() -> (w1635:bool)
                n612 = local read "Image Lock - Left"() -> (w1634:bool)
                n613 = Or(x=w1634, y=w1635) -> (x .or. y?=w1633:bool)
                n614 = case shown="False" w1640 {
                  tunnel: [w1653 w1663] -> w1641
                  tunnel: w1642 -> [w1654 _]
                  tunnel: [w1655 enum16{"Generic Sweep", "Recovery Search"}."Generic Sweep"] -> w1638
                  tunnel: [w1652 w1663] -> w1639
                  tunnel: w1633 -> [w1651 _]
                  frame False {
                    # "Is other servo tracking?"
                    n615 = case shown="True" w1651 {
                      tunnel: [enum16{"Generic Sweep", "Recovery Search"}."Generic Sweep" enum16{"Generic Sweep", "Recovery Search"}."Recovery Search"] -> w1655
                      tunnel: w1654 -> [w1658 _]
                      tunnel: [w1658 FALSE] -> w1653
                      tunnel: [FALSE TRUE] -> w1652
                      frame False {
                        # "Stay in Sweep"
                      }
                      frame True {
                        # "G o to Recovery Search  State"
                      }
                    }
                  }
                  frame True {
                    w1663 = FALSE
                    # "Override Move Servo\nCommand bc an Angle Was Found\nduring this Step"
                    # "Stay In Sweep\nLet Main State Machine transition\ninto Tracking"
                  }
                }
              }
            }
            n616 = Increment(x=w1523) -> (x+1=w1502:i32)
            n617 = case shown="True" w1515 {
              tunnel: w1502 -> [w1538 _]
              tunnel: [w1538 0] -> w1516
              frame False {
              }
              frame True {
              }
            }
            n618 = case shown="False" w1503 {
              tunnel: [T2."Recovery Mode" ("Next Main State") T2."Tracking" ("Next Main State")] -> w1514
              frame False {
              }
              frame True {
              }
            }
          }
        }
        "Current Move Delta - L 2" <- w1229
        n619 = Less?(x=w1256, y=w1255) -> (x < y?=w1254:bool)
        n620 = local write "New Data  Flag\nRight Servo"(FALSE) -> ()
        n621 = Select(t=w1255, s=w1254, f=w1256) -> (s? t:f=w1251:u16)
        n622 = Greater?(x=w1251, y=w1252) -> (0:w1253:bool)
        n623 = Select(t=w1252, s=w1253, f=w1251) -> (s? t:f=w1250:u16)
      }
    }
    "Next Main State - Right" <- w1114
    "Next Tracking State - Right" <- w1109
    "Next Recovery State - Right" <- w1110
    n624 = case shown="True" w1140 {
      tunnel: [w1715 w1753] -> w1187
      tunnel: [w1709 w1752] -> w1186
      tunnel: w1185 -> [w1710 w1751]
      tunnel: w1184 -> [_ w1750]
      tunnel: "Track Angle Valid - Left" -> [_ w1749]
      tunnel: w1182 -> [_ w1748]
      tunnel: w1181 -> [w1715 w1747]
      tunnel: "Mounting Offset - Left" -> [_ w1746]
      tunnel: w1179 -> [w1706 w1745]
      tunnel: w1178 -> [_ w1744]
      tunnel: w1177 -> [w1707 w1743]
      tunnel: w1176 -> [_ w1742]
      tunnel: w1175 -> [_ w1741]
      tunnel: w1174 -> [_ w1740]
      tunnel: "Middle Beacon\nCoordinates" -> [_ w1739]
      tunnel: w1172 -> [w1705 w1738]
      tunnel: w1171 -> [w1704 w1737]
      tunnel: w1170 -> [w1708 w1736]
      tunnel: w1169 -> [_ w1735]
      tunnel: w1168 -> [_ w1734]
      tunnel: w1167 -> [_ w1733]
      tunnel: [0 w1732] -> w1161
      tunnel: [w1710 w1731] -> w1160
      tunnel: [w1709 w1730] -> w1159
      tunnel: [w1708 w1729] -> w1158
      tunnel: [w1704 w1728] -> w1157
      tunnel: [w1707 w1727] -> w1156
      tunnel: [w1705 w1726] -> w1155
      tunnel: w1153 -> [_ w1725]
      tunnel: [w1706 w1724] -> w1152
      tunnel: w1150 -> [_ w1723]
      tunnel: w1146 -> [w1713 w1722]
      tunnel: w1145 -> [w1712 w1721]
      tunnel: [w1713 w1720] -> w1144
      tunnel: [w1712 w1719] -> w1143
      tunnel: w1142 -> [w1711 w1718]
      tunnel: [w1711 w1717] -> w1141
      frame False {
        w1709 = FALSE
        # "Recovery Mode COunt"
        # "Frames Processed - L"
        # "Recovery Search move Count - L"
        # "Recovery Search Attempt Count- L"
        # "WAITING FOR NEW IMAGE, RETAIN ALL VALUES"
      }
      frame True {
        w1755 = u16 1023
        w1758 = u16 0
        # "New Tracking State"
        # "Tracking Timeout Count"
        # "Next Main State"
        # "Next Recovery State"
        # "Reset Respond"
        # "Search Direction"
        # "Recovery Count"
        # "Recovery Search move Count"
        # "Recovery Search Attempt Count"
        # "Frames Processed"
        # "Apply Floor/Ceiling to Goal Position"
        # "Current move Delta"
        # "Service Track Angle Flag"
        # "Move Servo"
        # "Goal Position"
        # "Go to Current State"
        n625 = case shown="\"Recovery Mode\"" w1751 {
          tunnel: w1747 -> [w1777 w1854 w2032]
          tunnel: w1748 -> [_ w1856 _]
          tunnel: w1733 -> [w1776 _ w2027]
          tunnel: w1745 -> [w1775 w1836 w2021]
          tunnel: [w1774 w1852 w2031] -> w1759
          tunnel: [w1772 w1853 w2030] -> w1752
          tunnel: w1749 -> [w1770 w1847 w2008]
          tunnel: [w1769 w1849 w2017] -> w1731
          tunnel: w1750 -> [w1768 w1848 w2007]
          tunnel: w1746 -> [_ w1857 w2028]
          tunnel: w1735 -> [_ w1855 _]
          tunnel: [w1762 w1851 w2012] -> w1732
          tunnel: w1734 -> [_ w1850 _]
          tunnel: w1743 -> [w1767 _ w2022]
          tunnel: [enum16{"Generic Sweep", "Recovery Search"}."Recovery Search" enum16{"Generic Sweep", "Recovery Search"}."Recovery Search" w2029] -> w1717
          tunnel: w1738 -> [_ _ w2026]
          tunnel: w1718 -> [_ _ w2009]
          tunnel: w1744 -> [_ w1833 w2038]
          tunnel: w1725 -> [_ w1838 w2033]
          tunnel: w1740 -> [_ w1840 w2035]
          tunnel: w1741 -> [_ w1841 w2036]
          tunnel: w1742 -> [_ w1842 w2037]
          tunnel: w1739 -> [_ w1839 w2034]
          tunnel: [FALSE w1835 w2010] -> w1730
          tunnel: w1723 -> [w1766 _ w2020]
          tunnel: [w1762 w1830 w2019] -> w1726
          tunnel: [w1762 w1830 w2025] -> w1729
          tunnel: [w1762 w1830 w2024] -> w1728
          tunnel: [w1765 w1831 w2023] -> w1727
          tunnel: w1737 -> [_ _ w2015]
          tunnel: w1736 -> [_ _ w2014]
          tunnel: [w1763 w1836 w2013] -> w1724
          tunnel: w1722 -> [_ w1846 _]
          tunnel: [w1762 w1837 w2012] -> w1720
          tunnel: w1721 -> [_ w1843 _]
          tunnel: [enum16{"Track", "Reactive Predict", ""}."Track" ("Initial Tracking State - Right") w1834 enum16{"Track", "Reactive Predict", ""}."Track" ("Initial Tracking State - Right")] -> w1719
          frame "Start Up Search", Default {
            w1762 = u16 0
            # "Search Direction"
            # "Wait for 'x' Images to be Processed\nBefore Going to Next Step"
            # "Next Main State"
            # "New Goal Position"
            # "Move Servo"
            # "Choose Next State"
            # "Frames Processed Count"
            n626 = Greater Or Equal?(x=w1767, y=w1766) -> (x >= y?=w1773:bool)
            n627 = case shown="True" w1773 {
              tunnel: w1777 -> [w1792 w1804]
              tunnel: w1776 -> [_ w1802]
              tunnel: w1775 -> [w1791 w1801]
              tunnel: [w1792 w1798] -> w1774
              tunnel: [w1790 0] -> w1765
              tunnel: [FALSE TRUE] -> w1771
              tunnel: w1767 -> [w1793 _]
              tunnel: [w1791 w1795] -> w1763
              frame False {
                # "Increase Frames\nProcessed Count"
                n628 = Increment(x=w1793) -> (x+1=w1790:i32)
              }
              frame True {
                # "Reset Frames\nProcessed Count"
                # "SWEEP SEARCH - Startup"
                # "Multiple New Step\nby Step SIze"
                # "F = CCW\nT = CW"
                # "Last Direction"
                # "Min Step"
                # "add 10 in case\nactual position\nis lower than GP"
                # "Set New Step #"
                # "Choose Direction"
                # "Nearest step"
                # "Adjust Actual Posiiton\n to pre-determiend steps"
                # "Move Servo 1 \"Step\" to\nSearch"
                n629 = Add(x=3, y=w1804) -> (x+y=w1810:i32)
                n630 = Quotient & Remainder(x=w1810, y=w1802) -> (floor(x/y)=w1808:i32)  [unwired: 1 out]
                n631 = To Byte Integer(number=w1808) -> (8bit integer=w1799:i8)
                n632 = Less?(x=w1799, y=1) -> (x < y?=w1805:bool)
                n633 = case shown="False" w1805 {
                  tunnel: w1799 -> [w1821 w1829]
                  tunnel: [w1823 FALSE] -> w1795
                  tunnel: [w1822 w1829] -> w1807
                  tunnel: w1801 -> [w1820 _]
                  tunnel: w1802 -> [w1818 _]
                  frame False {
                    # "Max Step"
                    # "# of steps\nminus 1"
                    n634 = Divide(x=1024, y=w1818) -> (x/y=w1815:dbl)
                    n635 = To Unsigned Byte Integer(number=w1815) -> (unsigned 8bit integer=w1816:u8)
                    n636 = Greater Or Equal?(x=w1821, y=w1816) -> (x >= y?=w1817:bool)
                    n637 = case shown="True" w1817 {
                      tunnel: [w1824 TRUE] -> w1823
                      tunnel: [w1825 w1826] -> w1822
                      tunnel: w1821 -> [w1825 w1826]
                      tunnel: w1820 -> [w1824 _]
                      frame False {
                        # "No Need to\nChange Direction"
                      }
                      frame True {
                        # "T"
                        # "Move CW"
                      }
                    }
                  }
                  frame True {
                    # "F"
                    # "Move CCW"
                  }
                }
                n638 = case shown="False" w1795 {
                  tunnel: w1807 -> [w1812 w1813]
                  tunnel: [w1811 w1814] -> w1803
                  frame False {
                    # "CCW\n+1"
                    n639 = Increment(x=w1812) -> (x+1=w1811:i8)
                  }
                  frame True {
                    # "CW\n-1"
                    n640 = Decrement(x=w1813) -> (x-1=w1814:i8)
                  }
                }
                n641 = Multiply(x=w1803, y=w1802) -> (x*y=w1800:u16)
                n642 = To Unsigned Word Integer(number=w1800) -> (unsigned 16bit integer=w1798:u16)
              }
            }
            n643 = case shown="False" w1770 {
              tunnel: [w1781 FALSE] -> w1772
              tunnel: w1771 -> [w1781 _]
              tunnel: [w1782 w1787] -> w1769
              tunnel: w1768 -> [_ w1785]
              frame False {
                # "Check other Servo\nStay in Startup  State"
                n644 = local read "Track Angle Valid  - Right"() -> (w1778:bool)
                n645 = local read "Image Lock - Right"() -> (w1779:bool)
                n646 = Or(x=w1778, y=w1779) -> (x .or. y?=w1780:bool)
                n647 = case shown="True" w1780 {
                  tunnel: [T2."Start Up Search" ("Next Main State") T2."Recovery Mode" ("Next Main State")] -> w1782
                  frame False {
                  }
                  frame True {
                  }
                }
              }
              frame True {
                # "Override Move Servo\nCommand bc an Angle Was Found\nduring this Step"
                # "Transition to Tracking State When\nImage Processing has Locked"
                n648 = case shown="False" w1785 {
                  tunnel: [T2."Start Up Search" ("Next Main State") T2."Tracking" ("Next Main State")] -> w1787
                  frame False {
                  }
                  frame True {
                  }
                }
              }
            }
          }
          frame "Tracking" {
            w1830 = 0
            # "Frames Processed Count"
            # "Image Lock - L"
            # "Track Angle Valid"
            # "Tracking Angle"
            # "Tracking Timeout Count"
            # "Max ove delta"
            # "Move delta threshold"
            # "mount offset"
            # "Current Position"
            # "Move Respond"
            # "Trackin Timeout count"
            # "Move Servo"
            # "delta"
            # "GP"
            # "Reset Move Respond"
            # "New Tracking State"
            # "Delta Move Sum"
            # "Choose Next State"
            n649 = case shown="\"Track\", Default" w1843 {
              tunnel: w1857 -> [w1875 _]
              tunnel: w1856 -> [w1874 _]
              tunnel: w1855 -> [w1873 _]
              tunnel: w1854 -> [w1872 w1930]
              tunnel: [w1871 w1928] -> w1853
              tunnel: [w1870 w1936] -> w1852
              tunnel: [w1869 0] -> w1851
              tunnel: w1850 -> [w1868 _]
              tunnel: w1848 -> [w1867 w1920]
              tunnel: w1847 -> [w1866 w1923]
              tunnel: w1846 -> [w1865 w1925]
              tunnel: w1842 -> [_ w1935]
              tunnel: w1841 -> [_ w1934]
              tunnel: w1840 -> [_ w1933]
              tunnel: w1839 -> [_ w1932]
              tunnel: w1833 -> [_ w1931]
              tunnel: w1838 -> [_ w1929]
              tunnel: [TRUE w1926] -> w1835
              tunnel: [w1862 w1924] -> w1837
              tunnel: [w1860 w1922] -> w1834
              tunnel: [0 0] -> w1831
              frame "Track", Default {
                # "Reset"
                # "Tracking Timeout"
                # "Move Delta"
                # "Goal Position"
                # "Tracking Move"
                # "Move Servo"
                # "Only Consider Tracking Angle\n\nIF\n\nImage Locked        == T\nTrack Angle Flag   == T"
                n650 = And(x=w1867, y=w1866) -> (x .and. y?=w1859:bool)
                n651 = case shown="True" w1859 {
                  tunnel: w1875 -> [_ w1881]
                  tunnel: w1874 -> [_ w1899]
                  tunnel: w1873 -> [_ w1896]
                  tunnel: w1872 -> [w1878 w1886]
                  tunnel: [w1878 w1895] -> w1870
                  tunnel: [w1880 w1894] -> w1871
                  tunnel: [w1880 w1893] -> _
                  tunnel: [u16 0 w1892] -> w1869
                  tunnel: w1868 -> [_ w1888]
                  tunnel: w1865 -> [w1877 _]
                  tunnel: [w1876 0] -> w1862
                  frame False {
                    w1880 = FALSE
                    # "Increment timeout"
                    n652 = Increment(x=w1877) -> (x+1=w1876:i32)
                  }
                  frame True {
                    # "Convert Track Angle to UINT16"
                    # "1024/300"
                    # "Move to Tracking Angle \n\nif delta is greater than move servo threshold\nAND less than max move threshold"
                    n653 = Add(x=w1899, y=w1881) -> (x+y=w1902:sgl)
                    n654 = Add(x=w1902, y=sgl 60.0) -> (x+y=w1901:sgl)
                    n655 = Multiply(x=3.413333333333333, y=w1901) -> (x*y=w1882:dbl)
                    n656 = To Word Integer(number=w1886) -> (16bit integer=w1884:i16)
                    n657 = To Unsigned Word Integer(number=w1882) -> (unsigned 16bit integer=w1898:u16)
                    n658 = To Word Integer(number=w1882) -> (16bit integer=w1897:i16)
                    n659 = Subtract(x=w1897, y=w1884) -> (x-y=w1887:i16)
                    n660 = Absolute Value(x=w1887) -> (abs(x)=w1883:i16)
                    n661 = Greater Or Equal?(x=w1883, y=w1896) -> (x >= y?=w1890:bool)
                    n662 = Less Or Equal?(x=w1883, y=w1888) -> (x <= y?=w1889:bool)
                    n663 = And(x=w1890, y=w1889) -> (x .and. y?=w1891:bool)
                    n664 = case shown="True" w1891 {
                      tunnel: w1898 -> [_ w1910]
                      tunnel: [w1905 w1910] -> w1895
                      tunnel: [w1906 w1916] -> w1894
                      tunnel: [w1906 w1916] -> w1893
                      tunnel: w1886 -> [w1905 _]
                      tunnel: w1883 -> [_ w1915]
                      tunnel: [u16 0 w1915] -> w1892
                      tunnel: w1881 -> [_ w1909]
                      frame False {
                        w1906 = FALSE
                        # "Don't Move"
                      }
                      frame True {
                        w1916 = TRUE
                        # "45 DEG MOUNT OFFSET"
                        # "1024/300"
                        # "Current Delta"
                        # "Use new Track Angle"
                        n665 = Divide(x=w1910, y=3.413333333333333) -> (x/y=w1912:dbl)
                        n666 = Negate(x=w1909) -> (-x=w1908:sgl)
                        n667 = Subtract(x=w1912, y=sgl 60.0) -> (x-y=w1914:dbl)
                        n668 = Add(x=w1914, y=w1908) -> (x+y=w1907:dbl)
                        n669 = local write "Last Track Angle - L"(w1907) -> ()
                      }
                    }
                  }
                }
                n670 = local read "Timeout to \nEnable Reactive Predict"() -> (w1863:u16)
                n671 = Less?(x=w1862, y=w1863) -> (x < y?=w1861:bool)
                n672 = case shown="True" w1861 {
                  tunnel: [enum16{"Track", "Reactive Predict", ""}."Reactive Predict" ("Initial Tracking State - Right") enum16{"Track", "Reactive Predict", ""}."Track" ("Initial Tracking State - Right")] -> w1860
                  frame False {
                  }
                  frame True {
                  }
                }
              }
              frame "Reactive Predict" {
                # "Choose New\nTracking State"
                n673 = Or(x=w1920, y=w1923) -> (x .or. y?=w1919:bool)
                n674 = case shown="False" w1919 {
                  tunnel: [w1949 w2001] -> w1936
                  tunnel: w1935 -> [w1948 _]
                  tunnel: w1934 -> [w1947 _]
                  tunnel: w1933 -> [w1946 _]
                  tunnel: w1932 -> [w1945 _]
                  tunnel: w1931 -> [w1944 _]
                  tunnel: w1929 -> [w1943 _]
                  tunnel: [w1942 w2000] -> w1928
                  tunnel: [w1941 w2000] -> w1926
                  tunnel: w1925 -> [w1940 _]
                  tunnel: [w1939 0] -> w1924
                  tunnel: [enum16{"Track", "Reactive Predict", ""}."Reactive Predict" ("Initial Tracking State - Right") enum16{"Track", "Reactive Predict", ""}."Track" ("Initial Tracking State - Right")] -> w1922
                  tunnel: w1930 -> [w1937 w2001]
                  frame False {
                    # "Stay in Reactive State"
                    # "Increment Track Timeout"
                    # "Move Respond Flag"
                    n675 = Increment(x=w1940) -> (x+1=w1939:i32)
                    n676 = case shown="True" w1944 {
                      tunnel: w1948 -> [_ w1964]
                      tunnel: w1947 -> [_ w1963]
                      tunnel: w1946 -> [_ w1962]
                      tunnel: w1945 -> [_ w1961]
                      tunnel: w1943 -> [_ w1958]
                      tunnel: [w1950 w1954] -> w1949
                      tunnel: [w1951 w1953] -> w1942
                      tunnel: [w1951 w1953] -> w1941
                      tunnel: w1937 -> [w1950 w1952]
                      frame False {
                        w1951 = FALSE
                        # "Reset Move Respond = F"
                        # "Move Servo = F"
                      }
                      frame True {
                        w1953 = TRUE
                        # "Position Lock"
                        # "Current Servo\nPosition"
                        # "Reset Move\nRespond = T"
                        # "Move Servo = T"
                        # "Apply Direction \nto Offset (delta sum)"
                        # "Check Last Known Position of Robot"
                        n677 = case shown="True" w1964 {
                          tunnel: w1963 -> [_ w1992]
                          tunnel: w1962 -> [_ w1967]
                          tunnel: w1961 -> [_ w1968]
                          tunnel: [sgl 1.0 ("y") w1966] -> w1960
                          frame False {
                            # "No Position Data Available"
                            # "Default is to move\nSame Direction as other\nServo"
                          }
                          frame True {
                            w1973 = sgl 1.0 ("y")
                            # "Use previous position/orientation to Guess Which Direction to Move Servo"
                            # "Choose Search Direction"
                            # "\"Perpendicular \nThreshold\""
                            # "If Orientation is\n ~Perpendicular -> Start Search\n in Opposite Direction of Other"
                            # "****add 90 until orientation angle is fixed"
                            # "Last Orientation"
                            # "Convert to Rad"
                            # "Avoid Divide by 0"
                            # "-1/m"
                            # "Calculate Normal Line to \nLast Robot Position\nfrom Center Beacon"
                            # "last Position \nCoordinates"
                            n678 = Unbundle(w1992) -> ("X"=w1972:sgl, "Y"=w1971:sgl)
                            n679 = Unbundle(w1968) -> ("X"=w1970:sgl, "Y"=w1969:sgl)
                            n680 = Subtract(x=w1971, y=w1969) -> (x-y=w1988:sgl)
                            n681 = Subtract(x=w1972, y=w1970) -> (x-y=w1986:sgl)
                            n682 = Equal To 0?(x=w1986) -> (x = 0?=w1987:bool)
                            n683 = case shown="False" w1987 {
                              tunnel: w1988 -> [w1995 _]
                              tunnel: w1986 -> [w1994 _]
                              tunnel: [w1993 1000000000000000.0] -> w1985
                              frame False {
                                n684 = Divide(x=w1995, y=w1994) -> (x/y=w1993:sgl)
                              }
                              frame True {
                              }
                            }
                            n685 = Equal To 0?(x=w1985) -> (x = 0?=w1990:bool)
                            n686 = case shown="False" w1990 {
                              tunnel: [w1997 1e-08] -> w1989
                              tunnel: w1985 -> [w1997 _]
                              frame False {
                              }
                              frame True {
                                # "Can't have infinit slope"
                              }
                            }
                            n687 = Divide(x=-1.0, y=w1989) -> (x/y=w1984:dbl)
                            n688 = Inverse Tangent(1:w1984) -> (0:w1982:dbl)
                            n689 = expression code="(x/pi)*180.0" "radians to degrees"(w1982) -> (w1983:dbl)
                            n690 = To Single Precision Float(number=w1983) -> (single precision float=w1980:sgl)
                            n691 = Add(x=w1967, y=sgl 90.0) -> (x+y=w1979:sgl)
                            n692 = Subtract(x=w1980, y=w1979) -> (x-y=w1978:sgl)
                            n693 = Absolute Value(x=w1978) -> (abs(x)=w1977:sgl)
                            n694 = Less Or Equal?(x=w1977, y=sgl 10.0) -> (x <= y?=w1975:bool)
                            n695 = Negate(x=w1973) -> (-x=w1974:sgl)
                            n696 = Select(t=w1974, s=w1975, f=w1973) -> (s? t:f=w1966:sgl)
                          }
                        }
                        n697 = To Word Integer(number=w1960) -> (16bit integer=w1959:i16)
                        n698 = Multiply(x=w1959, y=w1958) -> (x*y=w1957:i32)
                        n699 = To Word Integer(number=w1952) -> (16bit integer=w1956:i16)
                        n700 = Add(x=w1957, y=w1956) -> (x+y=w1955:i32)
                        n701 = To Unsigned Word Integer(number=w1955) -> (unsigned 16bit integer=w1954:u16)
                      }
                    }
                  }
                  frame True {
                    w2000 = TRUE
                    # "Go Directly to Track State"
                  }
                }
              }
            }
            n702 = local read "Tracking Timeout\nThreshold"() -> (w1844:i32)
            n703 = Less?(x=w1837, y=w1844) -> (x < y?=w1845:bool)
            n704 = case shown="False" w1845 {
              tunnel: [T2."Recovery Mode" ("Next Main State") T2."Tracking" ("Next Main State")] -> w1849
              frame False {
              }
              frame True {
              }
            }
          }
          frame "Recovery Mode" {
            w2012 = u16 0
            # "***Compltetly resets as of R17, used to just reset to \"Max Recovery Count - 1\""
            # "Increment Recoveyr Mode Count"
            # "Frames Processed"
            # "Choose Next Main State"
            # "Reset recovery count"
            # "Recovery move\nCount"
            # "Recovery Search\nAttempt count"
            # "Move Servo = T"
            # "delta move sum"
            # "Robot Position Valid"
            n705 = local read "Image Lock - Right"() -> (w2016:bool)
            n706 = Or(x=w2007, y=w2008) -> (x .or. y?=w2006:bool)
            n707 = case shown="\"Recovery Search\"" w2009 {
              tunnel: w2038 -> [_ _]
              tunnel: w2037 -> [_ _]
              tunnel: w2036 -> [_ _]
              tunnel: w2035 -> [_ _]
              tunnel: w2034 -> [_ _]
              tunnel: w2033 -> [_ _]
              tunnel: w2032 -> [w2066 w2152]
              tunnel: [w2058 w2150] -> w2031
              tunnel: [w2055 w2144] -> w2030
              tunnel: [FALSE FALSE] -> w2010
              tunnel: [w2060 w2141] -> w2029
              tunnel: w2026 -> [w2064 _]
              tunnel: w2028 -> [w2067 _]
              tunnel: w2027 -> [w2065 w2147]
              tunnel: [w2057 w2140] -> w2024
              tunnel: [w2056 w2140] -> w2025
              tunnel: w2016 -> [w2054 _]
              tunnel: [w2045 w2151] -> w2023
              tunnel: w2022 -> [w2043 w2135]
              tunnel: w2021 -> [w2048 w2148]
              tunnel: w2020 -> [w2044 w2146]
              tunnel: w2007 -> [_ _]
              tunnel: w2008 -> [_ w2143]
              tunnel: [FALSE w2142] -> w2018
              tunnel: w2015 -> [w2052 _]
              tunnel: w2014 -> [w2051 _]
              tunnel: [w2048 w2139] -> w2013
              frame "Recovery Search" {
                # "Wait for 2 Images to be Processed\nBefore Going to Next Step"
                # "Choose Next Reovery State"
                # "Recovery Search \nAttempt Count"
                # "Move Servo"
                # "Goal Position"
                # "Recovery Search\nmove Count"
                # "Attempt Recovery Search if Other Servo has Valid Angle"
                n708 = local read "Last Track Angle - R"() -> (w2047:sgl)
                n709 = Greater Or Equal?(x=w2043, y=w2044) -> (x >= y?=w2046:bool)
                n710 = case shown="True" w2046 {
                  tunnel: w2067 -> [_ w2087]
                  tunnel: [w2072 w2086] -> w2056
                  tunnel: w2066 -> [w2075 w2085]
                  tunnel: w2065 -> [_ w2084]
                  tunnel: [w2073 w2083] -> w2057
                  tunnel: [w2075 w2082] -> w2058
                  tunnel: [FALSE w2081] -> w2055
                  tunnel: w2052 -> [w2073 w2080]
                  tunnel: w2051 -> [w2072 w2079]
                  tunnel: w2054 -> [_ w2078]
                  tunnel: w2047 -> [_ w2077]
                  tunnel: [w2070 0 ("Frames Processed\nCount - in")] -> w2045
                  tunnel: w2043 -> [w2071 _]
                  frame False {
                    # "Increment Frames Processed"
                    # "WAIT"
                    n711 = Increment(x=w2071) -> (x+1=w2070:i32)
                  }
                  frame True {
                    n712 = case shown="True" w2078 {
                      tunnel: w2077 -> [_ w2100]
                      tunnel: w2080 -> [w2088 w2096]
                      tunnel: w2087 -> [_ w2101]
                      tunnel: [w2091 w2099] -> w2082
                      tunnel: [w2089 w2098] -> w2086
                      tunnel: w2079 -> [w2089 w2097]
                      tunnel: w2085 -> [w2091 w2095]
                      tunnel: w2084 -> [_ w2094]
                      tunnel: [FALSE TRUE] -> w2081
                      tunnel: [w2088 w2092] -> w2083
                      frame False {
                        # "Don't Move bc Other Servo Doesn't Have Image Lock"
                      }
                      frame True {
                        # "Move Servo = T"
                        n713 = Greater Than 0?(x=w2096) -> (x > 0?=w2102:bool)
                        n714 = case shown="False" w2102 {
                          tunnel: w2101 -> [w2109 _]
                          tunnel: w2100 -> [w2103 _]
                          tunnel: [w2108 w2119] -> w2099
                          tunnel: [w2106 w2125] -> w2098
                          tunnel: w2097 -> [w2107 w2125]
                          tunnel: w2096 -> [w2105 w2122]
                          tunnel: [w2104 w2124] -> w2092
                          tunnel: w2095 -> [_ w2120]
                          tunnel: w2094 -> [_ w2117]
                          frame False {
                            # "Increment move count to transition\nto Pan mode"
                            # "Increment Recovery Search Attempt Count"
                            # "1024/300"
                            # "Move Parallel to Other Servo"
                            n715 = Increment(x=w2107) -> (x+1=w2106:i32)
                            n716 = Add(x=w2103, y=w2109) -> (x+y=w2115:sgl)
                            n717 = Add(x=w2115, y=sgl 60.0) -> (x+y=w2114:sgl)
                            n718 = Multiply(x=3.413333333333333, y=w2114) -> (x*y=w2112:dbl)
                            n719 = Add(x=0.5, y=w2112) -> (x+y=w2110:dbl)
                            n720 = To Unsigned Word Integer(number=w2110) -> (unsigned 16bit integer=w2108:u16)
                            n721 = Increment(x=w2105) -> (x+1=w2104:i32)
                          }
                          frame True {
                            # "Apply Direction"
                            # "Step SIze"
                            # "Current Position"
                            # "Attempt to Pan in Steps Towards other Servo"
                            # "Could be same or function of \nregular search step size"
                            # "Max # of Pan\nMoves"
                            # "Pan Towards Other Servo"
                            n722 = Greater Or Equal?(x=w2122, y=u16 20) -> (x >= y?=w2123:bool)
                            n723 = case shown="False" w2123 {
                              tunnel: w2122 -> [w2133 _]
                              tunnel: [w2132 u16 0] -> w2124
                              frame False {
                                # "Increment Pan Count"
                                n724 = Increment(x=w2133) -> (x+1=w2132:i32)
                              }
                              frame True {
                                # "Reset move count"
                              }
                            }
                            n725 = local read "Recovery Search\nDirection - L"() -> (w2118:bool)
                            n726 = case shown="False" w2118 {
                              tunnel: w2120 -> [w2127 w2131]
                              tunnel: w2117 -> [w2128 w2130]
                              tunnel: [w2126 w2129] -> w2119
                              frame False {
                                # "CCW"
                                n727 = Add(x=w2127, y=w2128) -> (x+y=w2126:u16)
                              }
                              frame True {
                                # "CW"
                                n728 = Subtract(x=w2131, y=w2130) -> (x-y=w2129:u16)
                              }
                            }
                          }
                        }
                      }
                    }
                  }
                }
                n729 = local read "Max Recovery Count\n(Recovery Search)"() -> (w2049:u16)
                n730 = local read "Max Recovery\nSearch Attempts"() -> (w2050:u16)
                n731 = Less Or Equal?(x=w2056, y=w2050) -> (x <= y?=w2062:bool)
                n732 = Less Or Equal?(x=w2064, y=w2049) -> (x <= y?=w2063:bool)
                n733 = And(x=w2062, y=w2063) -> (x .and. y?=w2061:bool)
                n734 = case shown="True" w2061 {
                  tunnel: [enum16{"Generic Sweep", "Recovery Search"}."Generic Sweep" enum16{"Generic Sweep", "Recovery Search"}."Recovery Search"] -> w2060
                  frame False {
                  }
                  frame True {
                  }
                }
              }
              frame "Generic Sweep" {
                w2140 = u16 0
                # "Angle Valid?"
                # "Choose Next Recovery State"
                # "Wait for 2 Images to be Processed\nBefore Going to Next Step"
                # "New Goal Position"
                # "Move Servo"
                # "Frames Processed Count"
                n735 = Greater Or Equal?(x=w2135, y=w2146) -> (x >= y?=w2153:bool)
                n736 = case shown="True" w2153 {
                  tunnel: w2152 -> [w2169 w2181]
                  tunnel: w2147 -> [_ w2179]
                  tunnel: w2148 -> [w2168 w2178]
                  tunnel: [w2169 w2175] -> w2150
                  tunnel: [w2167 0] -> w2151
                  tunnel: [FALSE TRUE] -> w2145
                  tunnel: w2135 -> [w2170 _]
                  tunnel: [w2168 w2172] -> w2139
                  frame False {
                    # "Increment Frames Processed"
                    n737 = Increment(x=w2170) -> (x+1=w2167:i32)
                  }
                  frame True {
                    # "Reset Frames\nProcessed Count"
                    # "SWEEP SEARCH - Startup"
                    # "Multiple New Step\nby Step SIze"
                    # "F = CCW\nT = CW"
                    # "Last Direction"
                    # "Min Step"
                    # "add 10 in case\nactual position\nis lower than GP"
                    # "Set New Step #"
                    # "Choose Direction"
                    # "Nearest step"
                    # "Adjust Actual Posiiton\n to pre-determiend steps"
                    # "Move Servo 1 \"Step\" to\nSearch"
                    n738 = Add(x=5, y=w2181) -> (x+y=w2187:i32)
                    n739 = Quotient & Remainder(x=w2187, y=w2179) -> (floor(x/y)=w2185:i32)  [unwired: 1 out]
                    n740 = To Byte Integer(number=w2185) -> (8bit integer=w2176:i8)
                    n741 = Less?(x=w2176, y=1) -> (x < y?=w2182:bool)
                    n742 = case shown="False" w2182 {
                      tunnel: w2176 -> [w2198 w2206]
                      tunnel: [w2200 FALSE] -> w2172
                      tunnel: [w2199 w2206] -> w2184
                      tunnel: w2178 -> [w2197 _]
                      tunnel: w2179 -> [w2195 _]
                      frame False {
                        # "Max Step"
                        # "# of steps\nminus 1"
                        n743 = Divide(x=1024, y=w2195) -> (x/y=w2192:dbl)
                        n744 = To Unsigned Byte Integer(number=w2192) -> (unsigned 8bit integer=w2193:u8)
                        n745 = Greater Or Equal?(x=w2198, y=w2193) -> (x >= y?=w2194:bool)
                        n746 = case shown="True" w2194 {
                          tunnel: [w2201 TRUE] -> w2200
                          tunnel: [w2202 w2203] -> w2199
                          tunnel: w2198 -> [w2202 w2203]
                          tunnel: w2197 -> [w2201 _]
                          frame False {
                            # "No Need to\nChange Direction"
                          }
                          frame True {
                            # "T"
                            # "Move CW"
                          }
                        }
                      }
                      frame True {
                        # "F"
                        # "Move CCW"
                      }
                    }
                    n747 = case shown="True" w2172 {
                      tunnel: w2184 -> [w2189 w2190]
                      tunnel: [w2188 w2191] -> w2180
                      frame False {
                        # "CCW\n+1"
                        n748 = Increment(x=w2189) -> (x+1=w2188:i8)
                      }
                      frame True {
                        # "CW\n-1"
                        n749 = Decrement(x=w2190) -> (x-1=w2191:i8)
                      }
                    }
                    n750 = Multiply(x=w2180, y=w2179) -> (x*y=w2177:u16)
                    n751 = To Unsigned Word Integer(number=w2177) -> (unsigned 16bit integer=w2175:u16)
                  }
                }
                n752 = local read "Track Angle Valid  - Right"() -> (w2138:bool)
                n753 = local read "Image Lock - Right"() -> (w2137:bool)
                n754 = Or(x=w2137, y=w2138) -> (x .or. y?=w2136:bool)
                n755 = case shown="False" w2143 {
                  tunnel: [w2156 w2166] -> w2144
                  tunnel: w2145 -> [w2157 _]
                  tunnel: [w2158 enum16{"Generic Sweep", "Recovery Search"}."Generic Sweep"] -> w2141
                  tunnel: [w2155 w2166] -> w2142
                  tunnel: w2136 -> [w2154 _]
                  frame False {
                    # "Is other servo tracking?"
                    n756 = case shown="True" w2154 {
                      tunnel: [enum16{"Generic Sweep", "Recovery Search"}."Generic Sweep" enum16{"Generic Sweep", "Recovery Search"}."Recovery Search"] -> w2158
                      tunnel: w2157 -> [w2161 _]
                      tunnel: [w2161 FALSE] -> w2156
                      tunnel: [FALSE TRUE] -> w2155
                      frame False {
                        # "Stay in Sweep"
                      }
                      frame True {
                        # "G o to Recovery Search  State"
                      }
                    }
                  }
                  frame True {
                    w2166 = FALSE
                    # "Override Move Servo\nCommand bc an Angle Was Found\nduring this Step"
                    # "Stay In Sweep\nLet Main State Machine transition\ninto Tracking"
                  }
                }
              }
            }
            n757 = Increment(x=w2026) -> (x+1=w2005:i32)
            n758 = case shown="True" w2018 {
              tunnel: w2005 -> [w2041 _]
              tunnel: [w2041 0] -> w2019
              frame False {
              }
              frame True {
              }
            }
            n759 = case shown="False" w2006 {
              tunnel: [T2."Recovery Mode" ("Next Main State") T2."Tracking" ("Next Main State")] -> w2017
              frame False {
              }
              frame True {
              }
            }
          }
        }
        "Current Move Delta - L" <- w1732
        n760 = Less?(x=w1759, y=w1758) -> (x < y?=w1757:bool)
        n761 = local write "New Data  Flag\nLeft Servo"(FALSE) -> ()
        n762 = Select(t=w1758, s=w1757, f=w1759) -> (s? t:f=w1754:u16)
        n763 = Greater?(x=w1754, y=w1755) -> (0:w1756:bool)
        n764 = Select(t=w1755, s=w1756, f=w1754) -> (s? t:f=w1753:u16)
      }
    }
    "Next Main State - Left" <- w1160
    "Next Tracking State - Left" <- w1143
    "Next Recovery State - Left" <- w1141
    n765 = flat-sequence {
      tunnel: w1186 -> [w2213]
      tunnel: w1113 -> [w2212]
      tunnel: w1187 -> [w2215]
      tunnel: w1102 -> [w2214]
      tunnel: [w2213] -> w1200
      tunnel: [w2212] -> w1199
      tunnel: w1200 -> [w2221]
      tunnel: [w2220] -> w1195
      tunnel: [w2219] -> w1196
      tunnel: w1199 -> [w2218]
      frame #0 {
        # "Only Update GP if Moving Servo"
        n766 = case shown="True" w2213 {
          tunnel: w2215 -> [_ w2217]
          frame False {
          }
          frame True {
            # "Update Goal Position"
            n767 = local write "Servo Goal Position\n - Left"(w2217) -> ()
          }
        }
        n768 = case shown="True" w2212 {
          tunnel: w2214 -> [_ w2216]
          frame False {
          }
          frame True {
            # "New Direction"
            # "Update Goal Position"
            # "Update Direction"
            n769 = local write "Servo Goal Position\n - Right"(w2216) -> ()
          }
        }
      }
      frame #1 {
        # "Allow Comm Process to Take Down the Flag\nOnly Raise if not already in motion"
        n770 = local read "Servo Moving - R"() -> (w2226:bool)
        n771 = local read "Servo Moving - L"() -> (w2223:bool)
        n772 = local read "Move Servo - L"() -> (w2222:bool)
        n773 = local read "Move Servo - R"() -> (w2229:bool)
        n774 = Not(x=w2226) -> (.not. x?=w2228:bool)
        n775 = Not(x=w2223) -> (.not. x?=w2225:bool)
        n776 = And(x=w2218, y=w2228) -> (x .and. y?=w2227:bool)
        n777 = And(x=w2221, y=w2225) -> (x .and. y?=w2224:bool)
        n778 = case shown="True" w2227 {
          selector: w2227 -> [_ w2231]
          tunnel: [w2230 w2231] -> w2219
          tunnel: w2229 -> [w2230 _]
          frame False {
          }
          frame True {
          }
        }
        n779 = case shown="False" w2224 {
          selector: w2224 -> [_ w2233]
          tunnel: [w2232 w2233] -> w2220
          tunnel: w2222 -> [w2232 _]
          frame False {
          }
          frame True {
          }
        }
        n780 = local write "Move Servo - R"(w2219) -> ()
        n781 = local write "Move Servo - L"(w2220) -> ()
      }
    }
    n782 = local read "Current Main State - Right"() -> (w1165:T2)
    n783 = local read "Current Main State - Left"() -> (w1166:T2)
    n784 = Equal?(x=w1166, y=w1164) -> (x = y?=w1163:bool)
    n785 = Equal?(x=w1165, y=w1164) -> (x = y?=w1162:bool)
    n786 = And(x=w1163, y=w1195) -> (x .and. y?=w1191:bool)
    n787 = And(x=w1196, y=w1162) -> (x .and. y?=w1192:bool)
    n788 = And(x=w1163, y=w1162) -> (x .and. y?=w1190:bool)
    n789 = Exclusive Or(1:w1192, 2:w1191) -> (0:w1189:bool)
    n790 = case shown="True" w1189 {
      tunnel: [w2244 w2265] -> w1197
      tunnel: [w2245 w2264] -> w1193
      tunnel: w1112 -> [_ w2268]
      tunnel: w1153 -> [w2242 w2269]
      tunnel: w1116 -> [w2240 w2267]
      tunnel: [w2243 w2255] -> w1194
      tunnel: [w2241 w2254] -> w1198
      tunnel: w1161 -> [_ w2266]
      tunnel: w1190 -> [w2239 _]
      tunnel: w1191 -> [_ w2265]
      tunnel: w1192 -> [_ w2264]
      frame False {
        n791 = case shown="False" w2239 {
          tunnel: [w2249 w2251] -> w2245
          tunnel: [w2248 w2251] -> w2244
          tunnel: [w2247 w2250] -> w2243
          tunnel: w2242 -> [w2247 _]
          tunnel: [w2246 w2250] -> w2241
          tunnel: w2240 -> [w2246 _]
          frame False {
            # "No Movement\nRetain All Values"
            n792 = local read "Move Respond - L"() -> (w2249:bool)
            n793 = local read "Move Respond - R"() -> (w2248:bool)
          }
          frame True {
            w2250 = i16 0
            w2251 = FALSE
            # "Reset Delta Move sum\nfor both"
            # "F"
            # "Both Moved,\nMake Flags False"
          }
        }
      }
      frame True {
        w2261 = 200 ("y")
        w2252 = -200 ("y")
        # "Add/Clear Sum for \nServo That didn't move"
        # "Update Moving Servo's  Delta Position"
        # "if one Servo Moves, other should \nmove too eventually,\nUsed in Search Process"
        # "Only 1 Servo is Moving Due to Tracking --> Update delta move sum"
        n794 = case shown="True" w2264 {
          tunnel: w2269 -> [_ w2277]
          tunnel: w2268 -> [_ w2276]
          tunnel: [i16 0 w2275] -> w2262
          frame False {
          }
          frame True {
            n795 = Add(x=w2277, y=w2276) -> (x+y=w2275:i32)
          }
        }
        n796 = case shown="True" w2265 {
          tunnel: w2267 -> [_ w2273]
          tunnel: w2266 -> [_ w2272]
          tunnel: [i16 0 w2271] -> w2259
          frame False {
          }
          frame True {
            n797 = Add(x=w2273, y=w2272) -> (x+y=w2271:i32)
          }
        }
        n798 = Greater?(x=w2262, y=w2261) -> (0:w2263:bool)
        n799 = Greater?(x=w2259, y=w2261) -> (0:w2260:bool)
        n800 = Select(t=w2261, s=w2260, f=w2259) -> (s? t:f=w2256:i32)
        n801 = Select(t=w2261, s=w2263, f=w2262) -> (s? t:f=w2257:i32)
        n802 = Greater?(x=w2257, y=w2252) -> (0:w2253:bool)
        n803 = Greater?(x=w2256, y=w2252) -> (0:w2258:bool)
        n804 = Select(t=w2256, s=w2258, f=w2252) -> (s? t:f=w2254:i32)
        n805 = Select(t=w2257, s=w2253, f=w2252) -> (s? t:f=w2255:i32)
      }
    }
    n806 = case shown="True" w1108 {
      selector: w1108 -> [_ w2211]
      tunnel: [w2208 w2210] -> w1148
      tunnel: [w2207 i16 0] -> w1149
      tunnel: w1197 -> [w2208 _]
      tunnel: w1198 -> [w2207 _]
      frame False {
      }
      frame True {
        n807 = Not(x=w2211) -> (.not. x?=w2210:bool)
      }
    }
    "Move Respond - R" <- w1148
    "deltaMoveServo\n- R" <- w1149
    n808 = case shown="False" w1159 {
      selector: w1159 -> [_ w2238]
      tunnel: [w2235 w2237] -> w1151
      tunnel: [w2234 i16 0] -> w1154
      tunnel: w1193 -> [w2235 _]
      tunnel: w1194 -> [w2234 _]
      frame False {
      }
      frame True {
        n809 = Not(x=w2238) -> (.not. x?=w2237:bool)
      }
    }
    "Move Respond - L" <- w1151
    "deltaMoveServo\n- L" <- w1154
    "Current Main State - Left" <- w1185
    "Frames Processed\nCount - in -L" <- w1177
    "Recovery Mode Count - in Left" <- w1172
    "Recovery Search\nmove Count - in - L" <- w1171
    "Recovery Search\nAttempt Count - in - L" <- w1170
    "Current Main State - Right" <- w1139
    "Frames Processed\nCount - in Right" <- w1122
    "Recovery Search\nmove Count - Right" <- w1124
    "Recovery Search\nAttempt Count - Right" <- w1123
    "Recovery Mode Count in Right" <- w1115
    "Tracking Timeout\nCount - L" <- w1146
    "Tracking Timeout\nCount - R" <- w1131
    "Current Tracking State - Left" <- w1145
    "Current Tracking State - Right 2" <- w1137
    "Current Recovery State - Right" <- w1138
    "Current Recovery State -L" <- w1142
  }
